vi "LS Durability Main (RT).vi"() -> ()   [LabVIEW 2013]
uses:
  Type Defs/App Config.ctl
  Type Defs/Controller Names.ctl
  SubVIs/Data Logger/Data Log Init.ctl
  Controls/Alarm Config.ctl
  Controls/Alarm Definition.ctl
  Controls/Alarm Profile Config.ctl
  Type Defs/Controller List.ctl
  Controls/Tank CMDs.ctl
  Controls/Controller Config.ctl
  Controls/Pump Data.ctl
  Controls/Tank Data.ctl
  Controls/HMI Cluster.ctl
  Controls/HMI Header.ctl
  Controls/HMI Tog Buttons.ctl
  Controls/HMI Mom Buttons.ctl
  Type Defs/LS Data.ctl
  Type Defs/Sequence States.ctl
  Controls/App Global Mode.ctl
  Controls/RPi HMI Mode.ctl
  Controls/Email Mode.ctl
  Type Defs/Pump Data Mode.ctl
  SubVIs/Watlow Modbus/Modbus Mode.ctl
  SubVIs/Watlow Modbus/Modbus Variable.ctl
  Controls/HMI Global Mode.ctl
  <vilib>/FPGAPlugInAG/sbRIO-9626/niLvFpga_Open_sbRIO-9626.vi
  <vilib>/Utility/error.llb/Error Cluster From Error Code.vi
  <vilib>/rvi/errors/niLvFpgaAdjustHostInterfaceError.vi
  <vilib>/Utility/file.llb/Write To Spreadsheet File (string).vi
  <vilib>/rvi/interface/nirviOpenFPGA/nirviOpenFPGA.xnode
  Controls/FPGA_Reference.ctl
  FPGA Bitfiles/LSDurability_Main.lvbitx
  <vilib>/rvi/interface/nirviReadWriteControl/nirviReadWriteControl.xnode
  <vilib>/Utility/config.llb/NI_LVConfig.lvlib
  Controls/Power Supply Global Mode.ctl
  SubVIs/Data Logger/Data Logger Mode.ctl
  SubVIs/Data Logger/Data Log Start.ctl
  <vilib>/rvi/errors/niLvFpgaMergeErrorWithErrorCode.vi
  NiFpgaLv.dll
panel:
  in  "pb.Run Profile":bool
  in  "Bank 2":T1={"7"=TRUE, "8"=TRUE, "9"=TRUE, "10"=TRUE, "11"=TRUE}
  in  "Bank 1":T2={"1"=TRUE, "2"=TRUE, "3"=TRUE, "4"=TRUE, "5"=TRUE} caption="Present"
  out "Email Alarms Disabled":bool
  out "Recording":bool
  in  "Disable Alarm Email":bool
  in  "Temp Tolerance":dbl=3.0 min=0.0 max=999999.0 step=1.0
  in  "Thermocouple":enum16{"2 TC/2 Tanks", "1 TC/1 Tank"}(ring)
  out "ADC Errors":i32
  in  "pb.Tare Pressure":bool
  in  "Data Log Enabled":bool=TRUE
  in  "RPMhyst":fxp<+,25,6>=1.0
  in  "pb.FuelChange":bool
  in  "Controller Type:":T3
  in  "Target Pressure:":dbl
  in  "Target Voltage:":dbl
  in  "Tank 1 Fuel Type:":string
  in  "Tank 2 Fuel Type:":string
  in  "Stagger Time (ms):":i32
  out "Cycles Completed:":u32=17
  in  "pb.Cycle Reset":bool
  in  "Serial Numbers":T4
  out "Read Inputs (ms)":u32
  out "Update Screen (ms)":u32
  out "Run Step (ms)":u32
  in  "Fuel Change Tab":enum32{"Page 1", "Page 2"}(tab)
  in  "pb.Fuel Change OK":bool
  in  "Reset Tab":enum32{"Page 1", "Page 2"}(tab)
  in  "pb.Reset OK":bool
  in  "pb.Reset Cancel":bool
  in  "Save As Tab":enum32{"Page 1", "Page 2"}(tab)
  in  "New Profile Name:":string
  in  "pb.Save As OK":bool
  in  "pb.Save As Cancel":bool
  in  "Alarm Tab":enum32{"Page 1", "Page 2"}(tab)
  out "Alarm Message":string
  in  "pb.Alarm OK":bool
  in  "Set Time Tab":enum32{"Page 1", "Page 2"}(tab)
  in  "pb.Set Time OK":bool
  in  "pb.Set Time Cancel":bool
  in  "New Time":dbl format="%<%H:%M:%S>t"
  in  "Pump Timers Tab":enum32{"Page 1", "Page 2"}(tab)=enum."Page 2"
  in  "Stop Time Enable":bool
  in  "Stop Time:":dbl format="%<%H:%M:%S>t"
  in  "pb.Time Reset All":bool
  out "Elapsed Time:":dbl[](array[numeric]) format="%<%H:%M:%S>t"
  in  "pb.Resets":bool[](array[boolean])=[FALSE, FALSE, FALSE, FALSE, FALSE, FALSE]
  in  "pb.Sets":bool[](array[boolean])=[FALSE, FALSE, FALSE, FALSE, FALSE, FALSE]
  in  "LS Serial Numbers":T5 caption="Serial Numbers"
  out "CPU Usage:":dbl=7.74131899555212 format="%.1f"
  in  "Live Data Tab":enum32{"Page 1", "Page 2", "Page 3"}(tab)=enum."Page 2"
  in  "Controller\nCMD":dbl[](array[numeric])=[0.0, 0.0, 0.0, 0.0, 0.0, 0.0] format="%#.2f"
  out "Speed":dbl[](array[numeric]) caption="Speed\n(RPM)" format="%#.0f"
  out "ControllerCurrent":dbl[](array[numeric])=[0.015201568603515625, 0.00335693359375, 0.003021240234375, 0.12260055541992188, 0.06085968017578125, 0.052234649658203125] caption="Controller\nCurrent\n(DC)" format="%.1f"
  out "PumpCurrent":dbl[](array[numeric])=[0.015201568603515625, 0.00335693359375, 0.003021240234375, 0.12260055541992188, 0.06085968017578125, 0.052234649658203125] caption="Pump\nCurrent\n(RMS)" format="%.1f"
  out "Flow":dbl[](array[numeric])=[0.0, 0.0, 0.0, 0.125, 0.0625, 0.0625] caption="Flow\n(L/H)" format="%#.0f"
  out "Pressure":dbl[](array[numeric])=[0.015201568603515625, 0.00335693359375, 0.003021240234375, 0.12260055541992188, 0.06085968017578125, 0.052234649658203125] caption="Pressure\n(kPa)" format="%#.0f"
  out "Ave. Speed":dbl=7.74131899555212 format="%.1f"
  out "Voltages":dbl[](array[numeric])=[0.015201568603515625, 0.00335693359375, 0.003021240234375, 0.12260055541992188, 0.06085968017578125, 0.052234649658203125] caption="Pump\nVoltage\n(V)" format="%.1f"
  in  "Reset Anomalies":bool
  in  "Reset Total Cycles":bool
  out "Anomalies (Last Cycle)":i32[](array[numeric]) caption="Anomalies\n(Last Cycle)" format="%#.0f"
  out "Anomalies/Cycle":i32[](array[numeric]) caption="Anomalies/\nCycle" format="%#.0f"
  out "Cycles":u32[](array[numeric]) format="%#.0f"
  out "Anomalies Total":i32[](array[numeric]) caption="Anomalies\nTotal" format="%#.0f"
  out "Steps":u32[](array[numeric]) format="%#.0f"
  out "Total Cycles":u32[](array[numeric]) caption="Total\nCycles" format="%#.0f"
  in  "Reset Opens":bool
  out "Opens":i32[](array[numeric]) format="%#.0f"
  in  "App Config":T6={"Location"="Tanks 162-163", "Profiles Path"=path "c:/Profiles", "Current Profile"="", "CA Number"="", "Cycles Completed"=0, "Controller Type:"=enum."Kuhnke", "Stagger Time (ms)"=0, "Tank 1 Fuel"="", "Tank 2 Fuel"="", "Serial Numbers"={"Position 1 SN"="", "Position 2 SN"="", "Poaition 3 SN"="", "Position 4 SN"="", "Position 5 SN"="", "Position 6 SN"=""}, "Pumps Present"={"Pump 1"=FALSE, "Pump 2"=FALSE, "Pump 3"=FALSE, "Pump 4"=FALSE, "Pump 5"=FALSE, "Pump 6"=FALSE}, "VoltCtrlRef"="", "VoltageSelect"=FALSE, "Watlow Present"=TRUE, "Temp 1"=0.0, "Temp 2"=0.0, "V_Run PI?"=FALSE, "Voltage Limits"={"V_Step"=1e-05, "V_CmdMax"=0.0, "V_CmdMin"=0.0}, "Voltage Far PI"={"V_FarSlew"=10.0, "V_FarKp"=0.0, "V_FarKi"=0.0}, "Voltage Mid PI"={"V_MidSlew"=10.0, "V_MidKp"=0.0, "V_MidKi"=0.0}, "Voltage Close PI"={"V_CloseSlew"=10.0, "V_CloseKp"=0.0, "V_CloseKi"=0.0}, "Voltage Scale"={"V_FFm"=0.0, "V_FFb"=0.0}, "Voltage Cutoffs"={"V_MidCutoff"=0.0, "V_CloseCutoff"=0.0}, "Pressure Scale"={"Pres_FFm"=1e-05, "Pres_FFb"=0.0}, "Temp Format"=0, "Temp Tolerance"=0.0, "Target Voltage"=0.0, "Target Pressure"=0.0, "Data Log Init"={"Data Path"=path "u:/Data", "Data Log Rate (S/s)"=1, "AKLH Rate (Hours/S)"=0.1, "Sync Time Offset (min)"=180, "IP Last 3"=0, "WebDAV IP"="10.31.176.36"}, "Email Handler IP"="10.30.189.34", "ADC Check"=FALSE, "3 Pump Tank"=TRUE, "Cycle Threshold:"=3.0, "Cycle Pts to Avg:"=3, "Anomaly Threshold:"=3.0, "Normal Steps:"=3, "Step Threshold:"=3.0} {"Step Threshold:" min=0.0 max=999999.0 step=1.0; "Normal Steps:" max=999999 step=1; "Anomaly Threshold:" min=0.0 max=999999.0 step=1.0; "Cycle Pts to Avg:" max=999999 step=1; "Cycle Threshold:" min=0.0 max=999999.0 step=1.0}
  in  "Monitoring Tab":enum32{"Page 1", "Page 2"}(tab)
  out "Avg Press:":dbl=7.74131899555212
  in  "pb.E Stop":bool
  in  "Ignition Relay":T8
  in  "Power Relay":T8
  out "Temp2":dbl caption="Tank 2 Temp (C):" format="%.1f"
  out "Temp1":dbl caption="Tank 1 Temp (C):" format="%.1f"
  out "PS Actual (V):":dbl format="%.2f"
  in  "Power Supply Cmd:":dbl min=0.0 max=20.0 format="%#.2f"
  in  "PressureCMD":dbl caption="Pressure Cmd:" min=0.0 max=825.0 format="%#.2f"
  in  "Pumps Present":T8={"Pump 1"=TRUE, "Pump 2"=TRUE, "Pump 3"=TRUE, "Pump 4"=TRUE, "Pump 5"=TRUE, "Pump 6"=TRUE}
  in  "Tank 1 Temp Cmd:":dbl caption="deg C"
  in  "Tank 2 Temp Cmd:":dbl caption="deg C"
  in  "Title Tab":enum32{"Page 1", "Page 2"}(tab)
  in  "Title":string="LS Durability Tester, v1.5"
  out "Time/Date":string
  in  "Login":bool
  in  "pb.Stop Profile":bool
  in  "Main Tab":T9(tab)
  in  "pb.Pause/Resume":bool
  out "Transferring":bool
  in  "Recording\nFrequency (Hz): 2":i32=1000
  in  "Recording\nDuration (s): 2":i32=3600
  in  "Record Constant":bool
  in  "Detection Mode:":u16(ring) items=["Anomalies", "Opens"]
  in  "Record During Profile":bool
  in  "Recording\nFrequency (Hz):":i32=1000
  in  "Recording\nDuration (s):":i32=10
  in  "Interval Between\nRecordings (s):":i32=600
  in  "LS Cycle Time (ms):":dbl=244.0 min=0.1 max=1000.0 step=0.1
  in  "LS On Time (ms):":dbl=4.0 min=0.0 max=1000.0 step=0.01
  in  "Bank 2 Power State:":u16(ring) items=["0 - Off", "1 - On", "2 - Pulsing"]
  in  "Bank 1 Power State:":u16(ring) items=["0 - Off", "1 - On", "2 - Pulsing"]
  in  "CA Number:":string
  in  "Profile Name:":string(combo)="test"
  in  "pb.Save As":bool
  out "Location:":string
  in  "Profile:":string[][](table)=[["1", "216000", "1", "2", "244", "4", "1", "67.6"], ["2", "1800", "0", "0", "244", "4", "1", "10.0"], ["3", "39600", "0", "0", "244", "4", "0", ""], ["4", "1800", "0", "0", "244", "4", "1", ""]]
  out "Recording":bool
  in  "Data File Name:":string
  out "Step:":i32=2
  out "Time Left:":dbl=0.21101045608520508
  out "Waveform Chart":dbl(graph)
  in  "Pause":bool
  in  "Position":i32=1 min=1 max=10 step=1
  in  "Voltage(T)/Resistance(F)":bool=TRUE
  in  "Bias Resistances":dbl[](array[numeric])=[681.0, 681.0, 681.0, 681.0, 681.0, 681.0, 681.0, 681.0, 681.0, 681.0, 681.0, 681.0] caption="Total\nCycles"
  in  "Subtract Noise":bool
  in  "Anomaly Threshold:":dbl=3.0 min=0.0 max=999999.0 step=1.0
  in  "Normal Steps:":u32=3 max=999999 step=1
  in  "Step Threshold:":dbl=3.0 min=0.0 max=999999.0 step=1.0
  in  "Cycle Pts to Avg:":i32=3 min=0 max=999999 step=1
  in  "Cycle Threshold:":dbl=3.0 min=0.0 max=999999.0 step=1.0
  in  "Note Tab":enum32{"Page 1", "Page 2"}(tab)
  in  "Stop Profile Note":string
  in  "pb.Note OK":bool
  in  "pb.Note Cancel":bool
  in  "Second Step Check":bool
  in  "Alarm Config":T10
  in  "WebDAV Push":bool
  in  "Concat Data":bool
  in  "Cutoffs":cluster{"Mid Range":dbl, "Close Range":dbl} {"Close Range" min=-100000.0 max=100000.0 step=1e-05 format="%#.5f"; "Mid Range" min=-100000.0 max=100000.0 step=1e-05 format="%#.5f"}
  in  "Mid PI":cluster{"Slew Rate":dbl, "Kp":dbl, "Ki":dbl}={"Slew Rate"=10.0, "Kp"=0.0, "Ki"=0.0} {"Ki" min=-100000.0 max=100000.0 step=1e-05 format="%#.5f"; "Kp" min=-100000.0 max=100000.0 step=1e-05 format="%#.5f"; "Slew Rate" min=0.0 max=1000000.0 step=0.01 format="%#.5f"}
  in  "Close PI":cluster{"Slew Rate":dbl, "Kp":dbl, "Ki":dbl}={"Slew Rate"=10.0, "Kp"=0.0, "Ki"=0.0} {"Ki" min=-100000.0 max=100000.0 step=1e-05 format="%#.5f"; "Kp" min=-100000.0 max=100000.0 step=1e-05 format="%#.5f"; "Slew Rate" min=0.0 max=1000000.0 step=0.01 format="%#.5f"}
  in  "Pressure Scale":cluster{"M":dbl, "B":dbl}={"M"=1e-05, "B"=0.0} {"B" min=-100000.0 max=100000.0 step=1e-05 format="%#.5f"; "M" min=-100000.0 max=100000.0 step=1e-05 format="%#.5f"}
  in  "Closed Loop Voltage":bool
  in  "Voltage Limits":cluster{"Step":dbl, "Max":dbl, "Min":dbl}={"Step"=1e-05, "Max"=0.0, "Min"=0.0} {"Min" min=0.0 max=10.0 step=1e-05 format="%#.5f"; "Max" min=0.0 max=10.0 step=1e-05 format="%#.5f"; "Step" min=0.0 max=100.0 step=1e-05 format="%#.5f"}
  in  "Far PI":cluster{"Slew Rate":dbl, "Kp":dbl, "Ki":dbl}={"Slew Rate"=10.0, "Kp"=0.0, "Ki"=0.0} {"Ki" min=-100000.0 max=100000.0 step=1e-05 format="%#.5f"; "Kp" min=-100000.0 max=100000.0 step=1e-05 format="%#.5f"; "Slew Rate" min=0.0 max=1000000.0 step=0.01 format="%#.5f"}
  in  "Voltage Scale":cluster{"M":dbl, "B":dbl} {"B" min=-100000.0 max=100000.0 step=1e-05 format="%#.5f"; "M" min=-100000.0 max=100000.0 step=1e-05 format="%#.5f"}
  # "Fuel Change was logged."
  # "Are you sure you want to reset?"
  # "Enter a new elapsed time."
  # "Pump Timers"
  # "Live Data"
  # "Level Sensor Monitor"
  # "Level Sensor Monitor"
  # "Manual Control"
  # "V"
  # "kPa"
  # "degC"
  # "degC"
  # "Data file note as to reason for stopping profile:"
  # "Voltage Control"
  # "Pressure Control"
  # "Data Server"
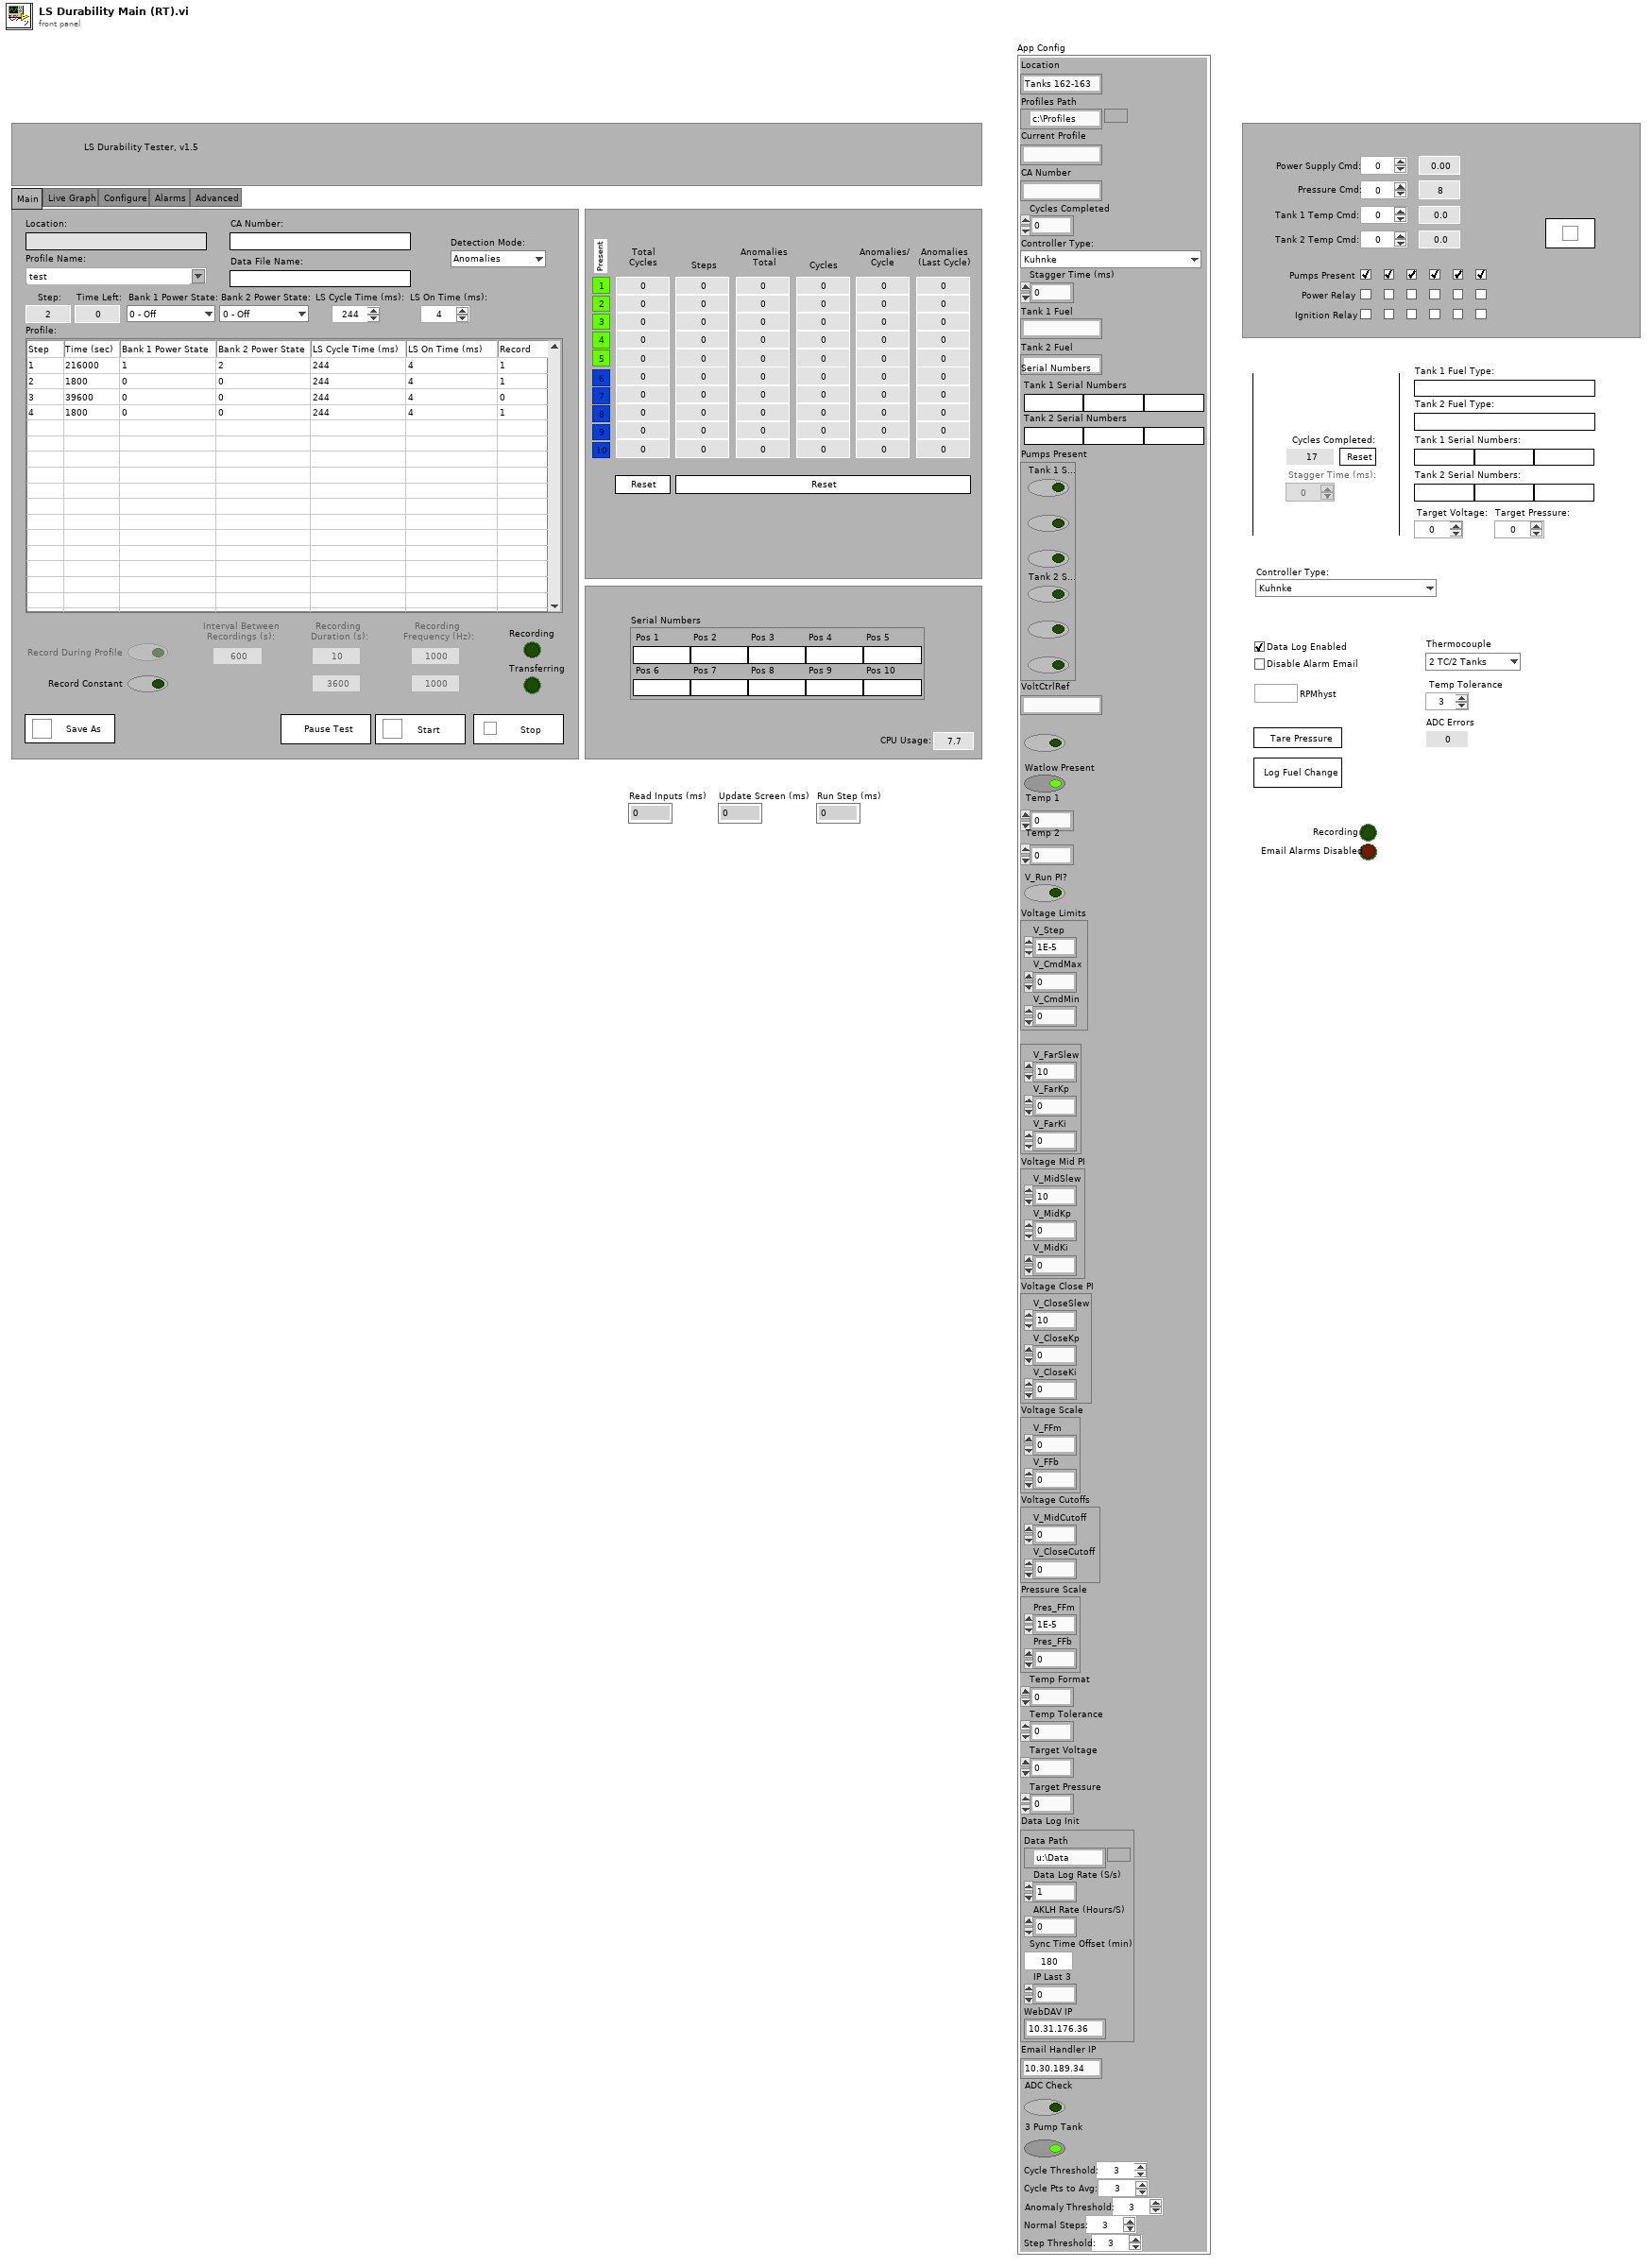
[diagram p1: front panel]
types:
  T1 = cluster{"7":bool, "8":bool, "9":bool, "10":bool, "11":bool}
  T2 = cluster{"1":bool, "2":bool, "3":bool, "4":bool, "5":bool}
  T3 = typedef "Controller Names.ctl" = enum16{"Kuhnke", "Helbako BLDC", "Conti", "Hella BLDC OL PWM", "Hella BLDC Turbine OL PWM", "Hella BLDC Pressure", "Helbako (old)", "TI PWM", "PSA", "Hella Gas", "Hella Diesel", "8 Comm", "10 Comm", "8 Comm Hella", "10 Comm Hella", "8 Comm Omron", "10 Comm Omron", "8 Comm Nissan", "10 Comm Nissan"}
  T4 = cluster{"Position 1 SN":string, "Position 2 SN":string, "Position 3 SN":string, "Position 4 SN":string, "Position 5 SN":string, "Position 6 SN":string}
  T5 = cluster{"Pos 1":string, "Pos 2":string, "Pos 3":string, "Pos 4":string, "Pos 5":string, "Pos 6":string, "Pos 7":string, "Pos 8":string, "Pos 9":string, "Pos 10":string}
  T6 = typedef "App Config.ctl" = cluster{"Location":string, "Profiles Path":path, "Current Profile":string, "CA Number":string, "Cycles Completed":u32, "Controller Type:":T3, "Stagger Time (ms)":i32, "Tank 1 Fuel":string, "Tank 2 Fuel":string, "Serial Numbers":cluster{"Position 1 SN":string, "Position 2 SN":string, "Poaition 3 SN":string, "Position 4 SN":string, "Position 5 SN":string, "Position 6 SN":string}, "Pumps Present":cluster{"Pump 1":bool, "Pump 2":bool, "Pump 3":bool, "Pump 4":bool, "Pump 5":bool, "Pump 6":bool}, "VoltCtrlRef":string, "VoltageSelect":bool, "Watlow Present":bool, "Temp 1":dbl, "Temp 2":dbl, "V_Run PI?":bool, "Voltage Limits":cluster{"V_Step":dbl, "V_CmdMax":dbl, "V_CmdMin":dbl}, "Voltage Far PI":cluster{"V_FarSlew":dbl, "V_FarKp":dbl, "V_FarKi":dbl}, "Voltage Mid PI":cluster{"V_MidSlew":dbl, "V_MidKp":dbl, "V_MidKi":dbl}, "Voltage Close PI":cluster{"V_CloseSlew":dbl, "V_CloseKp":dbl, "V_CloseKi":dbl}, "Voltage Scale":cluster{"V_FFm":dbl, "V_FFb":dbl}, "Voltage Cutoffs":cluster{"V_MidCutoff":dbl, "V_CloseCutoff":dbl}, "Pressure Scale":cluster{"Pres_FFm":dbl, "Pres_FFb":dbl}, "Temp Format":i32, "Temp Tolerance":dbl, "Target Voltage":dbl, "Target Pressure":dbl, "Data Log Init":T7, "Email Handler IP":string, "ADC Check":bool, "3 Pump Tank":bool, "Cycle Threshold:":dbl, "Cycle Pts to Avg:":i32, "Anomaly Threshold:":dbl, "Normal Steps:":u32, "Step Threshold:":dbl}
  T7 = typedef "Data Log Init.ctl" = cluster{"Data Path":path, "Data Log Rate (S/s)":u32, "AKLH Rate (Hours/S)":dbl, "Sync Time Offset (min)":i32, "IP Last 3":i32, "WebDAV IP":string}
  T8 = cluster{"Pump 1":bool, "Pump 2":bool, "Pump 3":bool, "Pump 4":bool, "Pump 5":bool, "Pump 6":bool}
  T9 = enum32{"Main", "Live Graph", "Configure", "Alarms", "Advanced"}
  T10 = typedef "Alarm Config.ctl" = cluster{"Alarms:":T11[], "Profile Sync:":T12}
  T11 = typedef "Alarm Definition.ctl" = cluster{"Description:":string, "Enabled:":bool, "Data Index:":i32, "Data Type:":string, "Low Limit:":dbl, "High Limit:":dbl, "Trip Time:":u32, "Profile Sync:":bool}
  T12 = typedef "Alarm Profile Config.ctl" = cluster{"Trip Time:":u32, "Consecutive Trips:":i32}
  T13 = cluster{"LS Power (Freq):":dbl, "LS Power (Duty):":dbl, "Bank 1 Present":cluster{"1":bool, "2":bool, "3":bool, "4":bool, "5":bool}, "Bank 2 Present":cluster{"7":bool, "8":bool, "9":bool, "10":bool, "11":bool}, "Data File Name:":string, "Record Bursts":bool, "RecInterval(s)":i32, "RecDuration(s)":i32, "RecFrequeny (Hz)":i32, "DetectionMode":i32, "Serial Numbers":string[], "Record Constant":bool, "2nd Step Check":bool, "Bias Resistances":dbl[], "Voltage(T)/Resistance(F)":bool}
  T14 = typedef "Sequence States.ctl" = enum16{"Main", "Init Files", "Init", "Unused", "Save As", "Start Profile", "Check Step Time", "Alarm", "Alarm Dismiss", "Run Step", "Stop Profile", "Cycle Reset", "Time Reset", "Time Reset All", "Time Set", "Tare CTs", "Save Profile", "Open Profile", "Get Profiles", "Update Screen", "Update Controls", "Save App Config", "Write Outputs", "Disable Background", "Enable Background", "Get/Release Control", "Log Fuel Change", "Fuel Change Popup", "Read Inputs", "Remote Timer Reset", "Controller Change", "Get Alarms", "Init Alarms", "Save Alarms", "Voltage Selection", "Set Watlow Temp 1", "Set Watlow Temp 2", "Get Pressure", "Write Tare Pressure", "Adjust Controls", "Reinit ADC", "Write Initial Times", "Write Pumps Present", "HMI Command", "Save Pump Times", "Check Pump Stop Time", "Save LS App Config", "Init Data File", "Reset LS Cycles", "Reset Anomalies", "Reset Opens", "Save LS Data", "Save LS Test Data", "Check Serial Numbers", "Main Tab", "Allow Data Note", "Resume Profile"}
  T15 = typedef "LS Data.ctl" = cluster{"Total Cycles":u32[], "Steps":u32[], "Anomalies Total":i32[], "Cycles":u32[], "Anomalies/Cycle":i32[], "Anomalies (Last Cycle)":i32[], "Opens":i32[]}
  T16 = typedef "HMI Cluster.ctl" = cluster{"Error":errorcluster, "COM Ref":refnum<visa-resource-name>, "Pump Data":T17, "Tank Data":cluster{"PS Actual (V):":dbl, "Temp1":dbl, "Temp2":dbl}, "Power Relays":cluster{"Pump 1":bool, "Pump 2":bool, "Pump 3":bool, "Pump 4":bool, "Pump 5":bool, "Pump 6":bool}, "Pump CMDs":dbl[], "HMI Header":T18, "Tank CMDs":T19, "HMI Tog Buttons":T20, "In Test":bool, "HMI Command":bool, "HMI Mom Buttons":T21, "Controller Config":T22, "Alarm":bool, "Alarm Message 1":string, "Alarm Message 2":string, "Recording":bool, "Serial Numbers":string[], "Pumps Present":bool[]}
  T17 = typedef "Pump Data.ctl" = cluster{"Voltages":dbl[], "PumpCurrent":dbl[], "Speed":dbl[], "ControllerCurrent":dbl[], "Pressure":dbl[], "Flow":dbl[], "Elapsed Time (Display)":dbl[], "Avg Pressure":dbl, "Avg Speed":dbl, "Elapsed Time":dbl[]}
  T18 = typedef "HMI Header.ctl" = cluster{"Line 1":string, "Line 2":string, "Line 3":string, "Line 4":string}
  T19 = typedef "Tank CMDs.ctl" = cluster{"PS CMD":dbl, "Press CMD":dbl, "Temp 1 CMD":dbl, "Temp 2 CMD":dbl}
  T20 = typedef "HMI Tog Buttons.ctl" = cluster{"Start Test":bool, "Toggle Spare 1":bool, "Toggle Spare 2":bool, "Toggle Spare 3":bool, "Toggle Spare 4":bool, "Toggle Spare 5":bool}
  T21 = typedef "HMI Mom Buttons.ctl" = cluster{"Stop":bool, "Reset Timers":bool, "Log Fuel Change":bool, "Alarm Dismiss":bool}
  T22 = typedef "Controller Config.ctl" = cluster{"Controller Name":T3, "CommSeg":i32, "PWM?":bool, "Frequency":i32, "Low Command":dbl, "High Command":dbl, "Stop Command":dbl, "Command Step":dbl, "Solenoid Stop?":bool, "Controller?":bool, "Invert PWM":bool}
  T23 = typedef "Tank Data.ctl" = cluster{"PS Actual (V):":dbl, "Temp1":dbl, "Temp2":dbl}
  T24 = typedef "Controller List.ctl" = cluster{"Controller Name":T3, "CommSeg":i32, "PWM?":bool, "Frequency":i32, "Low Command":dbl, "High Command":dbl, "Stop Command":dbl, "Command Step":dbl, "Solenoid Stop?":bool, "Controller?":bool, "Invert PWM":bool}[]
  T25 = cluster{"Error":errorcluster, "Profile":string[][], "App Config":T6, "Profiles":string[], "Current Step":i32, "Step Time Left":dbl, "Run Profile":bool, "Step Start Time":dbl, "Step Time":dbl, " # of Steps":i32, "Screen Timer":u32, "Last Profile Time":dbl, "Controller CMDs":dbl[], "Client?":bool, "pb.Run Profile":bool, "pb.Resets":bool[], "pb.Sets":bool[], "Initial Times":dbl[], "Pressure Offsets":dbl[], "Login":bool, "Stagger Counter":i32, "New Step":bool, "Inputs Timer":u32, "Tank Data":T23, "Voltage Enable":bool, "Power Relay":cluster{"Pump 1":bool, "Pump 2":bool, "Pump 3":bool, "Pump 4":bool, "Pump 5":bool, "Pump 6":bool}, "Ignition Relay":cluster{"Pump 1":bool, "Pump 2":bool, "Pump 3":bool, "Pump 4":bool, "Pump 5":bool, "Pump 6":bool}, "Controller List":T24, "Alarm Config":T10, "Alarm Config Path":path, "Trip Counters":i32[], "Previous Times":u32[], "Alarm Message 1":string, "Alarm Message 2":string, "Prev ON Times":u32[], "CalArray":dbl[][], "Tank CMDs":T19, "Controller Config":T22, "Fuel Log Path":path, "Pump Data":T17, "Alarm Latch":bool, "Time/Date":string, "Recording":bool, "HMI":T16, "WebDAV Push":bool, "Email Alarms Disabled":bool, "Concat Data":bool, "LS Data":T15, "Main Tab":enum32{"Main", "Live Graph", "Configure", "Alarms", "Advanced"}, "LS App Config":cluster{"LS Power (Freq):":dbl, "LS Power (Duty):":dbl, "Bank 1 Present":cluster{"1":bool, "2":bool, "3":bool, "4":bool, "5":bool}, "Bank 2 Present":cluster{"7":bool, "8":bool, "9":bool, "10":bool, "11":bool}, "Data File Name:":string, "Record Bursts":bool, "RecInterval(s)":i32, "RecDuration(s)":i32, "RecFrequeny (Hz)":i32, "DetectionMode":i32, "Serial Numbers":string[], "Record Constant":bool, "2nd Step Check":bool, "Bias Resistances":dbl[], "Voltage(T)/Resistance(F)":bool}, "Bank 1 State:":u16, "Bank 2 State:":u16, "LS Data Filepath":path, "Initial LS Data":T15, "day of month":i32, "Pause Test":bool}
  T26 = typedef "FPGA_Reference.ctl" = refnum<k20>
  T27 = typedef "App Global Mode.ctl" = enum16{"Read", "Write Client", "Write Login"}
  T28 = typedef "Data Logger Mode.ctl" = enum16{"Init", "Main", "Start", "Stop"}
  T29 = cluster{"Running?":bool, "Profile Record":bool, "RecordInterval":i32, "RecordDuration":i32, "RecordFreq":i32, "Data Filepath":path, "Hr Record":bool, "Serial Numbers":string[]}
  T30 = enum8{"Enabled", "Disabled", "Disabled and Grayed Out"}
  T31 = enum16{"open", "replace", "create", "open or create", "replace or create", "replace or create with confirmation"}
  T32 = typedef "Data Log Start.ctl" = cluster{"App Config":T6, "Profile":string[][], "Controller Type":string, "Tank CMDs":T19}
  T33 = typedef "Power Supply Global Mode.ctl" = enum16{"Write Setpoint", "Write FreezePID", "Read"}
  T34 = typedef "RPi HMI Mode.ctl" = enum16{"Init", "Write Data", "Read from RPi", "Write to RPi"}
  T35 = typedef "Email Mode.ctl" = enum16{"Trigger Email", "Send Email"}
  T36 = typedef "Pump Data Mode.ctl" = enum16{"Read", "Write Data", "Write Cal", "Write Watlow Data", "Write Pressure Offsets", "Write Initial Times", "Write Pumps Present"}
  T37 = typedef "Modbus Variable.ctl" = enum16{"Temperature", "Setpoint"}
  T38 = typedef "Modbus Mode.ctl" = enum16{"Init", "Tank 1 Write", "Tank 2 Write", "Tank 1 Read", "Tank 2 Read"}
  T39 = typedef "HMI Global Mode.ctl" = enum16{"Read", "Write Cluster", "Reset Cmd"}
  T40 = cluster{"Position 1 SN":string, "Position 2 SN":string, "Poaition 3 SN":string, "Position 4 SN":string, "Position 5 SN":string, "Position 6 SN":string}
  T41 = cluster{"V_Step":dbl, "V_CmdMax":dbl, "V_CmdMin":dbl}
  T42 = cluster{"V_FarSlew":dbl, "V_FarKp":dbl, "V_FarKi":dbl}
  T43 = cluster{"V_MidSlew":dbl, "V_MidKp":dbl, "V_MidKi":dbl}
  T44 = cluster{"V_CloseSlew":dbl, "V_CloseKp":dbl, "V_CloseKi":dbl}
  T45 = typedef "LVDateTimeRec.ctl" = cluster{"fractional second":dbl, "second":i32, "minute":i32, "hour":i32, "day of month":i32, "month":i32, "year":i32, "day of week":i32, "day of year":i32, "DST":i32}
  T46 = typedef "NI_LVConfig.lvlib/Config Data RefNum.ctl" = refnum<k1>
  T47 = cluster{"LS Power (Freq):":dbl, "LS Power (Duty):":dbl, "Bank 1 Present":cluster{"1":bool, "2":bool, "3":bool, "4":bool, "5":bool}, "Bank 2 Present":cluster{"6":bool, "7":bool, "8":bool, "9":bool, "10":bool}, "Data File Name:":string, "Record Bursts":bool, "RecInterval(s)":i32, "RecDuration(s)":i32, "RecFrequeny (Hz)":i32, "DetectionMode":i32, "Serial Numbers":string[], "Record Constant":bool, "2nd Step Check":bool, "Bias Resistances":dbl[], "Voltage(T)/Resistance(F)":bool}
  T48 = cluster{"Serial Numbers[0]":string, "Serial Numbers[1]":string, "Serial Numbers[2]":string, "Serial Numbers[3]":string, "Serial Numbers[4]":string, "Serial Numbers[5]":string, "Serial Numbers[6]":string, "Serial Numbers[7]":string, "Serial Numbers[8]":string, "Serial Numbers[9]":string}
  T49 = cluster{"Controller Name":T3, "CommSeg":i32, "PWM?":bool, "Frequency":i32, "Low Command":dbl, "High Command":dbl, "Stop Command":dbl, "Command Step":dbl, "Solenoid Stop?":bool, "Controller?":bool, "Invert PWM":bool}
  T50 = cluster{"[0]":bool, "[1]":bool, "[2]":bool, "[3]":bool, "[4]":bool, "[5]":bool}
  T51 = cluster{"[0]":string, "[1]":string, "[2]":string, "[3]":string, "[4]":string, "[5]":string, "[6]":string, "[7]":string, "[8]":string, "[9]":string}
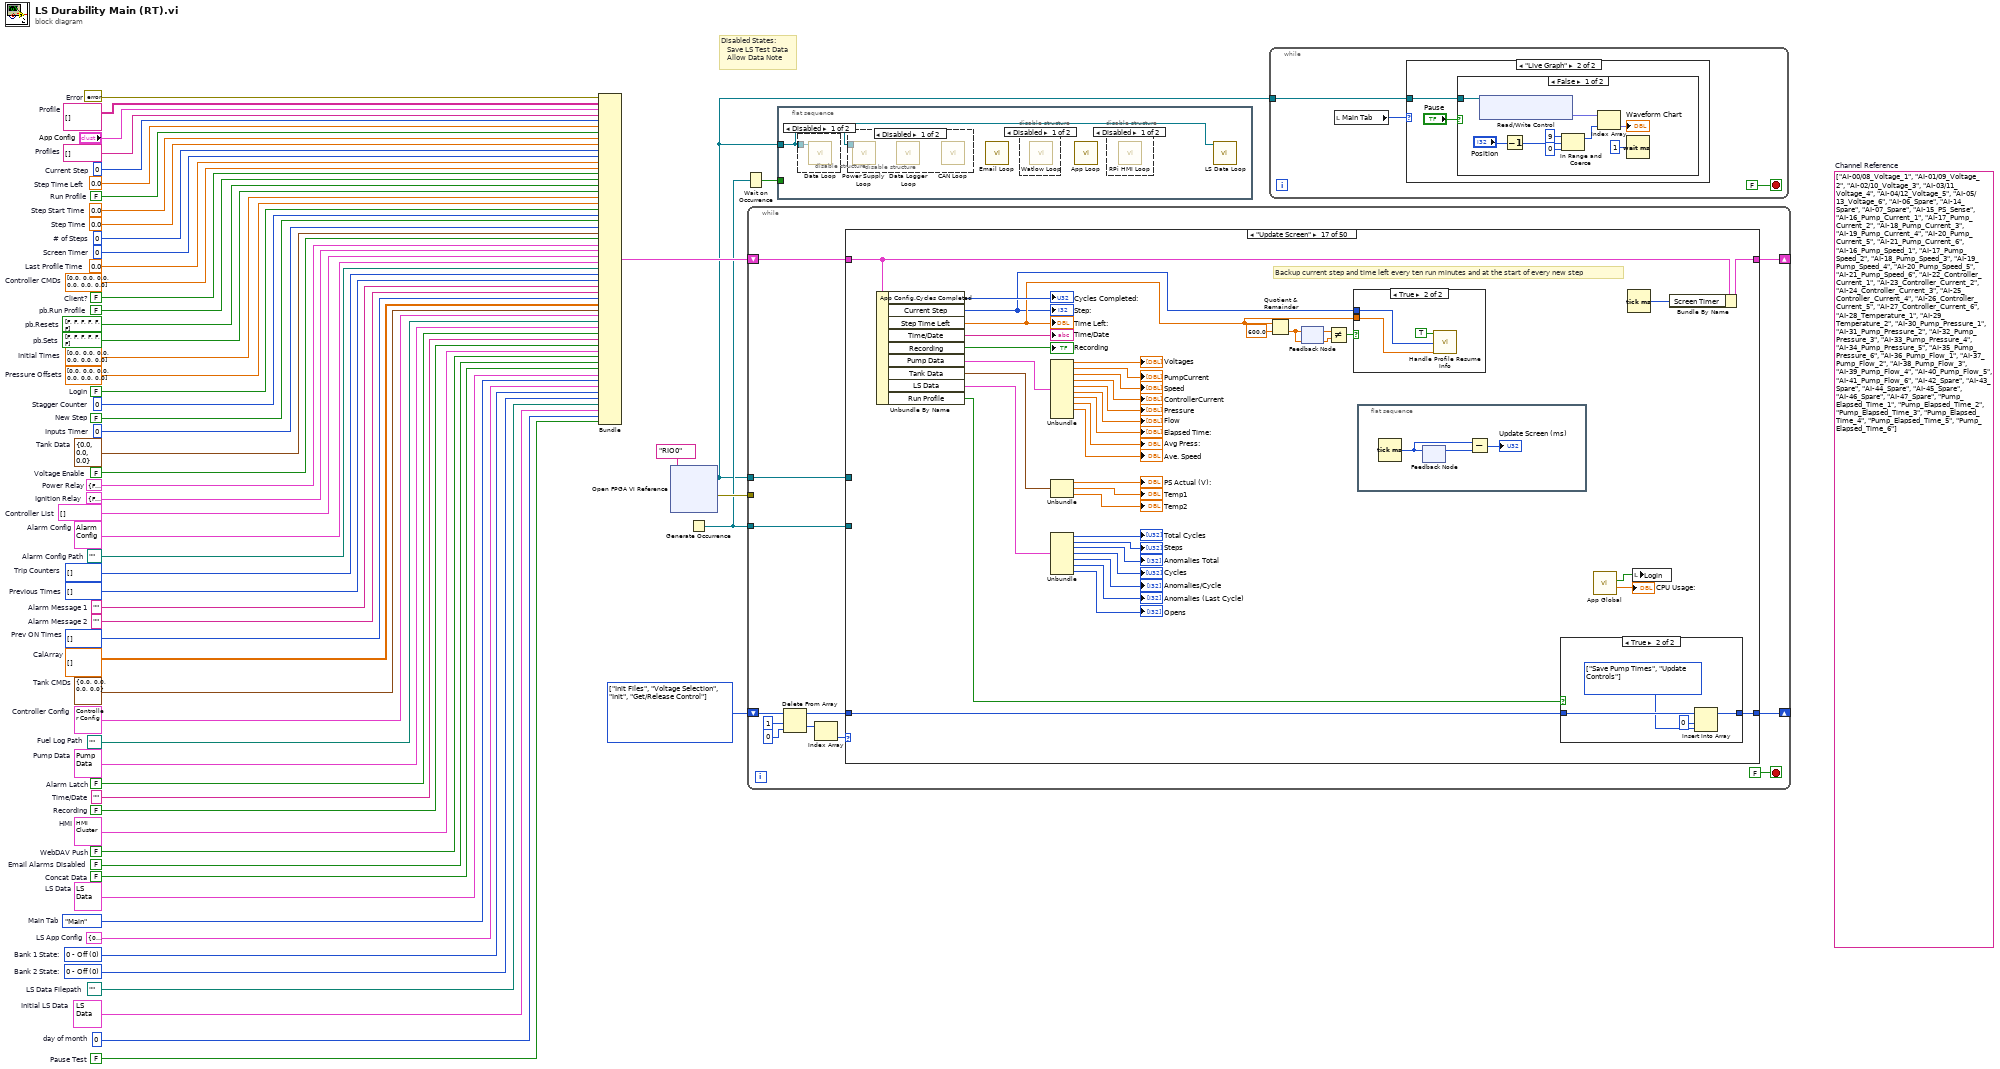
[diagram p0: block diagram]
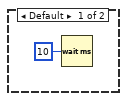
[diagram p2: hidden frame]
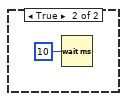
[diagram p3: hidden frame]
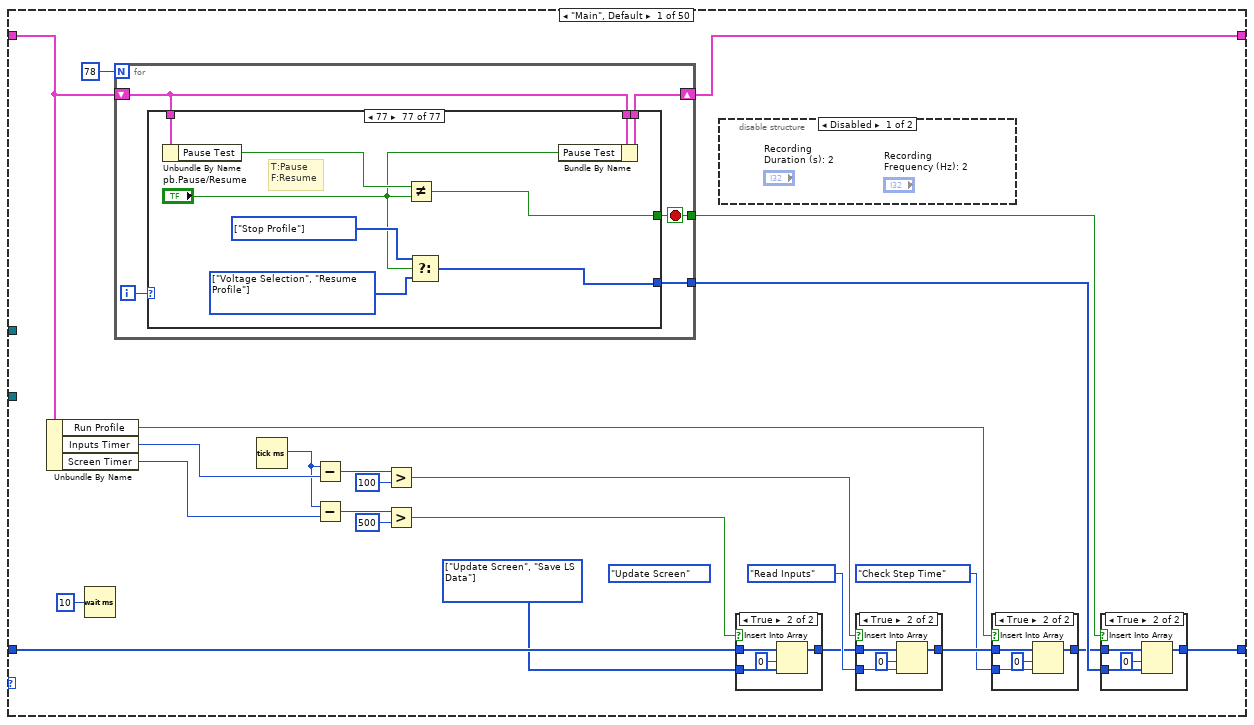
[diagram p8: hidden frame]
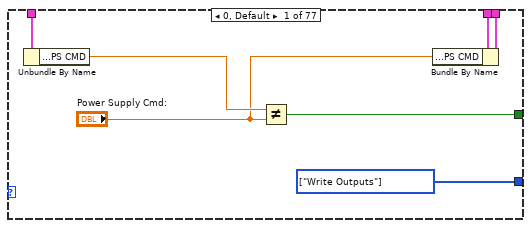
[diagram p14: hidden frame]
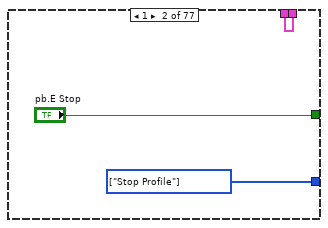
[diagram p15: hidden frame]
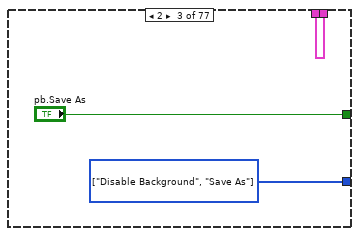
[diagram p16: hidden frame]
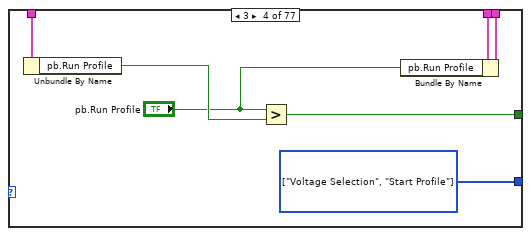
[diagram p17: hidden frame]
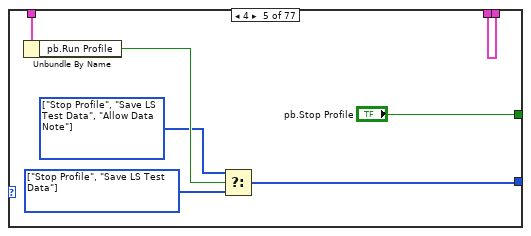
[diagram p18: hidden frame]
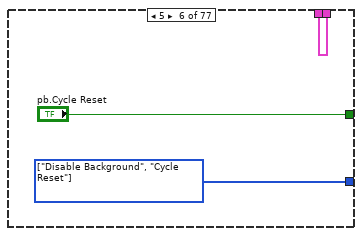
[diagram p19: hidden frame]
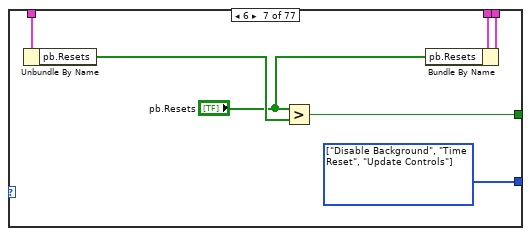
[diagram p20: hidden frame]
diagram:
  w1 = FALSE  # Pause Test
  w2 = T13 {"LS Power (Freq):"=0.0, "LS Power (Duty):"=0.0, "Bank 1 Present"={"1"=TRUE, "2"=TRUE, "3"=TRUE, "4"=TRUE, "5"=TRUE}, "Bank 2 Present"={"7"=TRUE, "8"=TRUE, "9"=TRUE, "10"=TRUE, "11"=TRUE}, "Data File Name:"="", "Record Bursts"=FALSE, "RecInterval(s)"=600, "RecDuration(s)"=10, "RecFrequeny (Hz)"=1000, "DetectionMode"=0, "Serial Numbers"=["", "", "", "", "", "", "", "", "", ""], "Record Constant"=FALSE, "2nd Step Check"=FALSE, "Bias Resistances"=[681.0, 681.0, 681.0, 681.0, 681.0, 681.0, 681.0, 681.0, 681.0, 681.0, 681.0, 681.0], "Voltage(T)/Resistance(F)"=TRUE}  # LS App Config
  w3 = 0  # day of month
  (unwired) string[] ["AI-00/08_Voltage_1", "AI-01/09_Voltage_2", "AI-02/10_Voltage_3", "AI-03/11_Voltage_4", "AI-04/12_Voltage_5", "AI-05/13_Voltage_6", "AI-06_Spare", "AI-14_Spare", "AI-07_Spare", "AI-15_PS_Sense", "AI-16_Pump_Current_1", "AI-17_Pump_Current_2", "AI-18_Pump_Current_3", "AI-19_Pump_Current_4", "AI-20_Pump_Current_5", "AI-21_Pump_Current_6", "AI-16_Pump_Speed_1", "AI-17_Pump_Speed_2", "AI-18_Pump_Speed_3", "AI-19_Pump_Speed_4", "AI-20_Pump_Speed_5", "AI-21_Pump_Speed_6", "AI-22_Controller_Current_1", "AI-23_Controller_Current_2", "AI-24_Controller_Current_3", "AI-25_Controller_Current_4", "AI-26_Controller_Current_5", "AI-27_Controller_Current_6", "AI-28_Temperature_1", "AI-29_Temperature_2", "AI-30_Pump_Pressure_1", "AI-31_Pump_Pressure_2", "AI-32_Pump_Pressure_3", "AI-33_Pump_Pressure_4", "AI-34_Pump_Pressure_5", "AI-35_Pump_Pressure_6", "AI-36_Pump_Flow_1", "AI-37_Pump_Flow_2", "AI-38_Pump_Flow_3", "AI-39_Pump_Flow_4", "AI-40_Pump_Flow_5", "AI-41_Pump_Flow_6", "AI-42_Spare", "AI-43_Spare", "AI-44_Spare", "AI-45_Spare", "AI-46_Spare", "AI-47_Spare", "Pump_Elapsed_Time_1", "Pump_Elapsed_Time_2", "Pump_Elapsed_Time_3", "Pump_Elapsed_Time_4", "Pump_Elapsed_Time_5", "Pump_Elapsed_Time_6"]  # Channel Reference
  w9 = T14[] [enum."Init Files", enum."Voltage Selection", enum."Init", enum."Get/Release Control"] items=["Main", "Init Files", "Init", "Unused", "Save As", "Start Profile", "Check Step Time", "Alarm", "Alarm Dismiss", "Run Step", "Stop Profile", "Cycle Reset", "Time Reset", "Time Reset All", "Time Set", "Tare CTs", "Save Profile", "Open Profile", "Get Profiles", "Update Screen", "Update Controls", "Save App Config", "Write Outputs", "Disable Background", "Enable Background", "Get/Release Control", "Log Fuel Change", "Fuel Change Popup", "Read Inputs", "Remote Timer Reset", "Controller Change", "Get Alarms", "Init Alarms", "Save Alarms", "Voltage Selection", "Set Watlow Temp 1", "Set Watlow Temp 2", "Get Pressure", "Write Tare Pressure", "Adjust Controls", "Reinit ADC", "Write Initial Times", "Write Pumps Present", "HMI Command", "Save Pump Times", "Check Pump Stop Time", "Save LS App Config", "Init Data File", "Reset LS Cycles", "Reset Anomalies", "Reset Opens", "Save LS Data", "Save LS Test Data", "Check Serial Numbers", "Main Tab", "Allow Data Note", "Resume Profile"]
  w10 = T15 {"Total Cycles"=[0, 0, 0, 0, 0, 0, 0, 0, 0, 0, 0, 0], "Steps"=[0, 0, 0, 0, 0, 0, 0, 0, 0, 0, 0, 0], "Anomalies Total"=[0, 0, 0, 0, 0, 0, 0, 0, 0, 0, 0, 0], "Cycles"=[0, 0, 0, 0, 0, 0, 0, 0, 0, 0, 0, 0], "Anomalies/Cycle"=[0, 0, 0, 0, 0, 0, 0, 0, 0, 0, 0, 0], "Anomalies (Last Cycle)"=[0, 0, 0, 0, 0, 0, 0, 0, 0, 0, 0, 0], "Opens"=[0, 0, 0, 0, 0, 0, 0, 0, 0, 0, 0, 0]}  # Initial LS Data
  w11 = path ""  # LS Data Filepath
  w13 = u16 0 items=["0 - Off", "1 - On", "2 - Pulsing"]  # Bank 1 State:
  w12 = u16 0 items=["0 - Off", "1 - On", "2 - Pulsing"]  # Bank 2 State:
  w14 = T9."Main"  # Main Tab
  w15 = T15 {"Total Cycles"=[0, 0, 0, 0, 0, 0, 0, 0, 0, 0, 0, 0], "Steps"=[0, 0, 0, 0, 0, 0, 0, 0, 0, 0, 0, 0], "Anomalies Total"=[0, 0, 0, 0, 0, 0, 0, 0, 0, 0, 0, 0], "Cycles"=[0, 0, 0, 0, 0, 0, 0, 0, 0, 0, 0, 0], "Anomalies/Cycle"=[0, 0, 0, 0, 0, 0, 0, 0, 0, 0, 0, 0], "Anomalies (Last Cycle)"=[0, 0, 0, 0, 0, 0, 0, 0, 0, 0, 0, 0], "Opens"=[]}  # LS Data
  w16 = FALSE  # Concat Data
  w17 = FALSE  # Email Alarms Disabled
  w18 = FALSE  # WebDAV Push
  w19 = T16 {"Error"={"status"=FALSE, "code"=0, "source"=""}, "COM Ref"="", "Pump Data"={"Voltages"=[], "PumpCurrent"=[], "Speed"=[], "ControllerCurrent"=[], "Pressure"=[], "Flow"=[], "Elapsed Time (Display)"=[], "Avg Pressure"=0.0, "Avg Speed"=0.0, "Elapsed Time"=[]}, "Tank Data"={"PS Actual (V):"=0.0, "Temp1"=0.0, "Temp2"=0.0}, "Power Relays"={"Pump 1"=FALSE, "Pump 2"=FALSE, "Pump 3"=FALSE, "Pump 4"=FALSE, "Pump 5"=FALSE, "Pump 6"=FALSE}, "Pump CMDs"=[], "HMI Header"={"Line 1"="", "Line 2"="", "Line 3"="", "Line 4"=""}, "Tank CMDs"={"PS CMD"=0.0, "Press CMD"=0.0, "Temp 1 CMD"=0.0, "Temp 2 CMD"=0.0}, "HMI Tog Buttons"={"Start Test"=FALSE, "Toggle Spare 1"=FALSE, "Toggle Spare 2"=FALSE, "Toggle Spare 3"=FALSE, "Toggle Spare 4"=FALSE, "Toggle Spare 5"=FALSE}, "In Test"=FALSE, "HMI Command"=FALSE, "HMI Mom Buttons"={"Stop"=FALSE, "Reset Timers"=FALSE, "Log Fuel Change"=FALSE, "Alarm Dismiss"=FALSE}, "Controller Config"={"Controller Name"=enum."Kuhnke", "CommSeg"=0, "PWM?"=FALSE, "Frequency"=0, "Low Command"=0.0, "High Command"=0.0, "Stop Command"=0.0, "Command Step"=0.0, "Solenoid Stop?"=FALSE, "Controller?"=FALSE, "Invert PWM"=FALSE}, "Alarm"=FALSE, "Alarm Message 1"="", "Alarm Message 2"="", "Recording"=FALSE, "Serial Numbers"=[], "Pumps Present"=[]}  # HMI
  w20 = T23 {"PS Actual (V):"=0.0, "Temp1"=0.0, "Temp2"=0.0}  # Tank Data
  w21 = FALSE  # Recording
  w22 = ""  # Time/Date
  w23 = ""  # Alarm Message 2
  w24 = FALSE  # Alarm Latch
  w25 = T17 {"Voltages"=[0.015201568603515625, 0.00335693359375, 0.003021240234375, 0.12260055541992188, 0.06085968017578125, 0.052234649658203125], "PumpCurrent"=[0.015201568603515625, 0.00335693359375, 0.003021240234375, 0.12260055541992188, 0.06085968017578125, 0.052234649658203125], "Speed"=[0.0, 0.0, 0.0, 0.0, 0.0, 0.0], "ControllerCurrent"=[0.015201568603515625, 0.00335693359375, 0.003021240234375, 0.12260055541992188, 0.06085968017578125, 0.052234649658203125], "Pressure"=[0.015201568603515625, 0.00335693359375, 0.003021240234375, 0.12260055541992188, 0.06085968017578125, 0.052234649658203125], "Flow"=[0.0, 0.0, 0.0, 0.125, 0.0625, 0.0625], "Elapsed Time (Display)"=[7.1, 7.1, 7.1, 458133.45, 458138.85000000003, 458126.75], "Avg Pressure"=0.0, "Avg Speed"=0.0, "Elapsed Time"=[]}  # Pump Data
  w26 = path ""  # Fuel Log Path
  w27 = T22 {"Controller Name"=enum."Kuhnke", "CommSeg"=0, "PWM?"=FALSE, "Frequency"=0, "Low Command"=0.0, "High Command"=0.0, "Stop Command"=0.0, "Command Step"=0.0, "Solenoid Stop?"=FALSE, "Controller?"=FALSE, "Invert PWM"=FALSE}  # Controller Config
  w28 = T19 {"PS CMD"=0.0, "Press CMD"=0.0, "Temp 1 CMD"=0.0, "Temp 2 CMD"=0.0}  # Tank CMDs
  w29 = dbl[][] []  # CalArray
  w30 = u32[] []  # Prev ON Times
  w31 = ""  # Alarm Message 1
  w32 = u32[] []  # Previous Times
  w33 = i32[] []  # Trip Counters
  w34 = path ""  # Alarm Config Path
  w35 = T10 {"Alarms:"=[{"Description:"="", "Enabled:"=FALSE, "Data Index:"=0, "Data Type:"="", "Low Limit:"=0.0, "High Limit:"=0.0, "Trip Time:"=0, "Profile Sync:"=FALSE}, {"Description:"="", "Enabled:"=FALSE, "Data Index:"=0, "Data Type:"="", "Low Limit:"=0.0, "High Limit:"=0.0, "Trip Time:"=0, "Profile Sync:"=FALSE}, {"Description:"="", "Enabled:"=FALSE, "Data Index:"=0, "Data Type:"="", "Low Limit:"=0.0, "High Limit:"=0.0, "Trip Time:"=0, "Profile Sync:"=FALSE}, {"Description:"="", "Enabled:"=FALSE, "Data Index:"=0, "Data Type:"="", "Low Limit:"=0.0, "High Limit:"=0.0, "Trip Time:"=0, "Profile Sync:"=FALSE}, {"Description:"="", "Enabled:"=FALSE, "Data Index:"=0, "Data Type:"="", "Low Limit:"=0.0, "High Limit:"=0.0, "Trip Time:"=0, "Profile Sync:"=FALSE}, {"Description:"="", "Enabled:"=FALSE, "Data Index:"=0, "Data Type:"="", "Low Limit:"=0.0, "High Limit:"=0.0, "Trip Time:"=0, "Profile Sync:"=FALSE}, {"Description:"="", "Enabled:"=FALSE, "Data Index:"=0, "Data Type:"="", "Low Limit:"=0.0, "High Limit:"=0.0, "Trip Time:"=0, "Profile Sync:"=FALSE}, {"Description:"="", "Enabled:"=FALSE, "Data Index:"=0, "Data Type:"="", "Low Limit:"=0.0, "High Limit:"=0.0, "Trip Time:"=0, "Profile Sync:"=FALSE}], "Profile Sync:"={"Trip Time:"=0, "Consecutive Trips:"=0}}  # Alarm Config
  w36 = T24 []  # Controller List
  w37 = T8 {"Pump 1"=FALSE, "Pump 2"=FALSE, "Pump 3"=FALSE, "Pump 4"=FALSE, "Pump 5"=FALSE, "Pump 6"=FALSE}  # Ignition Relay
  w38 = T8 {"Pump 1"=FALSE, "Pump 2"=FALSE, "Pump 3"=FALSE, "Pump 4"=FALSE, "Pump 5"=FALSE, "Pump 6"=FALSE}  # Power Relay
  w39 = FALSE  # Voltage Enable
  w40 = u32 0  # Inputs Timer
  w41 = dbl[] [0.0, 0.0, 0.0, 0.0, 0.0, 0.0]  # Pressure Offsets
  w43 = FALSE  # New Step
  w44 = 0  # Stagger Counter
  w45 = FALSE  # Login
  w46 = dbl[] [0.0, 0.0, 0.0, 0.0, 0.0, 0.0]  # Initial Times
  w47 = bool[] [FALSE, FALSE, FALSE, FALSE, FALSE, FALSE]  # pb.Sets
  w48 = bool[] [FALSE, FALSE, FALSE, FALSE, FALSE, FALSE]  # pb.Resets
  w49 = FALSE  # pb.Run Profile
  w50 = FALSE  # Client?
  w51 = dbl[] [0.0, 0.0, 0.0, 0.0, 0.0, 0.0]  # Controller CMDs
  w52 = 0.0  # Last Profile Time
  w53 = u32 0  # Screen Timer
  w54 = 0  # # of Steps
  w55 = 0.0  # Step Time
  w56 = 0.0  # Step Start Time
  w57 = FALSE  # Run Profile
  w59 = 0  # Current Step
  w58 = 0.0  # Step Time Left
  w60 = string[] []  # Profiles
  w62 = string[][] []  # Profile
  w63 = errorcluster {"status"=FALSE, "code"=0, "source"=""}  # Error
  # "Disabled States:\n   Save LS Test Data\n   Allow Data Note"
  n1 = Bundle("Error"=w63, "Profile"=w62, "App Config"="App Config", "Profiles"=w60, "Current Step"=w59, "Step Time Left"=w58, "Run Profile"=w57, "Step Start Time"=w56, "Step Time"=w55, "# of Steps"=w54, "Screen Timer"=w53, "Last Profile Time"=w52, "Controller CMDs"=w51, "Client?"=w50, "pb.Run Profile"=w49, "pb.Resets"=w48, "pb.Sets"=w47, "Initial Times"=w46, "Pressure Offsets"=w41, "Login"=w45, "Stagger Counter"=w44, "New Step"=w43, "Inputs Timer"=w40, "Tank Data"=w20, "Voltage Enable"=w39, "Power Relay"=w38, "Ignition Relay"=w37, "Controller List"=w36, "Alarm Config"=w35, "Alarm Config Path"=w34, "Trip Counters"=w33, "Previous Times"=w32, "Alarm Message 1"=w31, "Alarm Message 2"=w23, "Prev ON Times"=w30, "CalArray"=w29, "Tank CMDs"=w28, "Controller Config"=w27, "Fuel Log Path"=w26, "Pump Data"=w25, "Alarm Latch"=w24, "Time/Date"=w22, "Recording"=w21, "HMI"=w19, "WebDAV Push"=w18, "Email Alarms Disabled"=w17, "Concat Data"=w16, "LS Data"=w15, "Main Tab"=w14, "LS App Config"=w2, "Bank 1 State:"=w13, "Bank 2 State:"=w12, "LS Data Filepath"=w11, "Initial LS Data"=w10, "day of month"=w3, "Pause Test"=w1) -> (w42:T25)  [unwired: 1 in]
  n2 = xnode "Open FPGA VI Reference"("resource name"=tag "RIO0") -> ("FPGA VI Reference Out"=w4:T26, "error out"=w8:errorcluster)  [unwired: 1 in]
  n3 = Generate Occurrence() -> (w6:refnum<k4>)
  n4 = Wait on Occurrence(2:w6) -> (0:w5:bool)  [unwired: 2 in]
  n5 = while {
    shift-right: [w72] -> _
    shift-left: w9 -> [w70]
    shift-right: [w73] -> _
    shift-left: w42 -> [w74]
    tunnel: w4 -> [w71]
    tunnel: w6 -> [w65]
    tunnel: w8 -> [_]
    stop <- FALSE stop-if-true
    n6 = Delete From Array(array=w70, length=1, index=0 ("length")) -> (deleted portion=w66:T14[], array with subset deleted=w69:T14[])
    n7 = Index Array(array=w66) -> (element=w64:T14)  [unwired: 1 in]
    n8 = case shown="\"Update Screen\"" w64 {
      selector: w64 -> [_ _ _ _ _ _ _ _ _ _ _ _ _ _ _ _ _ _ _ _ _ _ _ _ _ _ w1599 _ _ _ _ _ _ _ _ _ w1857 _ _ _ _ _ _ _ _ _ _ _ _ _]
      tunnel: [w80 w713 w841 w876 w883 w905 w925 w933 w948 w962 w997 w1047 w1069 w1127 w1188 w1282 w1346 w1408 w1443 w1470 w1491 w1515 w1544 w1574 w1582 w1587 w1602 w1674 w1700 w1712 w1749 w1761 w1772 w1775 w1785 w1842 w1862 w1880 w1894 w1903 w1912 w1920 w1925 w1942 w1970 w2062 w2076 w2135 w2142 w2148] -> w73
      tunnel: w74 -> [w99 w714 w840 w876 w884 w906 w925 w934 w949 w963 w976 w1029 w1070 w1092 w1189 w1307 w1347 w1408 w1443 w1476 w1492 w1515 w1544 w1574 w1582 w1587 w1600 w1674 w1701 w1711 w1747 w1761 w1772 w1775 w1786 w1842 w1862 w1879 w1894 w1903 w1912 w1920 w1926 w1943 w1971 w2062 w2076 w2136 w2142 w2148]
      tunnel: [w93 w697 w822 w875 w880 w909 w926 w927 w938 w958 w990 w1042 w1050 w1107 w1176 w1277 w1369 w1421 w1439 w1479 w1486 w1516 w1543 w1575 w1581 w1585 w1597 w1680 w1702 w1706 w1743 w1760 w1771 w1776 w1783 w1841 w1863 w1883 w1895 w1904 w1911 w1915 w1934 w1939 w1972 w2061 w2072 w2134 w2143 w2151] -> w72
      tunnel: w71 -> [_ _ w796 _ _ _ _ _ _ _ _ _ _ _ w1152 w1260 _ _ _ _ _ _ _ _ _ w1586 w1601 _ _ w1710 w1748 _ _ _ w1787 _ _ _ _ _ w1907 _ _ _ _ _ _ _ _ _]
      tunnel: w69 -> [w87 w695 w825 w875 w879 w909 w926 w928 w939 w958 w991 w1043 w1051 w1123 w1142 w1292 w1368 w1420 w1440 w1480 w1487 w1516 w1543 w1575 w1581 w1585 w1598 w1681 w1703 w1707 w1742 w1760 w1771 w1777 w1784 w1841 w1863 w1884 w1895 w1904 w1911 w1916 w1935 w1951 w1972 w2061 w2072 w2134 w2143 w2152]
      tunnel: w65 -> [_ _ w834 _ _ _ _ _ _ _ _ _ _ _ _ _ _ _ _ _ _ _ _ _ _ _ _ _ _ _ _ _ _ _ _ _ _ _ _ _ _ _ _ _ _ _ _ _ _ _]
      frame "Main", Default {
        w76 = T14[] [enum."Update Screen", enum."Save LS Data"] items=["Main", "Init Files", "Init", "Unused", "Save As", "Start Profile", "Check Step Time", "Alarm", "Alarm Dismiss", "Run Step", "Stop Profile", "Cycle Reset", "Time Reset", "Time Reset All", "Time Set", "Tare CTs", "Save Profile", "Open Profile", "Get Profiles", "Update Screen", "Update Controls", "Save App Config", "Write Outputs", "Disable Background", "Enable Background", "Get/Release Control", "Log Fuel Change", "Fuel Change Popup", "Read Inputs", "Remote Timer Reset", "Controller Change", "Get Alarms", "Init Alarms", "Save Alarms", "Voltage Selection", "Set Watlow Temp 1", "Set Watlow Temp 2", "Get Pressure", "Write Tare Pressure", "Adjust Controls", "Reinit ADC", "Write Initial Times", "Write Pumps Present", "HMI Command", "Save Pump Times", "Check Pump Stop Time", "Save LS App Config", "Init Data File", "Reset LS Cycles", "Reset Anomalies", "Reset Opens", "Save LS Data", "Save LS Test Data", "Check Serial Numbers", "Main Tab", "Allow Data Note", "Resume Profile"]
        (unwired) Sequence_States."Update Screen"
        n9 = Unbundle By Name(w99) -> ("Run Profile"=w79:bool, "Inputs Timer"=w86:u32, "Screen Timer"=w85:u32)
        n10 = Wait (ms)(milliseconds to wait=u32 10) -> ()  [unwired: 1 out]
        n11 = for {
          N: 78 -> [_]
          shift-right: [w124] -> w80
          shift-left: w99 -> [w123]
          tunnel: [w122] -> w95
          tunnel: [w121] -> w94
          i -> [w120]
          stop <- w121 stop-if-true
          n12 = case shown="77" w120 {
            tunnel: w123 -> [w131 w133 w135 w144 w151 w152 w160 w167 w175 w182 w190 w198 w206 w213 w216 w217 w225 w233 w240 w248 w249 w257 w264 w271 w279 w283 w289 w305 w313 w320 w324 w327 w334 w343 w352 w361 w370 w379 w388 w397 w405 w412 w419 w426 w429 w436 w442 w447 w454 w461 w468 w475 w489 w497 w504 w513 w522 w529 w536 w543 w550 w557 w564 w576 w583 w590 w593 w596 w599 w607 w614 w621 w628 w635 w643 w650 w659]
            tunnel: [w130 w133 w135 w143 w151 w152 w159 w166 w174 w181 w189 w197 w205 w212 w216 w217 w224 w232 w239 w247 w249 w256 w263 w270 w278 w282 w288 w304 w312 w319 w324 w327 w333 w342 w351 w360 w369 w378 w387 w396 w404 w411 w418 w425 w429 w435 w441 w446 w453 w460 w467 w474 w488 w496 w503 w512 w521 w528 w535 w542 w549 w556 w563 w575 w582 w589 w593 w596 w599 w606 w613 w620 w628 w634 w642 w649 w658] -> w124
            tunnel: w123 -> [w129 _ _ w142 w149 _ w157 w164 w173 w180 w188 w196 w204 w211 _ _ w222 w230 w237 w246 _ w255 w262 w269 w277 w284 w291 w306 w314 w321 _ _ w335 w344 w353 w362 w371 w380 w389 w398 w406 w413 w417 w424 _ w437 _ _ w452 w459 w466 w473 w490 w498 w505 w514 w523 w530 w537 w544 w551 w558 w565 w577 w584 w591 _ _ _ w605 w615 w622 _ w633 w641 w648 w657]
            tunnel: [w128 w134 w136 w141 w146 w154 w155 w162 w170 w176 w187 w194 w200 w208 w215 w219 w221 w229 w236 w245 w251 w258 w265 w272 w276 w286 w296 w308 w315 w322 w325 w328 w330 w340 w345 w354 w363 w372 w381 w394 w402 w409 w420 w427 w431 w438 w443 w448 w455 w462 w469 w476 w485 w495 w502 w511 w520 w527 w534 w541 w548 w555 w562 w574 w581 w588 w594 w597 w600 w602 w610 w617 w626 w629 w639 w646 w651] -> w122
            tunnel: [w125 "pb.E Stop" "pb.Save As" w138 "pb.Stop Profile" "pb.Cycle Reset" w158 w165 w171 w178 w183 w192 w202 w209 FALSE ("pb.Tare Pressure") "pb.Time Reset All" w223 w231 w238 w242 "pb.FuelChange" w252 w261 w266 w273 w285 w292 w307 w309 w316 "pb.Alarm OK" "pb.Tare Pressure" w331 w336 w346 w356 w365 w373 w383 w391 w401 w407 w415 w422 w428 w432 FALSE ("HMI Command") FALSE ("HMI Command") w451 w458 w465 w472 w484 w492 w500 w506 w516 w525 w532 w539 w546 w553 w560 w569 w578 w586 "Reset Total Cycles" "Reset Anomalies" "Reset Opens" w603 w612 w619 FALSE ("Reset Opens") w632 w636 w645 w655] -> w121
            frame 0, Default {
              w128 = T14[] [enum."Write Outputs"] items=["Main", "Init Files", "Init", "Unused", "Save As", "Start Profile", "Check Step Time", "Alarm", "Alarm Dismiss", "Run Step", "Stop Profile", "Cycle Reset", "Time Reset", "Time Reset All", "Time Set", "Tare CTs", "Save Profile", "Open Profile", "Get Profiles", "Update Screen", "Update Controls", "Save App Config", "Write Outputs", "Disable Background", "Enable Background", "Get/Release Control", "Log Fuel Change", "Fuel Change Popup", "Read Inputs", "Remote Timer Reset", "Controller Change", "Get Alarms", "Init Alarms", "Save Alarms", "Voltage Selection", "Set Watlow Temp 1", "Set Watlow Temp 2", "Get Pressure", "Write Tare Pressure", "Adjust Controls", "Reinit ADC", "Write Initial Times", "Write Pumps Present", "HMI Command", "Save Pump Times", "Check Pump Stop Time", "Save LS App Config", "Init Data File", "Reset LS Cycles", "Reset Anomalies", "Reset Opens", "Save LS Data", "Save LS Test Data", "Check Serial Numbers", "Main Tab", "Allow Data Note", "Resume Profile"]
              n13 = Unbundle By Name(w129) -> ("Tank CMDs.PS CMD"=w127:dbl)
              n14 = Not Equal?(x=w127, y="Power Supply Cmd:") -> (x != y?=w125:bool)
              n15 = Bundle By Name(cluster=w131, "Tank CMDs.PS CMD"="Power Supply Cmd:") -> (w130:T25)
            }
            frame 1 {
              w134 = T14[] [enum."Stop Profile"] items=["Main", "Init Files", "Init", "Unused", "Save As", "Start Profile", "Check Step Time", "Alarm", "Alarm Dismiss", "Run Step", "Stop Profile", "Cycle Reset", "Time Reset", "Time Reset All", "Time Set", "Tare CTs", "Save Profile", "Open Profile", "Get Profiles", "Update Screen", "Update Controls", "Save App Config", "Write Outputs", "Disable Background", "Enable Background", "Get/Release Control", "Log Fuel Change", "Fuel Change Popup", "Read Inputs", "Remote Timer Reset", "Controller Change", "Get Alarms", "Init Alarms", "Save Alarms", "Voltage Selection", "Set Watlow Temp 1", "Set Watlow Temp 2", "Get Pressure", "Write Tare Pressure", "Adjust Controls", "Reinit ADC", "Write Initial Times", "Write Pumps Present", "HMI Command", "Save Pump Times", "Check Pump Stop Time", "Save LS App Config", "Init Data File", "Reset LS Cycles", "Reset Anomalies", "Reset Opens", "Save LS Data", "Save LS Test Data", "Check Serial Numbers", "Main Tab", "Allow Data Note", "Resume Profile"]
            }
            frame 2 {
              w136 = T14[] [enum."Disable Background", enum."Save As"] items=["Main", "Init Files", "Init", "Unused", "Save As", "Start Profile", "Check Step Time", "Alarm", "Alarm Dismiss", "Run Step", "Stop Profile", "Cycle Reset", "Time Reset", "Time Reset All", "Time Set", "Tare CTs", "Save Profile", "Open Profile", "Get Profiles", "Update Screen", "Update Controls", "Save App Config", "Write Outputs", "Disable Background", "Enable Background", "Get/Release Control", "Log Fuel Change", "Fuel Change Popup", "Read Inputs", "Remote Timer Reset", "Controller Change", "Get Alarms", "Init Alarms", "Save Alarms", "Voltage Selection", "Set Watlow Temp 1", "Set Watlow Temp 2", "Get Pressure", "Write Tare Pressure", "Adjust Controls", "Reinit ADC", "Write Initial Times", "Write Pumps Present", "HMI Command", "Save Pump Times", "Check Pump Stop Time", "Save LS App Config", "Init Data File", "Reset LS Cycles", "Reset Anomalies", "Reset Opens", "Save LS Data", "Save LS Test Data", "Check Serial Numbers", "Main Tab", "Allow Data Note", "Resume Profile"]
            }
            frame 3 {
              w141 = T14[] [enum."Voltage Selection", enum."Start Profile"] items=["Main", "Init Files", "Init", "Unused", "Save As", "Start Profile", "Check Step Time", "Alarm", "Alarm Dismiss", "Run Step", "Stop Profile", "Cycle Reset", "Time Reset", "Time Reset All", "Time Set", "Tare CTs", "Save Profile", "Open Profile", "Get Profiles", "Update Screen", "Update Controls", "Save App Config", "Write Outputs", "Disable Background", "Enable Background", "Get/Release Control", "Log Fuel Change", "Fuel Change Popup", "Read Inputs", "Remote Timer Reset", "Controller Change", "Get Alarms", "Init Alarms", "Save Alarms", "Voltage Selection", "Set Watlow Temp 1", "Set Watlow Temp 2", "Get Pressure", "Write Tare Pressure", "Adjust Controls", "Reinit ADC", "Write Initial Times", "Write Pumps Present", "HMI Command", "Save Pump Times", "Check Pump Stop Time", "Save LS App Config", "Init Data File", "Reset LS Cycles", "Reset Anomalies", "Reset Opens", "Save LS Data", "Save LS Test Data", "Check Serial Numbers", "Main Tab", "Allow Data Note", "Resume Profile"]
              n16 = Unbundle By Name(w142) -> ("pb.Run Profile"=w140:bool)
              n17 = Greater?(x="pb.Run Profile", y=w140) -> (0:w138:bool)
              n18 = Bundle By Name(cluster=w144, "pb.Run Profile"="pb.Run Profile") -> (w143:T25)
            }
            frame 4 {
              w145 = T14[] [enum."Stop Profile", enum."Save LS Test Data"] items=["Main", "Init Files", "Init", "Unused", "Save As", "Start Profile", "Check Step Time", "Alarm", "Alarm Dismiss", "Run Step", "Stop Profile", "Cycle Reset", "Time Reset", "Time Reset All", "Time Set", "Tare CTs", "Save Profile", "Open Profile", "Get Profiles", "Update Screen", "Update Controls", "Save App Config", "Write Outputs", "Disable Background", "Enable Background", "Get/Release Control", "Log Fuel Change", "Fuel Change Popup", "Read Inputs", "Remote Timer Reset", "Controller Change", "Get Alarms", "Init Alarms", "Save Alarms", "Voltage Selection", "Set Watlow Temp 1", "Set Watlow Temp 2", "Get Pressure", "Write Tare Pressure", "Adjust Controls", "Reinit ADC", "Write Initial Times", "Write Pumps Present", "HMI Command", "Save Pump Times", "Check Pump Stop Time", "Save LS App Config", "Init Data File", "Reset LS Cycles", "Reset Anomalies", "Reset Opens", "Save LS Data", "Save LS Test Data", "Check Serial Numbers", "Main Tab", "Allow Data Note", "Resume Profile"]
              w147 = T14[] [enum."Stop Profile", enum."Save LS Test Data", enum."Allow Data Note"] items=["Main", "Init Files", "Init", "Unused", "Save As", "Start Profile", "Check Step Time", "Alarm", "Alarm Dismiss", "Run Step", "Stop Profile", "Cycle Reset", "Time Reset", "Time Reset All", "Time Set", "Tare CTs", "Save Profile", "Open Profile", "Get Profiles", "Update Screen", "Update Controls", "Save App Config", "Write Outputs", "Disable Background", "Enable Background", "Get/Release Control", "Log Fuel Change", "Fuel Change Popup", "Read Inputs", "Remote Timer Reset", "Controller Change", "Get Alarms", "Init Alarms", "Save Alarms", "Voltage Selection", "Set Watlow Temp 1", "Set Watlow Temp 2", "Get Pressure", "Write Tare Pressure", "Adjust Controls", "Reinit ADC", "Write Initial Times", "Write Pumps Present", "HMI Command", "Save Pump Times", "Check Pump Stop Time", "Save LS App Config", "Init Data File", "Reset LS Cycles", "Reset Anomalies", "Reset Opens", "Save LS Data", "Save LS Test Data", "Check Serial Numbers", "Main Tab", "Allow Data Note", "Resume Profile"]
              n19 = Unbundle By Name(w149) -> ("pb.Run Profile"=w148:bool)
              n20 = Select(t=w147, s=w148, f=w145) -> (s? t:f=w146:T14[])
            }
            frame 5 {
              w154 = T14[] [enum."Disable Background", enum."Cycle Reset"] items=["Main", "Init Files", "Init", "Unused", "Save As", "Start Profile", "Check Step Time", "Alarm", "Alarm Dismiss", "Run Step", "Stop Profile", "Cycle Reset", "Time Reset", "Time Reset All", "Time Set", "Tare CTs", "Save Profile", "Open Profile", "Get Profiles", "Update Screen", "Update Controls", "Save App Config", "Write Outputs", "Disable Background", "Enable Background", "Get/Release Control", "Log Fuel Change", "Fuel Change Popup", "Read Inputs", "Remote Timer Reset", "Controller Change", "Get Alarms", "Init Alarms", "Save Alarms", "Voltage Selection", "Set Watlow Temp 1", "Set Watlow Temp 2", "Get Pressure", "Write Tare Pressure", "Adjust Controls", "Reinit ADC", "Write Initial Times", "Write Pumps Present", "HMI Command", "Save Pump Times", "Check Pump Stop Time", "Save LS App Config", "Init Data File", "Reset LS Cycles", "Reset Anomalies", "Reset Opens", "Save LS Data", "Save LS Test Data", "Check Serial Numbers", "Main Tab", "Allow Data Note", "Resume Profile"]
            }
            frame 6 {
              w155 = T14[] [enum."Disable Background", enum."Time Reset", enum."Update Controls"] items=["Main", "Init Files", "Init", "Unused", "Save As", "Start Profile", "Check Step Time", "Alarm", "Alarm Dismiss", "Run Step", "Stop Profile", "Cycle Reset", "Time Reset", "Time Reset All", "Time Set", "Tare CTs", "Save Profile", "Open Profile", "Get Profiles", "Update Screen", "Update Controls", "Save App Config", "Write Outputs", "Disable Background", "Enable Background", "Get/Release Control", "Log Fuel Change", "Fuel Change Popup", "Read Inputs", "Remote Timer Reset", "Controller Change", "Get Alarms", "Init Alarms", "Save Alarms", "Voltage Selection", "Set Watlow Temp 1", "Set Watlow Temp 2", "Get Pressure", "Write Tare Pressure", "Adjust Controls", "Reinit ADC", "Write Initial Times", "Write Pumps Present", "HMI Command", "Save Pump Times", "Check Pump Stop Time", "Save LS App Config", "Init Data File", "Reset LS Cycles", "Reset Anomalies", "Reset Opens", "Save LS Data", "Save LS Test Data", "Check Serial Numbers", "Main Tab", "Allow Data Note", "Resume Profile"]
              n21 = Unbundle By Name(w157) -> ("pb.Resets"=w161:bool[])
              n22 = Greater?(x="pb.Resets", y=w161) -> (0:w158:bool)
              n23 = Bundle By Name(cluster=w160, "pb.Resets"="pb.Resets") -> (w159:T25)
            }
            frame 7 {
              w162 = T14[] [enum."Disable Background", enum."Time Set", enum."Update Controls"] items=["Main", "Init Files", "Init", "Unused", "Save As", "Start Profile", "Check Step Time", "Alarm", "Alarm Dismiss", "Run Step", "Stop Profile", "Cycle Reset", "Time Reset", "Time Reset All", "Time Set", "Tare CTs", "Save Profile", "Open Profile", "Get Profiles", "Update Screen", "Update Controls", "Save App Config", "Write Outputs", "Disable Background", "Enable Background", "Get/Release Control", "Log Fuel Change", "Fuel Change Popup", "Read Inputs", "Remote Timer Reset", "Controller Change", "Get Alarms", "Init Alarms", "Save Alarms", "Voltage Selection", "Set Watlow Temp 1", "Set Watlow Temp 2", "Get Pressure", "Write Tare Pressure", "Adjust Controls", "Reinit ADC", "Write Initial Times", "Write Pumps Present", "HMI Command", "Save Pump Times", "Check Pump Stop Time", "Save LS App Config", "Init Data File", "Reset LS Cycles", "Reset Anomalies", "Reset Opens", "Save LS Data", "Save LS Test Data", "Check Serial Numbers", "Main Tab", "Allow Data Note", "Resume Profile"]
              n24 = Unbundle By Name(w164) -> ("pb.Sets"=w168:bool[])
              n25 = Greater?(x="pb.Sets", y=w168) -> (0:w165:bool)
              n26 = Bundle By Name(cluster=w167, "pb.Sets"="pb.Sets") -> (w166:T25)
            }
            frame 8 {
              w170 = T14[] [enum."Save Profile", enum."Update Controls"] items=["Main", "Init Files", "Init", "Unused", "Save As", "Start Profile", "Check Step Time", "Alarm", "Alarm Dismiss", "Run Step", "Stop Profile", "Cycle Reset", "Time Reset", "Time Reset All", "Time Set", "Tare CTs", "Save Profile", "Open Profile", "Get Profiles", "Update Screen", "Update Controls", "Save App Config", "Write Outputs", "Disable Background", "Enable Background", "Get/Release Control", "Log Fuel Change", "Fuel Change Popup", "Read Inputs", "Remote Timer Reset", "Controller Change", "Get Alarms", "Init Alarms", "Save Alarms", "Voltage Selection", "Set Watlow Temp 1", "Set Watlow Temp 2", "Get Pressure", "Write Tare Pressure", "Adjust Controls", "Reinit ADC", "Write Initial Times", "Write Pumps Present", "HMI Command", "Save Pump Times", "Check Pump Stop Time", "Save LS App Config", "Init Data File", "Reset LS Cycles", "Reset Anomalies", "Reset Opens", "Save LS Data", "Save LS Test Data", "Check Serial Numbers", "Main Tab", "Allow Data Note", "Resume Profile"]
              n27 = Unbundle By Name(w173) -> ("Profile"=w172:string[][])
              n28 = Not Equal?(x=w172, y="Profile:") -> (x != y?=w171:bool)
              n29 = Bundle By Name(cluster=w175, "Profile"="Profile:") -> (w174:T25)
            }
            frame 9 {
              w176 = T14[] [enum."Open Profile", enum."Update Controls"] items=["Main", "Init Files", "Init", "Unused", "Save As", "Start Profile", "Check Step Time", "Alarm", "Alarm Dismiss", "Run Step", "Stop Profile", "Cycle Reset", "Time Reset", "Time Reset All", "Time Set", "Tare CTs", "Save Profile", "Open Profile", "Get Profiles", "Update Screen", "Update Controls", "Save App Config", "Write Outputs", "Disable Background", "Enable Background", "Get/Release Control", "Log Fuel Change", "Fuel Change Popup", "Read Inputs", "Remote Timer Reset", "Controller Change", "Get Alarms", "Init Alarms", "Save Alarms", "Voltage Selection", "Set Watlow Temp 1", "Set Watlow Temp 2", "Get Pressure", "Write Tare Pressure", "Adjust Controls", "Reinit ADC", "Write Initial Times", "Write Pumps Present", "HMI Command", "Save Pump Times", "Check Pump Stop Time", "Save LS App Config", "Init Data File", "Reset LS Cycles", "Reset Anomalies", "Reset Opens", "Save LS Data", "Save LS Test Data", "Check Serial Numbers", "Main Tab", "Allow Data Note", "Resume Profile"]
              n30 = Unbundle By Name(w180) -> ("App Config.Current Profile"=w179:string)
              n31 = Not Equal?(x=w179, y="Profile Name:") -> (x != y?=w178:bool)
              n32 = Bundle By Name(cluster=w182, "App Config.Current Profile"="Profile Name:") -> (w181:T25)
            }
            frame 10 {
              w187 = T14[] [enum."Write Outputs"] items=["Main", "Init Files", "Init", "Unused", "Save As", "Start Profile", "Check Step Time", "Alarm", "Alarm Dismiss", "Run Step", "Stop Profile", "Cycle Reset", "Time Reset", "Time Reset All", "Time Set", "Tare CTs", "Save Profile", "Open Profile", "Get Profiles", "Update Screen", "Update Controls", "Save App Config", "Write Outputs", "Disable Background", "Enable Background", "Get/Release Control", "Log Fuel Change", "Fuel Change Popup", "Read Inputs", "Remote Timer Reset", "Controller Change", "Get Alarms", "Init Alarms", "Save Alarms", "Voltage Selection", "Set Watlow Temp 1", "Set Watlow Temp 2", "Get Pressure", "Write Tare Pressure", "Adjust Controls", "Reinit ADC", "Write Initial Times", "Write Pumps Present", "HMI Command", "Save Pump Times", "Check Pump Stop Time", "Save LS App Config", "Init Data File", "Reset LS Cycles", "Reset Anomalies", "Reset Opens", "Save LS Data", "Save LS Test Data", "Check Serial Numbers", "Main Tab", "Allow Data Note", "Resume Profile"]
              n33 = Unbundle By Name(w188) -> ("Controller CMDs"=w186:dbl[])
              n34 = Not Equal?(x="Controller\nCMD", y=w186) -> (x != y?=w184:bool[])
              n35 = Or Array Elements(Boolean array=w184) -> (logical OR=w183:bool)
              n36 = Bundle By Name(cluster=w190, "Controller CMDs"="Controller\nCMD") -> (w189:T25)
            }
            frame 11 {
              w194 = T14[] [enum."Get/Release Control"] items=["Main", "Init Files", "Init", "Unused", "Save As", "Start Profile", "Check Step Time", "Alarm", "Alarm Dismiss", "Run Step", "Stop Profile", "Cycle Reset", "Time Reset", "Time Reset All", "Time Set", "Tare CTs", "Save Profile", "Open Profile", "Get Profiles", "Update Screen", "Update Controls", "Save App Config", "Write Outputs", "Disable Background", "Enable Background", "Get/Release Control", "Log Fuel Change", "Fuel Change Popup", "Read Inputs", "Remote Timer Reset", "Controller Change", "Get Alarms", "Init Alarms", "Save Alarms", "Voltage Selection", "Set Watlow Temp 1", "Set Watlow Temp 2", "Get Pressure", "Write Tare Pressure", "Adjust Controls", "Reinit ADC", "Write Initial Times", "Write Pumps Present", "HMI Command", "Save Pump Times", "Check Pump Stop Time", "Save LS App Config", "Init Data File", "Reset LS Cycles", "Reset Anomalies", "Reset Opens", "Save LS Data", "Save LS Test Data", "Check Serial Numbers", "Main Tab", "Allow Data Note", "Resume Profile"]
              n37 = Unbundle By Name(w196) -> ("Client?"=w193:bool, "Profiles"=w195:string[])
              n38 = call "App Global.vi"() -> ("Client? OUT"=w191:bool)  [unwired: 9 in, 2 out]
              n39 = Greater?(x=w191, y=w193) -> (0:w192:bool)
              n40 = case shown="True" w192 {
                tunnel: w195 -> [_ w199]
                frame False {
                }
                frame True {
                  n41 = property on="Profile Name:" class="CmbBox"("Strings[]"=w199) -> ()  [unwired: 2 in, 2 out]
                }
              }
              n42 = Bundle By Name(cluster=w198, "Client?"=w191) -> (w197:T25)
            }
            frame 13 {
              w200 = T14[] [enum."Init Data File", enum."Save LS App Config", enum."Save App Config"] items=["Main", "Init Files", "Init", "Unused", "Save As", "Start Profile", "Check Step Time", "Alarm", "Alarm Dismiss", "Run Step", "Stop Profile", "Cycle Reset", "Time Reset", "Time Reset All", "Time Set", "Tare CTs", "Save Profile", "Open Profile", "Get Profiles", "Update Screen", "Update Controls", "Save App Config", "Write Outputs", "Disable Background", "Enable Background", "Get/Release Control", "Log Fuel Change", "Fuel Change Popup", "Read Inputs", "Remote Timer Reset", "Controller Change", "Get Alarms", "Init Alarms", "Save Alarms", "Voltage Selection", "Set Watlow Temp 1", "Set Watlow Temp 2", "Get Pressure", "Write Tare Pressure", "Adjust Controls", "Reinit ADC", "Write Initial Times", "Write Pumps Present", "HMI Command", "Save Pump Times", "Check Pump Stop Time", "Save LS App Config", "Init Data File", "Reset LS Cycles", "Reset Anomalies", "Reset Opens", "Save LS Data", "Save LS Test Data", "Check Serial Numbers", "Main Tab", "Allow Data Note", "Resume Profile"]
              n43 = Unbundle By Name(w204) -> ("App Config.CA Number"=w203:string)
              n44 = Not Equal?(x=w203, y="CA Number:") -> (x != y?=w202:bool)
              n45 = Bundle By Name(cluster=w206, "App Config.CA Number"="CA Number:") -> (w205:T25)
            }
            frame 14 {
              w208 = T14[] [enum."Save App Config", enum."Controller Change", enum."Write Outputs"] items=["Main", "Init Files", "Init", "Unused", "Save As", "Start Profile", "Check Step Time", "Alarm", "Alarm Dismiss", "Run Step", "Stop Profile", "Cycle Reset", "Time Reset", "Time Reset All", "Time Set", "Tare CTs", "Save Profile", "Open Profile", "Get Profiles", "Update Screen", "Update Controls", "Save App Config", "Write Outputs", "Disable Background", "Enable Background", "Get/Release Control", "Log Fuel Change", "Fuel Change Popup", "Read Inputs", "Remote Timer Reset", "Controller Change", "Get Alarms", "Init Alarms", "Save Alarms", "Voltage Selection", "Set Watlow Temp 1", "Set Watlow Temp 2", "Get Pressure", "Write Tare Pressure", "Adjust Controls", "Reinit ADC", "Write Initial Times", "Write Pumps Present", "HMI Command", "Save Pump Times", "Check Pump Stop Time", "Save LS App Config", "Init Data File", "Reset LS Cycles", "Reset Anomalies", "Reset Opens", "Save LS Data", "Save LS Test Data", "Check Serial Numbers", "Main Tab", "Allow Data Note", "Resume Profile"]
              n46 = Unbundle By Name(w211) -> ("App Config.Controller Type:"=w210:T3)
              n47 = Not Equal?(x=w210, y="Controller Type:") -> (x != y?=w209:bool)
              n48 = Bundle By Name(cluster=w213, "App Config.Controller Type:"="Controller Type:") -> (w212:T25)
            }
            frame 15 {
              w215 = T14[] [] items=["Main", "Init Files", "Init", "Unused", "Save As", "Start Profile", "Check Step Time", "Alarm", "Alarm Dismiss", "Run Step", "Stop Profile", "Cycle Reset", "Time Reset", "Time Reset All", "Time Set", "Tare CTs", "Save Profile", "Open Profile", "Get Profiles", "Update Screen", "Update Controls", "Save App Config", "Write Outputs", "Disable Background", "Enable Background", "Get/Release Control", "Log Fuel Change", "Fuel Change Popup", "Read Inputs", "Remote Timer Reset", "Controller Change", "Get Alarms", "Init Alarms", "Save Alarms", "Voltage Selection", "Set Watlow Temp 1", "Set Watlow Temp 2", "Get Pressure", "Write Tare Pressure", "Adjust Controls", "Reinit ADC", "Write Initial Times", "Write Pumps Present", "HMI Command", "Save Pump Times", "Check Pump Stop Time", "Save LS App Config", "Init Data File", "Reset LS Cycles", "Reset Anomalies", "Reset Opens", "Save LS Data", "Save LS Test Data", "Check Serial Numbers", "Main Tab", "Allow Data Note", "Resume Profile"]
            }
            frame 16 {
              w219 = T14[] [enum."Disable Background", enum."Time Reset All", enum."Update Controls"] items=["Main", "Init Files", "Init", "Unused", "Save As", "Start Profile", "Check Step Time", "Alarm", "Alarm Dismiss", "Run Step", "Stop Profile", "Cycle Reset", "Time Reset", "Time Reset All", "Time Set", "Tare CTs", "Save Profile", "Open Profile", "Get Profiles", "Update Screen", "Update Controls", "Save App Config", "Write Outputs", "Disable Background", "Enable Background", "Get/Release Control", "Log Fuel Change", "Fuel Change Popup", "Read Inputs", "Remote Timer Reset", "Controller Change", "Get Alarms", "Init Alarms", "Save Alarms", "Voltage Selection", "Set Watlow Temp 1", "Set Watlow Temp 2", "Get Pressure", "Write Tare Pressure", "Adjust Controls", "Reinit ADC", "Write Initial Times", "Write Pumps Present", "HMI Command", "Save Pump Times", "Check Pump Stop Time", "Save LS App Config", "Init Data File", "Reset LS Cycles", "Reset Anomalies", "Reset Opens", "Save LS Data", "Save LS Test Data", "Check Serial Numbers", "Main Tab", "Allow Data Note", "Resume Profile"]
            }
            frame 17 {
              w221 = T14[] [enum."Save App Config", enum."Write Pumps Present"] items=["Main", "Init Files", "Init", "Unused", "Save As", "Start Profile", "Check Step Time", "Alarm", "Alarm Dismiss", "Run Step", "Stop Profile", "Cycle Reset", "Time Reset", "Time Reset All", "Time Set", "Tare CTs", "Save Profile", "Open Profile", "Get Profiles", "Update Screen", "Update Controls", "Save App Config", "Write Outputs", "Disable Background", "Enable Background", "Get/Release Control", "Log Fuel Change", "Fuel Change Popup", "Read Inputs", "Remote Timer Reset", "Controller Change", "Get Alarms", "Init Alarms", "Save Alarms", "Voltage Selection", "Set Watlow Temp 1", "Set Watlow Temp 2", "Get Pressure", "Write Tare Pressure", "Adjust Controls", "Reinit ADC", "Write Initial Times", "Write Pumps Present", "HMI Command", "Save Pump Times", "Check Pump Stop Time", "Save LS App Config", "Init Data File", "Reset LS Cycles", "Reset Anomalies", "Reset Opens", "Save LS Data", "Save LS Test Data", "Check Serial Numbers", "Main Tab", "Allow Data Note", "Resume Profile"]
              n49 = Unbundle By Name(w222) -> ("App Config.Pumps Present"=w226:T8)
              n50 = Not Equal?(x="Pumps Present", y=w226) -> (x != y?=w223:bool)
              n51 = Bundle By Name(cluster=w225, "App Config.Pumps Present"="Pumps Present") -> (w224:T25)
            }
            frame 18 {
              w229 = T14[] [enum."Get/Release Control"] items=["Main", "Init Files", "Init", "Unused", "Save As", "Start Profile", "Check Step Time", "Alarm", "Alarm Dismiss", "Run Step", "Stop Profile", "Cycle Reset", "Time Reset", "Time Reset All", "Time Set", "Tare CTs", "Save Profile", "Open Profile", "Get Profiles", "Update Screen", "Update Controls", "Save App Config", "Write Outputs", "Disable Background", "Enable Background", "Get/Release Control", "Log Fuel Change", "Fuel Change Popup", "Read Inputs", "Remote Timer Reset", "Controller Change", "Get Alarms", "Init Alarms", "Save Alarms", "Voltage Selection", "Set Watlow Temp 1", "Set Watlow Temp 2", "Get Pressure", "Write Tare Pressure", "Adjust Controls", "Reinit ADC", "Write Initial Times", "Write Pumps Present", "HMI Command", "Save Pump Times", "Check Pump Stop Time", "Save LS App Config", "Init Data File", "Reset LS Cycles", "Reset Anomalies", "Reset Opens", "Save LS Data", "Save LS Test Data", "Check Serial Numbers", "Main Tab", "Allow Data Note", "Resume Profile"]
              n52 = Unbundle By Name(w230) -> ("Login"=w234:bool)
              n53 = call "App Global.vi"("Mode"=App_Global_Mode."Write Login", "Login"="Login") -> ()  [unwired: 7 in, 3 out]
              n54 = Not Equal?(x="Login", y=w234) -> (x != y?=w231:bool)
              n55 = Bundle By Name(cluster=w233, "Login"="Login") -> (w232:T25)
            }
            frame 19 {
              w236 = T14[] [enum."Save App Config"] items=["Main", "Init Files", "Init", "Unused", "Save As", "Start Profile", "Check Step Time", "Alarm", "Alarm Dismiss", "Run Step", "Stop Profile", "Cycle Reset", "Time Reset", "Time Reset All", "Time Set", "Tare CTs", "Save Profile", "Open Profile", "Get Profiles", "Update Screen", "Update Controls", "Save App Config", "Write Outputs", "Disable Background", "Enable Background", "Get/Release Control", "Log Fuel Change", "Fuel Change Popup", "Read Inputs", "Remote Timer Reset", "Controller Change", "Get Alarms", "Init Alarms", "Save Alarms", "Voltage Selection", "Set Watlow Temp 1", "Set Watlow Temp 2", "Get Pressure", "Write Tare Pressure", "Adjust Controls", "Reinit ADC", "Write Initial Times", "Write Pumps Present", "HMI Command", "Save Pump Times", "Check Pump Stop Time", "Save LS App Config", "Init Data File", "Reset LS Cycles", "Reset Anomalies", "Reset Opens", "Save LS Data", "Save LS Test Data", "Check Serial Numbers", "Main Tab", "Allow Data Note", "Resume Profile"]
              n56 = Unbundle By Name(w237) -> ("App Config.Stagger Time (ms)"=w241:i32)
              n57 = Not Equal?(x="Stagger Time (ms):", y=w241) -> (x != y?=w238:bool)
              n58 = Bundle By Name(cluster=w240, "App Config.Stagger Time (ms)"="Stagger Time (ms):") -> (w239:T25)
            }
            frame 20 {
              w245 = T14[] [enum."Write Outputs"] items=["Main", "Init Files", "Init", "Unused", "Save As", "Start Profile", "Check Step Time", "Alarm", "Alarm Dismiss", "Run Step", "Stop Profile", "Cycle Reset", "Time Reset", "Time Reset All", "Time Set", "Tare CTs", "Save Profile", "Open Profile", "Get Profiles", "Update Screen", "Update Controls", "Save App Config", "Write Outputs", "Disable Background", "Enable Background", "Get/Release Control", "Log Fuel Change", "Fuel Change Popup", "Read Inputs", "Remote Timer Reset", "Controller Change", "Get Alarms", "Init Alarms", "Save Alarms", "Voltage Selection", "Set Watlow Temp 1", "Set Watlow Temp 2", "Get Pressure", "Write Tare Pressure", "Adjust Controls", "Reinit ADC", "Write Initial Times", "Write Pumps Present", "HMI Command", "Save Pump Times", "Check Pump Stop Time", "Save LS App Config", "Init Data File", "Reset LS Cycles", "Reset Anomalies", "Reset Opens", "Save LS Data", "Save LS Test Data", "Check Serial Numbers", "Main Tab", "Allow Data Note", "Resume Profile"]
              n59 = Unbundle By Name(w246) -> ("Tank CMDs.Press CMD"=w244:dbl)
              n60 = Not Equal?(x="PressureCMD", y=w244) -> (x != y?=w242:bool)
              n61 = Bundle By Name(cluster=w248, "Tank CMDs.Press CMD"="PressureCMD") -> (w247:T25)
            }
            frame 21 {
              w251 = T14[] [enum."Disable Background", enum."Log Fuel Change", enum."Fuel Change Popup"] items=["Main", "Init Files", "Init", "Unused", "Save As", "Start Profile", "Check Step Time", "Alarm", "Alarm Dismiss", "Run Step", "Stop Profile", "Cycle Reset", "Time Reset", "Time Reset All", "Time Set", "Tare CTs", "Save Profile", "Open Profile", "Get Profiles", "Update Screen", "Update Controls", "Save App Config", "Write Outputs", "Disable Background", "Enable Background", "Get/Release Control", "Log Fuel Change", "Fuel Change Popup", "Read Inputs", "Remote Timer Reset", "Controller Change", "Get Alarms", "Init Alarms", "Save Alarms", "Voltage Selection", "Set Watlow Temp 1", "Set Watlow Temp 2", "Get Pressure", "Write Tare Pressure", "Adjust Controls", "Reinit ADC", "Write Initial Times", "Write Pumps Present", "HMI Command", "Save Pump Times", "Check Pump Stop Time", "Save LS App Config", "Init Data File", "Reset LS Cycles", "Reset Anomalies", "Reset Opens", "Save LS Data", "Save LS Test Data", "Check Serial Numbers", "Main Tab", "Allow Data Note", "Resume Profile"]
            }
            frame 22 {
              w258 = T14[] [enum."Save App Config"] items=["Main", "Init Files", "Init", "Unused", "Save As", "Start Profile", "Check Step Time", "Alarm", "Alarm Dismiss", "Run Step", "Stop Profile", "Cycle Reset", "Time Reset", "Time Reset All", "Time Set", "Tare CTs", "Save Profile", "Open Profile", "Get Profiles", "Update Screen", "Update Controls", "Save App Config", "Write Outputs", "Disable Background", "Enable Background", "Get/Release Control", "Log Fuel Change", "Fuel Change Popup", "Read Inputs", "Remote Timer Reset", "Controller Change", "Get Alarms", "Init Alarms", "Save Alarms", "Voltage Selection", "Set Watlow Temp 1", "Set Watlow Temp 2", "Get Pressure", "Write Tare Pressure", "Adjust Controls", "Reinit ADC", "Write Initial Times", "Write Pumps Present", "HMI Command", "Save Pump Times", "Check Pump Stop Time", "Save LS App Config", "Init Data File", "Reset LS Cycles", "Reset Anomalies", "Reset Opens", "Save LS Data", "Save LS Test Data", "Check Serial Numbers", "Main Tab", "Allow Data Note", "Resume Profile"]
              n62 = Unbundle By Name(w255) -> ("App Config.Tank 1 Fuel"=w254:string)
              n63 = Not Equal?(x=w254, y="Tank 1 Fuel Type:") -> (x != y?=w252:bool)
              n64 = Bundle By Name(cluster=w257, "App Config.Tank 1 Fuel"="Tank 1 Fuel Type:") -> (w256:T25)
            }
            frame 23 {
              w265 = T14[] [enum."Save App Config"] items=["Main", "Init Files", "Init", "Unused", "Save As", "Start Profile", "Check Step Time", "Alarm", "Alarm Dismiss", "Run Step", "Stop Profile", "Cycle Reset", "Time Reset", "Time Reset All", "Time Set", "Tare CTs", "Save Profile", "Open Profile", "Get Profiles", "Update Screen", "Update Controls", "Save App Config", "Write Outputs", "Disable Background", "Enable Background", "Get/Release Control", "Log Fuel Change", "Fuel Change Popup", "Read Inputs", "Remote Timer Reset", "Controller Change", "Get Alarms", "Init Alarms", "Save Alarms", "Voltage Selection", "Set Watlow Temp 1", "Set Watlow Temp 2", "Get Pressure", "Write Tare Pressure", "Adjust Controls", "Reinit ADC", "Write Initial Times", "Write Pumps Present", "HMI Command", "Save Pump Times", "Check Pump Stop Time", "Save LS App Config", "Init Data File", "Reset LS Cycles", "Reset Anomalies", "Reset Opens", "Save LS Data", "Save LS Test Data", "Check Serial Numbers", "Main Tab", "Allow Data Note", "Resume Profile"]
              n65 = Unbundle By Name(w262) -> ("App Config.Tank 2 Fuel"=w260:string)
              n66 = Not Equal?(x=w260, y="Tank 2 Fuel Type:") -> (x != y?=w261:bool)
              n67 = Bundle By Name(cluster=w264, "App Config.Tank 2 Fuel"="Tank 2 Fuel Type:") -> (w263:T25)
            }
            frame 24 {
              w272 = T14[] [enum."Save App Config"] items=["Main", "Init Files", "Init", "Unused", "Save As", "Start Profile", "Check Step Time", "Alarm", "Alarm Dismiss", "Run Step", "Stop Profile", "Cycle Reset", "Time Reset", "Time Reset All", "Time Set", "Tare CTs", "Save Profile", "Open Profile", "Get Profiles", "Update Screen", "Update Controls", "Save App Config", "Write Outputs", "Disable Background", "Enable Background", "Get/Release Control", "Log Fuel Change", "Fuel Change Popup", "Read Inputs", "Remote Timer Reset", "Controller Change", "Get Alarms", "Init Alarms", "Save Alarms", "Voltage Selection", "Set Watlow Temp 1", "Set Watlow Temp 2", "Get Pressure", "Write Tare Pressure", "Adjust Controls", "Reinit ADC", "Write Initial Times", "Write Pumps Present", "HMI Command", "Save Pump Times", "Check Pump Stop Time", "Save LS App Config", "Init Data File", "Reset LS Cycles", "Reset Anomalies", "Reset Opens", "Save LS Data", "Save LS Test Data", "Check Serial Numbers", "Main Tab", "Allow Data Note", "Resume Profile"]
              n68 = Unbundle By Name(w269) -> ("App Config.Serial Numbers"=w268:T40)
              n69 = Not Equal?(x=w268, y="Serial Numbers") -> (x != y?=w266:bool)
              n70 = Bundle By Name(cluster=w271, "App Config.Serial Numbers"="Serial Numbers") -> (w270:T25)
            }
            frame 25 {
              w276 = T14[] [enum."Write Pumps Present", enum."Save App Config"] items=["Main", "Init Files", "Init", "Unused", "Save As", "Start Profile", "Check Step Time", "Alarm", "Alarm Dismiss", "Run Step", "Stop Profile", "Cycle Reset", "Time Reset", "Time Reset All", "Time Set", "Tare CTs", "Save Profile", "Open Profile", "Get Profiles", "Update Screen", "Update Controls", "Save App Config", "Write Outputs", "Disable Background", "Enable Background", "Get/Release Control", "Log Fuel Change", "Fuel Change Popup", "Read Inputs", "Remote Timer Reset", "Controller Change", "Get Alarms", "Init Alarms", "Save Alarms", "Voltage Selection", "Set Watlow Temp 1", "Set Watlow Temp 2", "Get Pressure", "Write Tare Pressure", "Adjust Controls", "Reinit ADC", "Write Initial Times", "Write Pumps Present", "HMI Command", "Save Pump Times", "Check Pump Stop Time", "Save LS App Config", "Init Data File", "Reset LS Cycles", "Reset Anomalies", "Reset Opens", "Save LS Data", "Save LS Test Data", "Check Serial Numbers", "Main Tab", "Allow Data Note", "Resume Profile"]
              n71 = Unbundle By Name(w277) -> ("Power Relay"=w275:T8)
              n72 = Not Equal?(x="Power Relay", y=w275) -> (x != y?=w273:bool)
              n73 = Bundle By Name(cluster=w279, "Power Relay"="Power Relay") -> (w278:T25)
            }
            frame 26 {
              w286 = T14[] [enum."Write Pumps Present", enum."Save App Config"] items=["Main", "Init Files", "Init", "Unused", "Save As", "Start Profile", "Check Step Time", "Alarm", "Alarm Dismiss", "Run Step", "Stop Profile", "Cycle Reset", "Time Reset", "Time Reset All", "Time Set", "Tare CTs", "Save Profile", "Open Profile", "Get Profiles", "Update Screen", "Update Controls", "Save App Config", "Write Outputs", "Disable Background", "Enable Background", "Get/Release Control", "Log Fuel Change", "Fuel Change Popup", "Read Inputs", "Remote Timer Reset", "Controller Change", "Get Alarms", "Init Alarms", "Save Alarms", "Voltage Selection", "Set Watlow Temp 1", "Set Watlow Temp 2", "Get Pressure", "Write Tare Pressure", "Adjust Controls", "Reinit ADC", "Write Initial Times", "Write Pumps Present", "HMI Command", "Save Pump Times", "Check Pump Stop Time", "Save LS App Config", "Init Data File", "Reset LS Cycles", "Reset Anomalies", "Reset Opens", "Save LS Data", "Save LS Test Data", "Check Serial Numbers", "Main Tab", "Allow Data Note", "Resume Profile"]
              n74 = Unbundle By Name(w284) -> ("Ignition Relay"=w281:T8)
              n75 = Not Equal?(x="Ignition Relay", y=w281) -> (x != y?=w285:bool)
              n76 = Bundle By Name(cluster=w283, "Ignition Relay"="Ignition Relay") -> (w282:T25)
            }
            frame 27 {
              n77 = Unbundle By Name(w291) -> ("HMI.HMI Mom Buttons"=w290:T21)
              n78 = Cluster To Array(cluster=w290) -> (array=w295:bool[])
              n79 = Search 1D Array(1D array=w295, element=TRUE) -> (index of element=w293:i32)  [unwired: 1 in]
              n80 = case shown="1" w293 {
                tunnel: [w297 w298 w299 w300 w301] -> w296
                frame -1, Default {
                  w297 = T14[] [] items=["Main", "Init Files", "Init", "Unused", "Save As", "Start Profile", "Check Step Time", "Alarm", "Alarm Dismiss", "Run Step", "Stop Profile", "Cycle Reset", "Time Reset", "Time Reset All", "Time Set", "Tare CTs", "Save Profile", "Open Profile", "Get Profiles", "Update Screen", "Update Controls", "Save App Config", "Write Outputs", "Disable Background", "Enable Background", "Get/Release Control", "Log Fuel Change", "Fuel Change Popup", "Read Inputs", "Remote Timer Reset", "Controller Change", "Get Alarms", "Init Alarms", "Save Alarms", "Voltage Selection", "Set Watlow Temp 1", "Set Watlow Temp 2", "Get Pressure", "Write Tare Pressure", "Adjust Controls", "Reinit ADC", "Write Initial Times", "Write Pumps Present", "HMI Command", "Save Pump Times", "Check Pump Stop Time", "Save LS App Config", "Init Data File", "Reset LS Cycles", "Reset Anomalies", "Reset Opens", "Save LS Data", "Save LS Test Data", "Check Serial Numbers", "Main Tab", "Allow Data Note", "Resume Profile"]
                }
                frame 0 {
                  w298 = T14[] [enum."Stop Profile"] items=["Main", "Init Files", "Init", "Unused", "Save As", "Start Profile", "Check Step Time", "Alarm", "Alarm Dismiss", "Run Step", "Stop Profile", "Cycle Reset", "Time Reset", "Time Reset All", "Time Set", "Tare CTs", "Save Profile", "Open Profile", "Get Profiles", "Update Screen", "Update Controls", "Save App Config", "Write Outputs", "Disable Background", "Enable Background", "Get/Release Control", "Log Fuel Change", "Fuel Change Popup", "Read Inputs", "Remote Timer Reset", "Controller Change", "Get Alarms", "Init Alarms", "Save Alarms", "Voltage Selection", "Set Watlow Temp 1", "Set Watlow Temp 2", "Get Pressure", "Write Tare Pressure", "Adjust Controls", "Reinit ADC", "Write Initial Times", "Write Pumps Present", "HMI Command", "Save Pump Times", "Check Pump Stop Time", "Save LS App Config", "Init Data File", "Reset LS Cycles", "Reset Anomalies", "Reset Opens", "Save LS Data", "Save LS Test Data", "Check Serial Numbers", "Main Tab", "Allow Data Note", "Resume Profile"]
                }
                frame 1 {
                  w299 = T14[] [enum."Remote Timer Reset"] items=["Main", "Init Files", "Init", "Unused", "Save As", "Start Profile", "Check Step Time", "Alarm", "Alarm Dismiss", "Run Step", "Stop Profile", "Cycle Reset", "Time Reset", "Time Reset All", "Time Set", "Tare CTs", "Save Profile", "Open Profile", "Get Profiles", "Update Screen", "Update Controls", "Save App Config", "Write Outputs", "Disable Background", "Enable Background", "Get/Release Control", "Log Fuel Change", "Fuel Change Popup", "Read Inputs", "Remote Timer Reset", "Controller Change", "Get Alarms", "Init Alarms", "Save Alarms", "Voltage Selection", "Set Watlow Temp 1", "Set Watlow Temp 2", "Get Pressure", "Write Tare Pressure", "Adjust Controls", "Reinit ADC", "Write Initial Times", "Write Pumps Present", "HMI Command", "Save Pump Times", "Check Pump Stop Time", "Save LS App Config", "Init Data File", "Reset LS Cycles", "Reset Anomalies", "Reset Opens", "Save LS Data", "Save LS Test Data", "Check Serial Numbers", "Main Tab", "Allow Data Note", "Resume Profile"]
                }
                frame 2 {
                  w300 = T14[] [enum."Log Fuel Change"] items=["Main", "Init Files", "Init", "Unused", "Save As", "Start Profile", "Check Step Time", "Alarm", "Alarm Dismiss", "Run Step", "Stop Profile", "Cycle Reset", "Time Reset", "Time Reset All", "Time Set", "Tare CTs", "Save Profile", "Open Profile", "Get Profiles", "Update Screen", "Update Controls", "Save App Config", "Write Outputs", "Disable Background", "Enable Background", "Get/Release Control", "Log Fuel Change", "Fuel Change Popup", "Read Inputs", "Remote Timer Reset", "Controller Change", "Get Alarms", "Init Alarms", "Save Alarms", "Voltage Selection", "Set Watlow Temp 1", "Set Watlow Temp 2", "Get Pressure", "Write Tare Pressure", "Adjust Controls", "Reinit ADC", "Write Initial Times", "Write Pumps Present", "HMI Command", "Save Pump Times", "Check Pump Stop Time", "Save LS App Config", "Init Data File", "Reset LS Cycles", "Reset Anomalies", "Reset Opens", "Save LS Data", "Save LS Test Data", "Check Serial Numbers", "Main Tab", "Allow Data Note", "Resume Profile"]
                }
                frame 3 {
                  w301 = T14[] [enum."Alarm Dismiss"] items=["Main", "Init Files", "Init", "Unused", "Save As", "Start Profile", "Check Step Time", "Alarm", "Alarm Dismiss", "Run Step", "Stop Profile", "Cycle Reset", "Time Reset", "Time Reset All", "Time Set", "Tare CTs", "Save Profile", "Open Profile", "Get Profiles", "Update Screen", "Update Controls", "Save App Config", "Write Outputs", "Disable Background", "Enable Background", "Get/Release Control", "Log Fuel Change", "Fuel Change Popup", "Read Inputs", "Remote Timer Reset", "Controller Change", "Get Alarms", "Init Alarms", "Save Alarms", "Voltage Selection", "Set Watlow Temp 1", "Set Watlow Temp 2", "Get Pressure", "Write Tare Pressure", "Adjust Controls", "Reinit ADC", "Write Initial Times", "Write Pumps Present", "HMI Command", "Save Pump Times", "Check Pump Stop Time", "Save LS App Config", "Init Data File", "Reset LS Cycles", "Reset Anomalies", "Reset Opens", "Save LS Data", "Save LS Test Data", "Check Serial Numbers", "Main Tab", "Allow Data Note", "Resume Profile"]
                }
              }
              n81 = Greater Or Equal To 0?(x=w293) -> (x >= 0?=w292:bool)
              n82 = Bundle By Name(cluster=w289, "HMI.HMI Mom Buttons"=T21 {"Stop"=FALSE, "Reset Timers"=FALSE, "Log Fuel Change"=FALSE, "Alarm Dismiss"=FALSE}) -> (w288:T25)
            }
            frame 28 {
              w308 = T14[] [enum."Save Alarms"] items=["Main", "Init Files", "Init", "Unused", "Save As", "Start Profile", "Check Step Time", "Alarm", "Alarm Dismiss", "Run Step", "Stop Profile", "Cycle Reset", "Time Reset", "Time Reset All", "Time Set", "Tare CTs", "Save Profile", "Open Profile", "Get Profiles", "Update Screen", "Update Controls", "Save App Config", "Write Outputs", "Disable Background", "Enable Background", "Get/Release Control", "Log Fuel Change", "Fuel Change Popup", "Read Inputs", "Remote Timer Reset", "Controller Change", "Get Alarms", "Init Alarms", "Save Alarms", "Voltage Selection", "Set Watlow Temp 1", "Set Watlow Temp 2", "Get Pressure", "Write Tare Pressure", "Adjust Controls", "Reinit ADC", "Write Initial Times", "Write Pumps Present", "HMI Command", "Save Pump Times", "Check Pump Stop Time", "Save LS App Config", "Init Data File", "Reset LS Cycles", "Reset Anomalies", "Reset Opens", "Save LS Data", "Save LS Test Data", "Check Serial Numbers", "Main Tab", "Allow Data Note", "Resume Profile"]
              n83 = Unbundle By Name(w306) -> ("Alarm Config"=w303:T10)
              n84 = Not Equal?(x="Alarm Config", y=w303) -> (x != y?=w307:bool)
              n85 = Bundle By Name(cluster=w305, "Alarm Config"="Alarm Config") -> (w304:T25)
            }
            frame 29 {
              w315 = T14[] [enum."Set Watlow Temp 1", enum."Save App Config"] items=["Main", "Init Files", "Init", "Unused", "Save As", "Start Profile", "Check Step Time", "Alarm", "Alarm Dismiss", "Run Step", "Stop Profile", "Cycle Reset", "Time Reset", "Time Reset All", "Time Set", "Tare CTs", "Save Profile", "Open Profile", "Get Profiles", "Update Screen", "Update Controls", "Save App Config", "Write Outputs", "Disable Background", "Enable Background", "Get/Release Control", "Log Fuel Change", "Fuel Change Popup", "Read Inputs", "Remote Timer Reset", "Controller Change", "Get Alarms", "Init Alarms", "Save Alarms", "Voltage Selection", "Set Watlow Temp 1", "Set Watlow Temp 2", "Get Pressure", "Write Tare Pressure", "Adjust Controls", "Reinit ADC", "Write Initial Times", "Write Pumps Present", "HMI Command", "Save Pump Times", "Check Pump Stop Time", "Save LS App Config", "Init Data File", "Reset LS Cycles", "Reset Anomalies", "Reset Opens", "Save LS Data", "Save LS Test Data", "Check Serial Numbers", "Main Tab", "Allow Data Note", "Resume Profile"]
              n86 = Unbundle By Name(w314) -> ("Tank CMDs.Temp 1 CMD"=w311:dbl)
              n87 = Not Equal?(x="Tank 1 Temp Cmd:", y=w311) -> (x != y?=w309:bool)
              n88 = Bundle By Name(cluster=w313, "Tank CMDs.Temp 1 CMD"="Tank 1 Temp Cmd:", "App Config.Temp 1"="Tank 1 Temp Cmd:") -> (w312:T25)
            }
            frame 30 {
              w322 = T14[] [enum."Set Watlow Temp 2", enum."Save App Config"] items=["Main", "Init Files", "Init", "Unused", "Save As", "Start Profile", "Check Step Time", "Alarm", "Alarm Dismiss", "Run Step", "Stop Profile", "Cycle Reset", "Time Reset", "Time Reset All", "Time Set", "Tare CTs", "Save Profile", "Open Profile", "Get Profiles", "Update Screen", "Update Controls", "Save App Config", "Write Outputs", "Disable Background", "Enable Background", "Get/Release Control", "Log Fuel Change", "Fuel Change Popup", "Read Inputs", "Remote Timer Reset", "Controller Change", "Get Alarms", "Init Alarms", "Save Alarms", "Voltage Selection", "Set Watlow Temp 1", "Set Watlow Temp 2", "Get Pressure", "Write Tare Pressure", "Adjust Controls", "Reinit ADC", "Write Initial Times", "Write Pumps Present", "HMI Command", "Save Pump Times", "Check Pump Stop Time", "Save LS App Config", "Init Data File", "Reset LS Cycles", "Reset Anomalies", "Reset Opens", "Save LS Data", "Save LS Test Data", "Check Serial Numbers", "Main Tab", "Allow Data Note", "Resume Profile"]
              n89 = Unbundle By Name(w321) -> ("Tank CMDs.Temp 2 CMD"=w318:dbl)
              n90 = Not Equal?(x="Tank 2 Temp Cmd:", y=w318) -> (x != y?=w316:bool)
              n91 = Bundle By Name(cluster=w320, "Tank CMDs.Temp 2 CMD"="Tank 2 Temp Cmd:", "App Config.Temp 2"="Tank 2 Temp Cmd:") -> (w319:T25)
            }
            frame 31 {
              w325 = T14[] [enum."Alarm Dismiss"] items=["Main", "Init Files", "Init", "Unused", "Save As", "Start Profile", "Check Step Time", "Alarm", "Alarm Dismiss", "Run Step", "Stop Profile", "Cycle Reset", "Time Reset", "Time Reset All", "Time Set", "Tare CTs", "Save Profile", "Open Profile", "Get Profiles", "Update Screen", "Update Controls", "Save App Config", "Write Outputs", "Disable Background", "Enable Background", "Get/Release Control", "Log Fuel Change", "Fuel Change Popup", "Read Inputs", "Remote Timer Reset", "Controller Change", "Get Alarms", "Init Alarms", "Save Alarms", "Voltage Selection", "Set Watlow Temp 1", "Set Watlow Temp 2", "Get Pressure", "Write Tare Pressure", "Adjust Controls", "Reinit ADC", "Write Initial Times", "Write Pumps Present", "HMI Command", "Save Pump Times", "Check Pump Stop Time", "Save LS App Config", "Init Data File", "Reset LS Cycles", "Reset Anomalies", "Reset Opens", "Save LS Data", "Save LS Test Data", "Check Serial Numbers", "Main Tab", "Allow Data Note", "Resume Profile"]
            }
            frame 32 {
              w328 = T14[] [enum."Get Pressure"] items=["Main", "Init Files", "Init", "Unused", "Save As", "Start Profile", "Check Step Time", "Alarm", "Alarm Dismiss", "Run Step", "Stop Profile", "Cycle Reset", "Time Reset", "Time Reset All", "Time Set", "Tare CTs", "Save Profile", "Open Profile", "Get Profiles", "Update Screen", "Update Controls", "Save App Config", "Write Outputs", "Disable Background", "Enable Background", "Get/Release Control", "Log Fuel Change", "Fuel Change Popup", "Read Inputs", "Remote Timer Reset", "Controller Change", "Get Alarms", "Init Alarms", "Save Alarms", "Voltage Selection", "Set Watlow Temp 1", "Set Watlow Temp 2", "Get Pressure", "Write Tare Pressure", "Adjust Controls", "Reinit ADC", "Write Initial Times", "Write Pumps Present", "HMI Command", "Save Pump Times", "Check Pump Stop Time", "Save LS App Config", "Init Data File", "Reset LS Cycles", "Reset Anomalies", "Reset Opens", "Save LS Data", "Save LS Test Data", "Check Serial Numbers", "Main Tab", "Allow Data Note", "Resume Profile"]
            }
            frame 33 {
              w330 = T14[] [enum."Save App Config"] items=["Main", "Init Files", "Init", "Unused", "Save As", "Start Profile", "Check Step Time", "Alarm", "Alarm Dismiss", "Run Step", "Stop Profile", "Cycle Reset", "Time Reset", "Time Reset All", "Time Set", "Tare CTs", "Save Profile", "Open Profile", "Get Profiles", "Update Screen", "Update Controls", "Save App Config", "Write Outputs", "Disable Background", "Enable Background", "Get/Release Control", "Log Fuel Change", "Fuel Change Popup", "Read Inputs", "Remote Timer Reset", "Controller Change", "Get Alarms", "Init Alarms", "Save Alarms", "Voltage Selection", "Set Watlow Temp 1", "Set Watlow Temp 2", "Get Pressure", "Write Tare Pressure", "Adjust Controls", "Reinit ADC", "Write Initial Times", "Write Pumps Present", "HMI Command", "Save Pump Times", "Check Pump Stop Time", "Save LS App Config", "Init Data File", "Reset LS Cycles", "Reset Anomalies", "Reset Opens", "Save LS Data", "Save LS Test Data", "Check Serial Numbers", "Main Tab", "Allow Data Note", "Resume Profile"]
              n92 = Unbundle By Name(w335) -> ("App Config.V_Run PI?"=w332:bool)
              n93 = Not Equal?(x="Closed Loop Voltage", y=w332) -> (x != y?=w331:bool)
              n94 = Bundle By Name(cluster=w334, "App Config.V_Run PI?"="Closed Loop Voltage") -> (w333:T25)
            }
            frame 34 {
              w340 = T14[] [enum."Adjust Controls", enum."Save App Config"] items=["Main", "Init Files", "Init", "Unused", "Save As", "Start Profile", "Check Step Time", "Alarm", "Alarm Dismiss", "Run Step", "Stop Profile", "Cycle Reset", "Time Reset", "Time Reset All", "Time Set", "Tare CTs", "Save Profile", "Open Profile", "Get Profiles", "Update Screen", "Update Controls", "Save App Config", "Write Outputs", "Disable Background", "Enable Background", "Get/Release Control", "Log Fuel Change", "Fuel Change Popup", "Read Inputs", "Remote Timer Reset", "Controller Change", "Get Alarms", "Init Alarms", "Save Alarms", "Voltage Selection", "Set Watlow Temp 1", "Set Watlow Temp 2", "Get Pressure", "Write Tare Pressure", "Adjust Controls", "Reinit ADC", "Write Initial Times", "Write Pumps Present", "HMI Command", "Save Pump Times", "Check Pump Stop Time", "Save LS App Config", "Init Data File", "Reset LS Cycles", "Reset Anomalies", "Reset Opens", "Save LS Data", "Save LS Test Data", "Check Serial Numbers", "Main Tab", "Allow Data Note", "Resume Profile"]
              n95 = Unbundle By Name(w344) -> ("App Config.Voltage Limits"=w341:T41)
              n96 = Not Equal?(x="Voltage Limits", y=w341) -> (x != y?=w337:cluster{bool, bool, bool})
              n97 = Cluster To Array(cluster=w337) -> (array=w338:bool[])
              n98 = Or Array Elements(Boolean array=w338) -> (logical OR=w336:bool)
              n99 = Bundle By Name(cluster=w343, "App Config.Voltage Limits"="Voltage Limits") -> (w342:T25)
            }
            frame 35 {
              w345 = T14[] [enum."Adjust Controls", enum."Save App Config"] items=["Main", "Init Files", "Init", "Unused", "Save As", "Start Profile", "Check Step Time", "Alarm", "Alarm Dismiss", "Run Step", "Stop Profile", "Cycle Reset", "Time Reset", "Time Reset All", "Time Set", "Tare CTs", "Save Profile", "Open Profile", "Get Profiles", "Update Screen", "Update Controls", "Save App Config", "Write Outputs", "Disable Background", "Enable Background", "Get/Release Control", "Log Fuel Change", "Fuel Change Popup", "Read Inputs", "Remote Timer Reset", "Controller Change", "Get Alarms", "Init Alarms", "Save Alarms", "Voltage Selection", "Set Watlow Temp 1", "Set Watlow Temp 2", "Get Pressure", "Write Tare Pressure", "Adjust Controls", "Reinit ADC", "Write Initial Times", "Write Pumps Present", "HMI Command", "Save Pump Times", "Check Pump Stop Time", "Save LS App Config", "Init Data File", "Reset LS Cycles", "Reset Anomalies", "Reset Opens", "Save LS Data", "Save LS Test Data", "Check Serial Numbers", "Main Tab", "Allow Data Note", "Resume Profile"]
              n100 = Unbundle By Name(w353) -> ("App Config.Voltage Far PI"=w350:T42)
              n101 = Not Equal?(x="Far PI", y=w350) -> (x != y?=w347:cluster{bool, bool, bool})
              n102 = Cluster To Array(cluster=w347) -> (array=w348:bool[])
              n103 = Or Array Elements(Boolean array=w348) -> (logical OR=w346:bool)
              n104 = Bundle By Name(cluster=w352, "App Config.Voltage Far PI"="Far PI") -> (w351:T25)
            }
            frame 36 {
              w354 = T14[] [enum."Adjust Controls", enum."Save App Config"] items=["Main", "Init Files", "Init", "Unused", "Save As", "Start Profile", "Check Step Time", "Alarm", "Alarm Dismiss", "Run Step", "Stop Profile", "Cycle Reset", "Time Reset", "Time Reset All", "Time Set", "Tare CTs", "Save Profile", "Open Profile", "Get Profiles", "Update Screen", "Update Controls", "Save App Config", "Write Outputs", "Disable Background", "Enable Background", "Get/Release Control", "Log Fuel Change", "Fuel Change Popup", "Read Inputs", "Remote Timer Reset", "Controller Change", "Get Alarms", "Init Alarms", "Save Alarms", "Voltage Selection", "Set Watlow Temp 1", "Set Watlow Temp 2", "Get Pressure", "Write Tare Pressure", "Adjust Controls", "Reinit ADC", "Write Initial Times", "Write Pumps Present", "HMI Command", "Save Pump Times", "Check Pump Stop Time", "Save LS App Config", "Init Data File", "Reset LS Cycles", "Reset Anomalies", "Reset Opens", "Save LS Data", "Save LS Test Data", "Check Serial Numbers", "Main Tab", "Allow Data Note", "Resume Profile"]
              n105 = Unbundle By Name(w362) -> ("App Config.Voltage Mid PI"=w359:T43)
              n106 = Not Equal?(x="Mid PI", y=w359) -> (x != y?=w357:cluster{bool, bool, bool})
              n107 = Cluster To Array(cluster=w357) -> (array=w358:bool[])
              n108 = Or Array Elements(Boolean array=w358) -> (logical OR=w356:bool)
              n109 = Bundle By Name(cluster=w361, "App Config.Voltage Mid PI"="Mid PI") -> (w360:T25)
            }
            frame 37 {
              w363 = T14[] [enum."Adjust Controls", enum."Save App Config"] items=["Main", "Init Files", "Init", "Unused", "Save As", "Start Profile", "Check Step Time", "Alarm", "Alarm Dismiss", "Run Step", "Stop Profile", "Cycle Reset", "Time Reset", "Time Reset All", "Time Set", "Tare CTs", "Save Profile", "Open Profile", "Get Profiles", "Update Screen", "Update Controls", "Save App Config", "Write Outputs", "Disable Background", "Enable Background", "Get/Release Control", "Log Fuel Change", "Fuel Change Popup", "Read Inputs", "Remote Timer Reset", "Controller Change", "Get Alarms", "Init Alarms", "Save Alarms", "Voltage Selection", "Set Watlow Temp 1", "Set Watlow Temp 2", "Get Pressure", "Write Tare Pressure", "Adjust Controls", "Reinit ADC", "Write Initial Times", "Write Pumps Present", "HMI Command", "Save Pump Times", "Check Pump Stop Time", "Save LS App Config", "Init Data File", "Reset LS Cycles", "Reset Anomalies", "Reset Opens", "Save LS Data", "Save LS Test Data", "Check Serial Numbers", "Main Tab", "Allow Data Note", "Resume Profile"]
              n110 = Unbundle By Name(w371) -> ("App Config.Voltage Close PI"=w368:T44)
              n111 = Not Equal?(x="Close PI", y=w368) -> (x != y?=w366:cluster{bool, bool, bool})
              n112 = Cluster To Array(cluster=w366) -> (array=w367:bool[])
              n113 = Or Array Elements(Boolean array=w367) -> (logical OR=w365:bool)
              n114 = Bundle By Name(cluster=w370, "App Config.Voltage Close PI"="Close PI") -> (w369:T25)
            }
            frame 38 {
              w372 = T14[] [enum."Adjust Controls", enum."Save App Config"] items=["Main", "Init Files", "Init", "Unused", "Save As", "Start Profile", "Check Step Time", "Alarm", "Alarm Dismiss", "Run Step", "Stop Profile", "Cycle Reset", "Time Reset", "Time Reset All", "Time Set", "Tare CTs", "Save Profile", "Open Profile", "Get Profiles", "Update Screen", "Update Controls", "Save App Config", "Write Outputs", "Disable Background", "Enable Background", "Get/Release Control", "Log Fuel Change", "Fuel Change Popup", "Read Inputs", "Remote Timer Reset", "Controller Change", "Get Alarms", "Init Alarms", "Save Alarms", "Voltage Selection", "Set Watlow Temp 1", "Set Watlow Temp 2", "Get Pressure", "Write Tare Pressure", "Adjust Controls", "Reinit ADC", "Write Initial Times", "Write Pumps Present", "HMI Command", "Save Pump Times", "Check Pump Stop Time", "Save LS App Config", "Init Data File", "Reset LS Cycles", "Reset Anomalies", "Reset Opens", "Save LS Data", "Save LS Test Data", "Check Serial Numbers", "Main Tab", "Allow Data Note", "Resume Profile"]
              n115 = Unbundle By Name(w380) -> ("App Config.Voltage Scale"=w377:cluster{"V_FFm":dbl, "V_FFb":dbl})
              n116 = Not Equal?(x="Voltage Scale", y=w377) -> (x != y?=w375:cluster{bool, bool})
              n117 = Cluster To Array(cluster=w375) -> (array=w374:bool[])
              n118 = Or Array Elements(Boolean array=w374) -> (logical OR=w373:bool)
              n119 = Bundle By Name(cluster=w379, "App Config.Voltage Scale"="Voltage Scale") -> (w378:T25)
            }
            frame 39 {
              w381 = T14[] [enum."Adjust Controls", enum."Save App Config"] items=["Main", "Init Files", "Init", "Unused", "Save As", "Start Profile", "Check Step Time", "Alarm", "Alarm Dismiss", "Run Step", "Stop Profile", "Cycle Reset", "Time Reset", "Time Reset All", "Time Set", "Tare CTs", "Save Profile", "Open Profile", "Get Profiles", "Update Screen", "Update Controls", "Save App Config", "Write Outputs", "Disable Background", "Enable Background", "Get/Release Control", "Log Fuel Change", "Fuel Change Popup", "Read Inputs", "Remote Timer Reset", "Controller Change", "Get Alarms", "Init Alarms", "Save Alarms", "Voltage Selection", "Set Watlow Temp 1", "Set Watlow Temp 2", "Get Pressure", "Write Tare Pressure", "Adjust Controls", "Reinit ADC", "Write Initial Times", "Write Pumps Present", "HMI Command", "Save Pump Times", "Check Pump Stop Time", "Save LS App Config", "Init Data File", "Reset LS Cycles", "Reset Anomalies", "Reset Opens", "Save LS Data", "Save LS Test Data", "Check Serial Numbers", "Main Tab", "Allow Data Note", "Resume Profile"]
              n120 = Unbundle By Name(w389) -> ("App Config.Voltage Cutoffs"=w386:cluster{"V_MidCutoff":dbl, "V_CloseCutoff":dbl})
              n121 = Not Equal?(x="Cutoffs", y=w386) -> (x != y?=w385:cluster{bool, bool})
              n122 = Cluster To Array(cluster=w385) -> (array=w384:bool[])
              n123 = Or Array Elements(Boolean array=w384) -> (logical OR=w383:bool)
              n124 = Bundle By Name(cluster=w388, "App Config.Voltage Cutoffs"="Cutoffs") -> (w387:T25)
            }
            frame 40 {
              w394 = T14[] [enum."Save App Config"] items=["Main", "Init Files", "Init", "Unused", "Save As", "Start Profile", "Check Step Time", "Alarm", "Alarm Dismiss", "Run Step", "Stop Profile", "Cycle Reset", "Time Reset", "Time Reset All", "Time Set", "Tare CTs", "Save Profile", "Open Profile", "Get Profiles", "Update Screen", "Update Controls", "Save App Config", "Write Outputs", "Disable Background", "Enable Background", "Get/Release Control", "Log Fuel Change", "Fuel Change Popup", "Read Inputs", "Remote Timer Reset", "Controller Change", "Get Alarms", "Init Alarms", "Save Alarms", "Voltage Selection", "Set Watlow Temp 1", "Set Watlow Temp 2", "Get Pressure", "Write Tare Pressure", "Adjust Controls", "Reinit ADC", "Write Initial Times", "Write Pumps Present", "HMI Command", "Save Pump Times", "Check Pump Stop Time", "Save LS App Config", "Init Data File", "Reset LS Cycles", "Reset Anomalies", "Reset Opens", "Save LS Data", "Save LS Test Data", "Check Serial Numbers", "Main Tab", "Allow Data Note", "Resume Profile"]
              n125 = Unbundle By Name(w398) -> ("App Config.Pressure Scale"=w395:cluster{"Pres_FFm":dbl, "Pres_FFb":dbl})
              n126 = Not Equal?(x="Pressure Scale", y=w395) -> (x != y?=w393:cluster{bool, bool})
              n127 = Cluster To Array(cluster=w393) -> (array=w392:bool[])
              n128 = Or Array Elements(Boolean array=w392) -> (logical OR=w391:bool)
              n129 = Bundle By Name(cluster=w397, "App Config.Pressure Scale"="Pressure Scale") -> (w396:T25)
            }
            frame 41 {
              w402 = T14[] [enum."Save App Config"] items=["Main", "Init Files", "Init", "Unused", "Save As", "Start Profile", "Check Step Time", "Alarm", "Alarm Dismiss", "Run Step", "Stop Profile", "Cycle Reset", "Time Reset", "Time Reset All", "Time Set", "Tare CTs", "Save Profile", "Open Profile", "Get Profiles", "Update Screen", "Update Controls", "Save App Config", "Write Outputs", "Disable Background", "Enable Background", "Get/Release Control", "Log Fuel Change", "Fuel Change Popup", "Read Inputs", "Remote Timer Reset", "Controller Change", "Get Alarms", "Init Alarms", "Save Alarms", "Voltage Selection", "Set Watlow Temp 1", "Set Watlow Temp 2", "Get Pressure", "Write Tare Pressure", "Adjust Controls", "Reinit ADC", "Write Initial Times", "Write Pumps Present", "HMI Command", "Save Pump Times", "Check Pump Stop Time", "Save LS App Config", "Init Data File", "Reset LS Cycles", "Reset Anomalies", "Reset Opens", "Save LS Data", "Save LS Test Data", "Check Serial Numbers", "Main Tab", "Allow Data Note", "Resume Profile"]
              n130 = Unbundle By Name(w406) -> ("App Config.Temp Format"=w403:i32)
              n131 = To Long Integer(number="Thermocouple") -> (32bit integer=w399:i32)
              n132 = Not Equal?(x=w399, y=w403) -> (x != y?=w401:bool)
              n133 = Bundle By Name(cluster=w405, "App Config.Temp Format"=w399) -> (w404:T25)
            }
            frame 42 {
              w409 = T14[] [enum."Save App Config"] items=["Main", "Init Files", "Init", "Unused", "Save As", "Start Profile", "Check Step Time", "Alarm", "Alarm Dismiss", "Run Step", "Stop Profile", "Cycle Reset", "Time Reset", "Time Reset All", "Time Set", "Tare CTs", "Save Profile", "Open Profile", "Get Profiles", "Update Screen", "Update Controls", "Save App Config", "Write Outputs", "Disable Background", "Enable Background", "Get/Release Control", "Log Fuel Change", "Fuel Change Popup", "Read Inputs", "Remote Timer Reset", "Controller Change", "Get Alarms", "Init Alarms", "Save Alarms", "Voltage Selection", "Set Watlow Temp 1", "Set Watlow Temp 2", "Get Pressure", "Write Tare Pressure", "Adjust Controls", "Reinit ADC", "Write Initial Times", "Write Pumps Present", "HMI Command", "Save Pump Times", "Check Pump Stop Time", "Save LS App Config", "Init Data File", "Reset LS Cycles", "Reset Anomalies", "Reset Opens", "Save LS Data", "Save LS Test Data", "Check Serial Numbers", "Main Tab", "Allow Data Note", "Resume Profile"]
              n134 = Unbundle By Name(w413) -> ("App Config.Temp Tolerance"=w410:dbl)
              n135 = Not Equal?(x="Temp Tolerance", y=w410) -> (x != y?=w407:bool)
              n136 = Bundle By Name(cluster=w412, "App Config.Temp Tolerance"="Temp Tolerance") -> (w411:T25)
            }
            frame 43 {
              w420 = T14[] [enum."Save App Config"] items=["Main", "Init Files", "Init", "Unused", "Save As", "Start Profile", "Check Step Time", "Alarm", "Alarm Dismiss", "Run Step", "Stop Profile", "Cycle Reset", "Time Reset", "Time Reset All", "Time Set", "Tare CTs", "Save Profile", "Open Profile", "Get Profiles", "Update Screen", "Update Controls", "Save App Config", "Write Outputs", "Disable Background", "Enable Background", "Get/Release Control", "Log Fuel Change", "Fuel Change Popup", "Read Inputs", "Remote Timer Reset", "Controller Change", "Get Alarms", "Init Alarms", "Save Alarms", "Voltage Selection", "Set Watlow Temp 1", "Set Watlow Temp 2", "Get Pressure", "Write Tare Pressure", "Adjust Controls", "Reinit ADC", "Write Initial Times", "Write Pumps Present", "HMI Command", "Save Pump Times", "Check Pump Stop Time", "Save LS App Config", "Init Data File", "Reset LS Cycles", "Reset Anomalies", "Reset Opens", "Save LS Data", "Save LS Test Data", "Check Serial Numbers", "Main Tab", "Allow Data Note", "Resume Profile"]
              n137 = Unbundle By Name(w417) -> ("App Config.Target Voltage"=w416:dbl)
              n138 = Not Equal?(x=w416, y="Target Voltage:") -> (x != y?=w415:bool)
              n139 = Bundle By Name(cluster=w419, "App Config.Target Voltage"="Target Voltage:") -> (w418:T25)
            }
            frame 44 {
              w427 = T14[] [enum."Save App Config"] items=["Main", "Init Files", "Init", "Unused", "Save As", "Start Profile", "Check Step Time", "Alarm", "Alarm Dismiss", "Run Step", "Stop Profile", "Cycle Reset", "Time Reset", "Time Reset All", "Time Set", "Tare CTs", "Save Profile", "Open Profile", "Get Profiles", "Update Screen", "Update Controls", "Save App Config", "Write Outputs", "Disable Background", "Enable Background", "Get/Release Control", "Log Fuel Change", "Fuel Change Popup", "Read Inputs", "Remote Timer Reset", "Controller Change", "Get Alarms", "Init Alarms", "Save Alarms", "Voltage Selection", "Set Watlow Temp 1", "Set Watlow Temp 2", "Get Pressure", "Write Tare Pressure", "Adjust Controls", "Reinit ADC", "Write Initial Times", "Write Pumps Present", "HMI Command", "Save Pump Times", "Check Pump Stop Time", "Save LS App Config", "Init Data File", "Reset LS Cycles", "Reset Anomalies", "Reset Opens", "Save LS Data", "Save LS Test Data", "Check Serial Numbers", "Main Tab", "Allow Data Note", "Resume Profile"]
              n140 = Unbundle By Name(w424) -> ("App Config.Target Pressure"=w423:dbl)
              n141 = Not Equal?(x=w423, y="Target Pressure:") -> (x != y?=w422:bool)
              n142 = Bundle By Name(cluster=w426, "App Config.Target Pressure"="Target Pressure:") -> (w425:T25)
            }
            frame 45 {
              w431 = T14[] [enum."HMI Command"] items=["Main", "Init Files", "Init", "Unused", "Save As", "Start Profile", "Check Step Time", "Alarm", "Alarm Dismiss", "Run Step", "Stop Profile", "Cycle Reset", "Time Reset", "Time Reset All", "Time Set", "Tare CTs", "Save Profile", "Open Profile", "Get Profiles", "Update Screen", "Update Controls", "Save App Config", "Write Outputs", "Disable Background", "Enable Background", "Get/Release Control", "Log Fuel Change", "Fuel Change Popup", "Read Inputs", "Remote Timer Reset", "Controller Change", "Get Alarms", "Init Alarms", "Save Alarms", "Voltage Selection", "Set Watlow Temp 1", "Set Watlow Temp 2", "Get Pressure", "Write Tare Pressure", "Adjust Controls", "Reinit ADC", "Write Initial Times", "Write Pumps Present", "HMI Command", "Save Pump Times", "Check Pump Stop Time", "Save LS App Config", "Init Data File", "Reset LS Cycles", "Reset Anomalies", "Reset Opens", "Save LS Data", "Save LS Test Data", "Check Serial Numbers", "Main Tab", "Allow Data Note", "Resume Profile"]
              n143 = call "RPi HMI Global.vi"() -> ("HMI Cluster OUT"=w430:T16)  [unwired: 11 in]
              n144 = Unbundle By Name(w430) -> ("HMI Command"=w428:bool)
            }
            frame 46 {
              w438 = T14[] [enum."Update Controls"] items=["Main", "Init Files", "Init", "Unused", "Save As", "Start Profile", "Check Step Time", "Alarm", "Alarm Dismiss", "Run Step", "Stop Profile", "Cycle Reset", "Time Reset", "Time Reset All", "Time Set", "Tare CTs", "Save Profile", "Open Profile", "Get Profiles", "Update Screen", "Update Controls", "Save App Config", "Write Outputs", "Disable Background", "Enable Background", "Get/Release Control", "Log Fuel Change", "Fuel Change Popup", "Read Inputs", "Remote Timer Reset", "Controller Change", "Get Alarms", "Init Alarms", "Save Alarms", "Voltage Selection", "Set Watlow Temp 1", "Set Watlow Temp 2", "Get Pressure", "Write Tare Pressure", "Adjust Controls", "Reinit ADC", "Write Initial Times", "Write Pumps Present", "HMI Command", "Save Pump Times", "Check Pump Stop Time", "Save LS App Config", "Init Data File", "Reset LS Cycles", "Reset Anomalies", "Reset Opens", "Save LS Data", "Save LS Test Data", "Check Serial Numbers", "Main Tab", "Allow Data Note", "Resume Profile"]
              n145 = Unbundle By Name(w437) -> ("Email Alarms Disabled"=w434:bool)
              n146 = Greater?(x="Disable Alarm Email", y=w434) -> (0:w432:bool)
              n147 = Bundle By Name(cluster=w436, "Email Alarms Disabled"="Disable Alarm Email") -> (w435:T25)
            }
            frame 47 {
              w443 = T14[] [] items=["Main", "Init Files", "Init", "Unused", "Save As", "Start Profile", "Check Step Time", "Alarm", "Alarm Dismiss", "Run Step", "Stop Profile", "Cycle Reset", "Time Reset", "Time Reset All", "Time Set", "Tare CTs", "Save Profile", "Open Profile", "Get Profiles", "Update Screen", "Update Controls", "Save App Config", "Write Outputs", "Disable Background", "Enable Background", "Get/Release Control", "Log Fuel Change", "Fuel Change Popup", "Read Inputs", "Remote Timer Reset", "Controller Change", "Get Alarms", "Init Alarms", "Save Alarms", "Voltage Selection", "Set Watlow Temp 1", "Set Watlow Temp 2", "Get Pressure", "Write Tare Pressure", "Adjust Controls", "Reinit ADC", "Write Initial Times", "Write Pumps Present", "HMI Command", "Save Pump Times", "Check Pump Stop Time", "Save LS App Config", "Init Data File", "Reset LS Cycles", "Reset Anomalies", "Reset Opens", "Save LS Data", "Save LS Test Data", "Check Serial Numbers", "Main Tab", "Allow Data Note", "Resume Profile"]
              n148 = Bundle By Name(cluster=w442, "Concat Data"="Concat Data") -> (w441:T25)
            }
            frame 48 {
              w448 = T14[] [] items=["Main", "Init Files", "Init", "Unused", "Save As", "Start Profile", "Check Step Time", "Alarm", "Alarm Dismiss", "Run Step", "Stop Profile", "Cycle Reset", "Time Reset", "Time Reset All", "Time Set", "Tare CTs", "Save Profile", "Open Profile", "Get Profiles", "Update Screen", "Update Controls", "Save App Config", "Write Outputs", "Disable Background", "Enable Background", "Get/Release Control", "Log Fuel Change", "Fuel Change Popup", "Read Inputs", "Remote Timer Reset", "Controller Change", "Get Alarms", "Init Alarms", "Save Alarms", "Voltage Selection", "Set Watlow Temp 1", "Set Watlow Temp 2", "Get Pressure", "Write Tare Pressure", "Adjust Controls", "Reinit ADC", "Write Initial Times", "Write Pumps Present", "HMI Command", "Save Pump Times", "Check Pump Stop Time", "Save LS App Config", "Init Data File", "Reset LS Cycles", "Reset Anomalies", "Reset Opens", "Save LS Data", "Save LS Test Data", "Check Serial Numbers", "Main Tab", "Allow Data Note", "Resume Profile"]
              n149 = Bundle By Name(cluster=w447, "WebDAV Push"="WebDAV Push") -> (w446:T25)
            }
            frame 49 {
              w455 = T14[] [enum."Save App Config"] items=["Main", "Init Files", "Init", "Unused", "Save As", "Start Profile", "Check Step Time", "Alarm", "Alarm Dismiss", "Run Step", "Stop Profile", "Cycle Reset", "Time Reset", "Time Reset All", "Time Set", "Tare CTs", "Save Profile", "Open Profile", "Get Profiles", "Update Screen", "Update Controls", "Save App Config", "Write Outputs", "Disable Background", "Enable Background", "Get/Release Control", "Log Fuel Change", "Fuel Change Popup", "Read Inputs", "Remote Timer Reset", "Controller Change", "Get Alarms", "Init Alarms", "Save Alarms", "Voltage Selection", "Set Watlow Temp 1", "Set Watlow Temp 2", "Get Pressure", "Write Tare Pressure", "Adjust Controls", "Reinit ADC", "Write Initial Times", "Write Pumps Present", "HMI Command", "Save Pump Times", "Check Pump Stop Time", "Save LS App Config", "Init Data File", "Reset LS Cycles", "Reset Anomalies", "Reset Opens", "Save LS Data", "Save LS Test Data", "Check Serial Numbers", "Main Tab", "Allow Data Note", "Resume Profile"]
              n150 = Unbundle By Name(w452) -> ("App Config.Cycle Threshold:"=w450:dbl)
              n151 = Not Equal?(x=w450, y="Cycle Threshold:") -> (x != y?=w451:bool)
              n152 = Bundle By Name(cluster=w454, "App Config.Cycle Threshold:"="Cycle Threshold:") -> (w453:T25)
            }
            frame 50 {
              w462 = T14[] [enum."Save App Config"] items=["Main", "Init Files", "Init", "Unused", "Save As", "Start Profile", "Check Step Time", "Alarm", "Alarm Dismiss", "Run Step", "Stop Profile", "Cycle Reset", "Time Reset", "Time Reset All", "Time Set", "Tare CTs", "Save Profile", "Open Profile", "Get Profiles", "Update Screen", "Update Controls", "Save App Config", "Write Outputs", "Disable Background", "Enable Background", "Get/Release Control", "Log Fuel Change", "Fuel Change Popup", "Read Inputs", "Remote Timer Reset", "Controller Change", "Get Alarms", "Init Alarms", "Save Alarms", "Voltage Selection", "Set Watlow Temp 1", "Set Watlow Temp 2", "Get Pressure", "Write Tare Pressure", "Adjust Controls", "Reinit ADC", "Write Initial Times", "Write Pumps Present", "HMI Command", "Save Pump Times", "Check Pump Stop Time", "Save LS App Config", "Init Data File", "Reset LS Cycles", "Reset Anomalies", "Reset Opens", "Save LS Data", "Save LS Test Data", "Check Serial Numbers", "Main Tab", "Allow Data Note", "Resume Profile"]
              n153 = Unbundle By Name(w459) -> ("App Config.Cycle Pts to Avg:"=w457:i32)
              n154 = Not Equal?(x=w457, y="Cycle Pts to Avg:") -> (x != y?=w458:bool)
              n155 = Bundle By Name(cluster=w461, "App Config.Cycle Pts to Avg:"="Cycle Pts to Avg:") -> (w460:T25)
            }
            frame 51 {
              w469 = T14[] [enum."Save App Config", enum."Write Outputs"] items=["Main", "Init Files", "Init", "Unused", "Save As", "Start Profile", "Check Step Time", "Alarm", "Alarm Dismiss", "Run Step", "Stop Profile", "Cycle Reset", "Time Reset", "Time Reset All", "Time Set", "Tare CTs", "Save Profile", "Open Profile", "Get Profiles", "Update Screen", "Update Controls", "Save App Config", "Write Outputs", "Disable Background", "Enable Background", "Get/Release Control", "Log Fuel Change", "Fuel Change Popup", "Read Inputs", "Remote Timer Reset", "Controller Change", "Get Alarms", "Init Alarms", "Save Alarms", "Voltage Selection", "Set Watlow Temp 1", "Set Watlow Temp 2", "Get Pressure", "Write Tare Pressure", "Adjust Controls", "Reinit ADC", "Write Initial Times", "Write Pumps Present", "HMI Command", "Save Pump Times", "Check Pump Stop Time", "Save LS App Config", "Init Data File", "Reset LS Cycles", "Reset Anomalies", "Reset Opens", "Save LS Data", "Save LS Test Data", "Check Serial Numbers", "Main Tab", "Allow Data Note", "Resume Profile"]
              n156 = Unbundle By Name(w466) -> ("App Config.Step Threshold:"=w464:dbl)
              n157 = Not Equal?(x=w464, y="Step Threshold:") -> (x != y?=w465:bool)
              n158 = Bundle By Name(cluster=w468, "App Config.Step Threshold:"="Step Threshold:") -> (w467:T25)
            }
            frame 52 {
              w476 = T14[] [enum."Save App Config", enum."Write Outputs"] items=["Main", "Init Files", "Init", "Unused", "Save As", "Start Profile", "Check Step Time", "Alarm", "Alarm Dismiss", "Run Step", "Stop Profile", "Cycle Reset", "Time Reset", "Time Reset All", "Time Set", "Tare CTs", "Save Profile", "Open Profile", "Get Profiles", "Update Screen", "Update Controls", "Save App Config", "Write Outputs", "Disable Background", "Enable Background", "Get/Release Control", "Log Fuel Change", "Fuel Change Popup", "Read Inputs", "Remote Timer Reset", "Controller Change", "Get Alarms", "Init Alarms", "Save Alarms", "Voltage Selection", "Set Watlow Temp 1", "Set Watlow Temp 2", "Get Pressure", "Write Tare Pressure", "Adjust Controls", "Reinit ADC", "Write Initial Times", "Write Pumps Present", "HMI Command", "Save Pump Times", "Check Pump Stop Time", "Save LS App Config", "Init Data File", "Reset LS Cycles", "Reset Anomalies", "Reset Opens", "Save LS Data", "Save LS Test Data", "Check Serial Numbers", "Main Tab", "Allow Data Note", "Resume Profile"]
              n159 = Unbundle By Name(w473) -> ("App Config.Normal Steps:"=w471:u32)
              n160 = Not Equal?(x=w471, y="Normal Steps:") -> (x != y?=w472:bool)
              n161 = Bundle By Name(cluster=w475, "App Config.Normal Steps:"="Normal Steps:") -> (w474:T25)
            }
            frame 53 {
              w485 = T14[] [enum."Main Tab"] items=["Main", "Init Files", "Init", "Unused", "Save As", "Start Profile", "Check Step Time", "Alarm", "Alarm Dismiss", "Run Step", "Stop Profile", "Cycle Reset", "Time Reset", "Time Reset All", "Time Set", "Tare CTs", "Save Profile", "Open Profile", "Get Profiles", "Update Screen", "Update Controls", "Save App Config", "Write Outputs", "Disable Background", "Enable Background", "Get/Release Control", "Log Fuel Change", "Fuel Change Popup", "Read Inputs", "Remote Timer Reset", "Controller Change", "Get Alarms", "Init Alarms", "Save Alarms", "Voltage Selection", "Set Watlow Temp 1", "Set Watlow Temp 2", "Get Pressure", "Write Tare Pressure", "Adjust Controls", "Reinit ADC", "Write Initial Times", "Write Pumps Present", "HMI Command", "Save Pump Times", "Check Pump Stop Time", "Save LS App Config", "Init Data File", "Reset LS Cycles", "Reset Anomalies", "Reset Opens", "Save LS Data", "Save LS Test Data", "Check Serial Numbers", "Main Tab", "Allow Data Note", "Resume Profile"]
              n162 = Unbundle By Name(w490) -> ("Main Tab"=w487:T9)
              n163 = local read "Main Tab"() -> (w486:T9)
              n164 = local read "Position"() -> (w479:i32)
              n165 = local read "Pause"() -> (w481:bool)
              n166 = feedback-in #1(w479) -> ()
              n167 = feedback #1(w479) -> (w480:i32)
              n168 = feedback #2(w481) -> (w482:bool)
              n169 = feedback-in #2(w481) -> ()
              n170 = Not Equal?(x=w487, y=w486) -> (x != y?=w484:bool)
              n171 = Not Equal?(x=w480, y=w479) -> (x != y?=w478:bool)
              n172 = Greater?(x=w482, y=w481) -> (0:w477:bool)
              n173 = Compound Arithmetic op=OR(w484, w478, w477) -> (w483:bool)
              n174 = case shown="True" w483 {
                frame False {
                }
                frame True {
                  n175 = property on="Waveform Chart" class="WFChart (strict)"("History Data"=dbl[] []) -> ()  [unwired: 2 in, 2 out]
                }
              }
              n176 = Bundle By Name(cluster=w489, "Main Tab"=w486) -> (w488:T25)
            }
            frame 54 {
              w495 = T14[] [enum."Save LS App Config", enum."Write Outputs"] items=["Main", "Init Files", "Init", "Unused", "Save As", "Start Profile", "Check Step Time", "Alarm", "Alarm Dismiss", "Run Step", "Stop Profile", "Cycle Reset", "Time Reset", "Time Reset All", "Time Set", "Tare CTs", "Save Profile", "Open Profile", "Get Profiles", "Update Screen", "Update Controls", "Save App Config", "Write Outputs", "Disable Background", "Enable Background", "Get/Release Control", "Log Fuel Change", "Fuel Change Popup", "Read Inputs", "Remote Timer Reset", "Controller Change", "Get Alarms", "Init Alarms", "Save Alarms", "Voltage Selection", "Set Watlow Temp 1", "Set Watlow Temp 2", "Get Pressure", "Write Tare Pressure", "Adjust Controls", "Reinit ADC", "Write Initial Times", "Write Pumps Present", "HMI Command", "Save Pump Times", "Check Pump Stop Time", "Save LS App Config", "Init Data File", "Reset LS Cycles", "Reset Anomalies", "Reset Opens", "Save LS Data", "Save LS Test Data", "Check Serial Numbers", "Main Tab", "Allow Data Note", "Resume Profile"]
              n177 = Unbundle By Name(w498) -> ("LS App Config.LS Power (Freq):"=w494:dbl)
              n178 = Not Equal?(x=w494, y="LS Cycle Time (ms):") -> (x != y?=w492:bool)
              n179 = Bundle By Name(cluster=w497, "LS App Config.LS Power (Freq):"="LS Cycle Time (ms):") -> (w496:T25)
            }
            frame 55 {
              w502 = T14[] [enum."Save LS App Config", enum."Write Outputs"] items=["Main", "Init Files", "Init", "Unused", "Save As", "Start Profile", "Check Step Time", "Alarm", "Alarm Dismiss", "Run Step", "Stop Profile", "Cycle Reset", "Time Reset", "Time Reset All", "Time Set", "Tare CTs", "Save Profile", "Open Profile", "Get Profiles", "Update Screen", "Update Controls", "Save App Config", "Write Outputs", "Disable Background", "Enable Background", "Get/Release Control", "Log Fuel Change", "Fuel Change Popup", "Read Inputs", "Remote Timer Reset", "Controller Change", "Get Alarms", "Init Alarms", "Save Alarms", "Voltage Selection", "Set Watlow Temp 1", "Set Watlow Temp 2", "Get Pressure", "Write Tare Pressure", "Adjust Controls", "Reinit ADC", "Write Initial Times", "Write Pumps Present", "HMI Command", "Save Pump Times", "Check Pump Stop Time", "Save LS App Config", "Init Data File", "Reset LS Cycles", "Reset Anomalies", "Reset Opens", "Save LS Data", "Save LS Test Data", "Check Serial Numbers", "Main Tab", "Allow Data Note", "Resume Profile"]
              n180 = Unbundle By Name(w505) -> ("LS App Config.LS Power (Duty):"=w501:dbl)
              n181 = Not Equal?(x=w501, y="LS On Time (ms):") -> (x != y?=w500:bool)
              n182 = Bundle By Name(cluster=w504, "LS App Config.LS Power (Duty):"="LS On Time (ms):") -> (w503:T25)
            }
            frame 56 {
              w511 = T14[] [enum."Save LS App Config", enum."Write Outputs"] items=["Main", "Init Files", "Init", "Unused", "Save As", "Start Profile", "Check Step Time", "Alarm", "Alarm Dismiss", "Run Step", "Stop Profile", "Cycle Reset", "Time Reset", "Time Reset All", "Time Set", "Tare CTs", "Save Profile", "Open Profile", "Get Profiles", "Update Screen", "Update Controls", "Save App Config", "Write Outputs", "Disable Background", "Enable Background", "Get/Release Control", "Log Fuel Change", "Fuel Change Popup", "Read Inputs", "Remote Timer Reset", "Controller Change", "Get Alarms", "Init Alarms", "Save Alarms", "Voltage Selection", "Set Watlow Temp 1", "Set Watlow Temp 2", "Get Pressure", "Write Tare Pressure", "Adjust Controls", "Reinit ADC", "Write Initial Times", "Write Pumps Present", "HMI Command", "Save Pump Times", "Check Pump Stop Time", "Save LS App Config", "Init Data File", "Reset LS Cycles", "Reset Anomalies", "Reset Opens", "Save LS Data", "Save LS Test Data", "Check Serial Numbers", "Main Tab", "Allow Data Note", "Resume Profile"]
              n183 = Unbundle By Name(w514) -> ("LS App Config.Bank 1 Present"=w510:T2)
              n184 = Not Equal?(x=w510, y="Bank 1") -> (x != y?=w508:T2)
              n185 = Cluster To Array(cluster=w508) -> (array=w507:bool[])
              n186 = Or Array Elements(Boolean array=w507) -> (logical OR=w506:bool)
              n187 = Bundle By Name(cluster=w513, "LS App Config.Bank 1 Present"="Bank 1") -> (w512:T25)
            }
            frame 57 {
              w520 = T14[] [enum."Save LS App Config", enum."Write Outputs"] items=["Main", "Init Files", "Init", "Unused", "Save As", "Start Profile", "Check Step Time", "Alarm", "Alarm Dismiss", "Run Step", "Stop Profile", "Cycle Reset", "Time Reset", "Time Reset All", "Time Set", "Tare CTs", "Save Profile", "Open Profile", "Get Profiles", "Update Screen", "Update Controls", "Save App Config", "Write Outputs", "Disable Background", "Enable Background", "Get/Release Control", "Log Fuel Change", "Fuel Change Popup", "Read Inputs", "Remote Timer Reset", "Controller Change", "Get Alarms", "Init Alarms", "Save Alarms", "Voltage Selection", "Set Watlow Temp 1", "Set Watlow Temp 2", "Get Pressure", "Write Tare Pressure", "Adjust Controls", "Reinit ADC", "Write Initial Times", "Write Pumps Present", "HMI Command", "Save Pump Times", "Check Pump Stop Time", "Save LS App Config", "Init Data File", "Reset LS Cycles", "Reset Anomalies", "Reset Opens", "Save LS Data", "Save LS Test Data", "Check Serial Numbers", "Main Tab", "Allow Data Note", "Resume Profile"]
              n188 = Unbundle By Name(w523) -> ("LS App Config.Bank 2 Present"=w519:T1)
              n189 = Not Equal?(x=w519, y="Bank 2") -> (x != y?=w518:T1)
              n190 = Cluster To Array(cluster=w518) -> (array=w517:bool[])
              n191 = Or Array Elements(Boolean array=w517) -> (logical OR=w516:bool)
              n192 = Bundle By Name(cluster=w522, "LS App Config.Bank 2 Present"="Bank 2") -> (w521:T25)
            }
            frame 58 {
              w527 = T14[] [enum."Init Data File", enum."Save LS App Config"] items=["Main", "Init Files", "Init", "Unused", "Save As", "Start Profile", "Check Step Time", "Alarm", "Alarm Dismiss", "Run Step", "Stop Profile", "Cycle Reset", "Time Reset", "Time Reset All", "Time Set", "Tare CTs", "Save Profile", "Open Profile", "Get Profiles", "Update Screen", "Update Controls", "Save App Config", "Write Outputs", "Disable Background", "Enable Background", "Get/Release Control", "Log Fuel Change", "Fuel Change Popup", "Read Inputs", "Remote Timer Reset", "Controller Change", "Get Alarms", "Init Alarms", "Save Alarms", "Voltage Selection", "Set Watlow Temp 1", "Set Watlow Temp 2", "Get Pressure", "Write Tare Pressure", "Adjust Controls", "Reinit ADC", "Write Initial Times", "Write Pumps Present", "HMI Command", "Save Pump Times", "Check Pump Stop Time", "Save LS App Config", "Init Data File", "Reset LS Cycles", "Reset Anomalies", "Reset Opens", "Save LS Data", "Save LS Test Data", "Check Serial Numbers", "Main Tab", "Allow Data Note", "Resume Profile"]
              n193 = Unbundle By Name(w530) -> ("LS App Config.Data File Name:"=w526:string)
              n194 = Not Equal?(x=w526, y="Data File Name:") -> (x != y?=w525:bool)
              n195 = Bundle By Name(cluster=w529, "LS App Config.Data File Name:"="Data File Name:") -> (w528:T25)
            }
            frame 59 {
              w534 = T14[] [enum."Save LS App Config"] items=["Main", "Init Files", "Init", "Unused", "Save As", "Start Profile", "Check Step Time", "Alarm", "Alarm Dismiss", "Run Step", "Stop Profile", "Cycle Reset", "Time Reset", "Time Reset All", "Time Set", "Tare CTs", "Save Profile", "Open Profile", "Get Profiles", "Update Screen", "Update Controls", "Save App Config", "Write Outputs", "Disable Background", "Enable Background", "Get/Release Control", "Log Fuel Change", "Fuel Change Popup", "Read Inputs", "Remote Timer Reset", "Controller Change", "Get Alarms", "Init Alarms", "Save Alarms", "Voltage Selection", "Set Watlow Temp 1", "Set Watlow Temp 2", "Get Pressure", "Write Tare Pressure", "Adjust Controls", "Reinit ADC", "Write Initial Times", "Write Pumps Present", "HMI Command", "Save Pump Times", "Check Pump Stop Time", "Save LS App Config", "Init Data File", "Reset LS Cycles", "Reset Anomalies", "Reset Opens", "Save LS Data", "Save LS Test Data", "Check Serial Numbers", "Main Tab", "Allow Data Note", "Resume Profile"]
              n196 = Unbundle By Name(w537) -> ("LS App Config.Record Bursts"=w533:bool)
              n197 = Not Equal?(x=w533, y="Record During Profile") -> (x != y?=w532:bool)
              n198 = Bundle By Name(cluster=w536, "LS App Config.Record Bursts"="Record During Profile") -> (w535:T25)
            }
            frame 60 {
              w541 = T14[] [enum."Save LS App Config"] items=["Main", "Init Files", "Init", "Unused", "Save As", "Start Profile", "Check Step Time", "Alarm", "Alarm Dismiss", "Run Step", "Stop Profile", "Cycle Reset", "Time Reset", "Time Reset All", "Time Set", "Tare CTs", "Save Profile", "Open Profile", "Get Profiles", "Update Screen", "Update Controls", "Save App Config", "Write Outputs", "Disable Background", "Enable Background", "Get/Release Control", "Log Fuel Change", "Fuel Change Popup", "Read Inputs", "Remote Timer Reset", "Controller Change", "Get Alarms", "Init Alarms", "Save Alarms", "Voltage Selection", "Set Watlow Temp 1", "Set Watlow Temp 2", "Get Pressure", "Write Tare Pressure", "Adjust Controls", "Reinit ADC", "Write Initial Times", "Write Pumps Present", "HMI Command", "Save Pump Times", "Check Pump Stop Time", "Save LS App Config", "Init Data File", "Reset LS Cycles", "Reset Anomalies", "Reset Opens", "Save LS Data", "Save LS Test Data", "Check Serial Numbers", "Main Tab", "Allow Data Note", "Resume Profile"]
              n199 = Unbundle By Name(w544) -> ("LS App Config.RecInterval(s)"=w540:i32)
              n200 = Not Equal?(x=w540, y="Interval Between\nRecordings (s):") -> (x != y?=w539:bool)
              n201 = Bundle By Name(cluster=w543, "LS App Config.RecInterval(s)"="Interval Between\nRecordings (s):") -> (w542:T25)
            }
            frame 61 {
              w548 = T14[] [enum."Save LS App Config"] items=["Main", "Init Files", "Init", "Unused", "Save As", "Start Profile", "Check Step Time", "Alarm", "Alarm Dismiss", "Run Step", "Stop Profile", "Cycle Reset", "Time Reset", "Time Reset All", "Time Set", "Tare CTs", "Save Profile", "Open Profile", "Get Profiles", "Update Screen", "Update Controls", "Save App Config", "Write Outputs", "Disable Background", "Enable Background", "Get/Release Control", "Log Fuel Change", "Fuel Change Popup", "Read Inputs", "Remote Timer Reset", "Controller Change", "Get Alarms", "Init Alarms", "Save Alarms", "Voltage Selection", "Set Watlow Temp 1", "Set Watlow Temp 2", "Get Pressure", "Write Tare Pressure", "Adjust Controls", "Reinit ADC", "Write Initial Times", "Write Pumps Present", "HMI Command", "Save Pump Times", "Check Pump Stop Time", "Save LS App Config", "Init Data File", "Reset LS Cycles", "Reset Anomalies", "Reset Opens", "Save LS Data", "Save LS Test Data", "Check Serial Numbers", "Main Tab", "Allow Data Note", "Resume Profile"]
              n202 = Unbundle By Name(w551) -> ("LS App Config.RecDuration(s)"=w547:i32)
              n203 = Not Equal?(x=w547, y="Recording\nDuration (s):") -> (x != y?=w546:bool)
              n204 = Bundle By Name(cluster=w550, "LS App Config.RecDuration(s)"="Recording\nDuration (s):") -> (w549:T25)
            }
            frame 62 {
              w555 = T14[] [enum."Save LS App Config"] items=["Main", "Init Files", "Init", "Unused", "Save As", "Start Profile", "Check Step Time", "Alarm", "Alarm Dismiss", "Run Step", "Stop Profile", "Cycle Reset", "Time Reset", "Time Reset All", "Time Set", "Tare CTs", "Save Profile", "Open Profile", "Get Profiles", "Update Screen", "Update Controls", "Save App Config", "Write Outputs", "Disable Background", "Enable Background", "Get/Release Control", "Log Fuel Change", "Fuel Change Popup", "Read Inputs", "Remote Timer Reset", "Controller Change", "Get Alarms", "Init Alarms", "Save Alarms", "Voltage Selection", "Set Watlow Temp 1", "Set Watlow Temp 2", "Get Pressure", "Write Tare Pressure", "Adjust Controls", "Reinit ADC", "Write Initial Times", "Write Pumps Present", "HMI Command", "Save Pump Times", "Check Pump Stop Time", "Save LS App Config", "Init Data File", "Reset LS Cycles", "Reset Anomalies", "Reset Opens", "Save LS Data", "Save LS Test Data", "Check Serial Numbers", "Main Tab", "Allow Data Note", "Resume Profile"]
              n205 = Unbundle By Name(w558) -> ("LS App Config.RecFrequeny (Hz)"=w554:i32)
              n206 = Not Equal?(x=w554, y="Recording\nFrequency (Hz):") -> (x != y?=w553:bool)
              n207 = Bundle By Name(cluster=w557, "LS App Config.RecFrequeny (Hz)"="Recording\nFrequency (Hz):") -> (w556:T25)
            }
            frame 63 {
              w562 = T14[] [enum."Save LS App Config", enum."Write Outputs"] items=["Main", "Init Files", "Init", "Unused", "Save As", "Start Profile", "Check Step Time", "Alarm", "Alarm Dismiss", "Run Step", "Stop Profile", "Cycle Reset", "Time Reset", "Time Reset All", "Time Set", "Tare CTs", "Save Profile", "Open Profile", "Get Profiles", "Update Screen", "Update Controls", "Save App Config", "Write Outputs", "Disable Background", "Enable Background", "Get/Release Control", "Log Fuel Change", "Fuel Change Popup", "Read Inputs", "Remote Timer Reset", "Controller Change", "Get Alarms", "Init Alarms", "Save Alarms", "Voltage Selection", "Set Watlow Temp 1", "Set Watlow Temp 2", "Get Pressure", "Write Tare Pressure", "Adjust Controls", "Reinit ADC", "Write Initial Times", "Write Pumps Present", "HMI Command", "Save Pump Times", "Check Pump Stop Time", "Save LS App Config", "Init Data File", "Reset LS Cycles", "Reset Anomalies", "Reset Opens", "Save LS Data", "Save LS Test Data", "Check Serial Numbers", "Main Tab", "Allow Data Note", "Resume Profile"]
              n208 = Unbundle By Name(w565) -> ("LS App Config.DetectionMode"=w561:i32)
              n209 = Not Equal?(x=w561, y="Detection Mode:") -> (x != y?=w560:bool)
              n210 = case shown="True" w560 {
                tunnel: "Detection Mode:" -> [_ w566]
                frame False {
                }
                frame True {
                  n211 = case shown="0, Default" w566 {
                    frame 0, Default {
                      n212 = local write "Live Data Tab"(enum32{"Page 1", "Page 2", "Page 3"}."Page 2" ("Live Data Tab")) -> ()
                    }
                    frame 1 {
                      n213 = local write "Live Data Tab"(enum32{"Page 1", "Page 2", "Page 3"}."Page 3" ("Live Data Tab")) -> ()
                    }
                  }
                }
              }
              n214 = Bundle By Name(cluster=w564, "LS App Config.DetectionMode"="Detection Mode:") -> (w563:T25)
            }
            frame 64 {
              w574 = T14[] [enum."Check Serial Numbers", enum."Save LS App Config"] items=["Main", "Init Files", "Init", "Unused", "Save As", "Start Profile", "Check Step Time", "Alarm", "Alarm Dismiss", "Run Step", "Stop Profile", "Cycle Reset", "Time Reset", "Time Reset All", "Time Set", "Tare CTs", "Save Profile", "Open Profile", "Get Profiles", "Update Screen", "Update Controls", "Save App Config", "Write Outputs", "Disable Background", "Enable Background", "Get/Release Control", "Log Fuel Change", "Fuel Change Popup", "Read Inputs", "Remote Timer Reset", "Controller Change", "Get Alarms", "Init Alarms", "Save Alarms", "Voltage Selection", "Set Watlow Temp 1", "Set Watlow Temp 2", "Get Pressure", "Write Tare Pressure", "Adjust Controls", "Reinit ADC", "Write Initial Times", "Write Pumps Present", "HMI Command", "Save Pump Times", "Check Pump Stop Time", "Save LS App Config", "Init Data File", "Reset LS Cycles", "Reset Anomalies", "Reset Opens", "Save LS Data", "Save LS Test Data", "Check Serial Numbers", "Main Tab", "Allow Data Note", "Resume Profile"]
              n215 = Unbundle By Name(w577) -> ("LS App Config.Serial Numbers"=w573:string[])
              n216 = Cluster To Array(cluster="LS Serial Numbers") -> (array=w571:string[])
              n217 = Not Equal?(x=w573, y=w571) -> (x != y?=w570:bool[])
              n218 = Or Array Elements(Boolean array=w570) -> (logical OR=w569:bool)
              n219 = Bundle By Name(cluster=w576, "LS App Config.Serial Numbers"=w571) -> (w575:T25)
            }
            frame 65 {
              w581 = T14[] [enum."Write Outputs"] items=["Main", "Init Files", "Init", "Unused", "Save As", "Start Profile", "Check Step Time", "Alarm", "Alarm Dismiss", "Run Step", "Stop Profile", "Cycle Reset", "Time Reset", "Time Reset All", "Time Set", "Tare CTs", "Save Profile", "Open Profile", "Get Profiles", "Update Screen", "Update Controls", "Save App Config", "Write Outputs", "Disable Background", "Enable Background", "Get/Release Control", "Log Fuel Change", "Fuel Change Popup", "Read Inputs", "Remote Timer Reset", "Controller Change", "Get Alarms", "Init Alarms", "Save Alarms", "Voltage Selection", "Set Watlow Temp 1", "Set Watlow Temp 2", "Get Pressure", "Write Tare Pressure", "Adjust Controls", "Reinit ADC", "Write Initial Times", "Write Pumps Present", "HMI Command", "Save Pump Times", "Check Pump Stop Time", "Save LS App Config", "Init Data File", "Reset LS Cycles", "Reset Anomalies", "Reset Opens", "Save LS Data", "Save LS Test Data", "Check Serial Numbers", "Main Tab", "Allow Data Note", "Resume Profile"]
              n220 = Unbundle By Name(w584) -> ("Bank 1 State:"=w580:u16)
              n221 = Not Equal?(x=w580, y="Bank 1 Power State:") -> (x != y?=w578:bool)
              n222 = Bundle By Name(cluster=w583, "Bank 1 State:"="Bank 1 Power State:") -> (w582:T25)
            }
            frame 66 {
              w588 = T14[] [enum."Write Outputs"] items=["Main", "Init Files", "Init", "Unused", "Save As", "Start Profile", "Check Step Time", "Alarm", "Alarm Dismiss", "Run Step", "Stop Profile", "Cycle Reset", "Time Reset", "Time Reset All", "Time Set", "Tare CTs", "Save Profile", "Open Profile", "Get Profiles", "Update Screen", "Update Controls", "Save App Config", "Write Outputs", "Disable Background", "Enable Background", "Get/Release Control", "Log Fuel Change", "Fuel Change Popup", "Read Inputs", "Remote Timer Reset", "Controller Change", "Get Alarms", "Init Alarms", "Save Alarms", "Voltage Selection", "Set Watlow Temp 1", "Set Watlow Temp 2", "Get Pressure", "Write Tare Pressure", "Adjust Controls", "Reinit ADC", "Write Initial Times", "Write Pumps Present", "HMI Command", "Save Pump Times", "Check Pump Stop Time", "Save LS App Config", "Init Data File", "Reset LS Cycles", "Reset Anomalies", "Reset Opens", "Save LS Data", "Save LS Test Data", "Check Serial Numbers", "Main Tab", "Allow Data Note", "Resume Profile"]
              n223 = Unbundle By Name(w591) -> ("Bank 2 State:"=w587:u16)
              n224 = Not Equal?(x=w587, y="Bank 2 Power State:") -> (x != y?=w586:bool)
              n225 = Bundle By Name(cluster=w590, "Bank 2 State:"="Bank 2 Power State:") -> (w589:T25)
            }
            frame 67 {
              w594 = T14[] [enum."Reset LS Cycles"] items=["Main", "Init Files", "Init", "Unused", "Save As", "Start Profile", "Check Step Time", "Alarm", "Alarm Dismiss", "Run Step", "Stop Profile", "Cycle Reset", "Time Reset", "Time Reset All", "Time Set", "Tare CTs", "Save Profile", "Open Profile", "Get Profiles", "Update Screen", "Update Controls", "Save App Config", "Write Outputs", "Disable Background", "Enable Background", "Get/Release Control", "Log Fuel Change", "Fuel Change Popup", "Read Inputs", "Remote Timer Reset", "Controller Change", "Get Alarms", "Init Alarms", "Save Alarms", "Voltage Selection", "Set Watlow Temp 1", "Set Watlow Temp 2", "Get Pressure", "Write Tare Pressure", "Adjust Controls", "Reinit ADC", "Write Initial Times", "Write Pumps Present", "HMI Command", "Save Pump Times", "Check Pump Stop Time", "Save LS App Config", "Init Data File", "Reset LS Cycles", "Reset Anomalies", "Reset Opens", "Save LS Data", "Save LS Test Data", "Check Serial Numbers", "Main Tab", "Allow Data Note", "Resume Profile"]
            }
            frame 68 {
              w597 = T14[] [enum."Reset Anomalies"] items=["Main", "Init Files", "Init", "Unused", "Save As", "Start Profile", "Check Step Time", "Alarm", "Alarm Dismiss", "Run Step", "Stop Profile", "Cycle Reset", "Time Reset", "Time Reset All", "Time Set", "Tare CTs", "Save Profile", "Open Profile", "Get Profiles", "Update Screen", "Update Controls", "Save App Config", "Write Outputs", "Disable Background", "Enable Background", "Get/Release Control", "Log Fuel Change", "Fuel Change Popup", "Read Inputs", "Remote Timer Reset", "Controller Change", "Get Alarms", "Init Alarms", "Save Alarms", "Voltage Selection", "Set Watlow Temp 1", "Set Watlow Temp 2", "Get Pressure", "Write Tare Pressure", "Adjust Controls", "Reinit ADC", "Write Initial Times", "Write Pumps Present", "HMI Command", "Save Pump Times", "Check Pump Stop Time", "Save LS App Config", "Init Data File", "Reset LS Cycles", "Reset Anomalies", "Reset Opens", "Save LS Data", "Save LS Test Data", "Check Serial Numbers", "Main Tab", "Allow Data Note", "Resume Profile"]
            }
            frame 69 {
              w600 = T14[] [enum."Reset Opens"] items=["Main", "Init Files", "Init", "Unused", "Save As", "Start Profile", "Check Step Time", "Alarm", "Alarm Dismiss", "Run Step", "Stop Profile", "Cycle Reset", "Time Reset", "Time Reset All", "Time Set", "Tare CTs", "Save Profile", "Open Profile", "Get Profiles", "Update Screen", "Update Controls", "Save App Config", "Write Outputs", "Disable Background", "Enable Background", "Get/Release Control", "Log Fuel Change", "Fuel Change Popup", "Read Inputs", "Remote Timer Reset", "Controller Change", "Get Alarms", "Init Alarms", "Save Alarms", "Voltage Selection", "Set Watlow Temp 1", "Set Watlow Temp 2", "Get Pressure", "Write Tare Pressure", "Adjust Controls", "Reinit ADC", "Write Initial Times", "Write Pumps Present", "HMI Command", "Save Pump Times", "Check Pump Stop Time", "Save LS App Config", "Init Data File", "Reset LS Cycles", "Reset Anomalies", "Reset Opens", "Save LS Data", "Save LS Test Data", "Check Serial Numbers", "Main Tab", "Allow Data Note", "Resume Profile"]
            }
            frame 70 {
              w602 = T14[] [enum."Init Data File", enum."Save LS App Config"] items=["Main", "Init Files", "Init", "Unused", "Save As", "Start Profile", "Check Step Time", "Alarm", "Alarm Dismiss", "Run Step", "Stop Profile", "Cycle Reset", "Time Reset", "Time Reset All", "Time Set", "Tare CTs", "Save Profile", "Open Profile", "Get Profiles", "Update Screen", "Update Controls", "Save App Config", "Write Outputs", "Disable Background", "Enable Background", "Get/Release Control", "Log Fuel Change", "Fuel Change Popup", "Read Inputs", "Remote Timer Reset", "Controller Change", "Get Alarms", "Init Alarms", "Save Alarms", "Voltage Selection", "Set Watlow Temp 1", "Set Watlow Temp 2", "Get Pressure", "Write Tare Pressure", "Adjust Controls", "Reinit ADC", "Write Initial Times", "Write Pumps Present", "HMI Command", "Save Pump Times", "Check Pump Stop Time", "Save LS App Config", "Init Data File", "Reset LS Cycles", "Reset Anomalies", "Reset Opens", "Save LS Data", "Save LS Test Data", "Check Serial Numbers", "Main Tab", "Allow Data Note", "Resume Profile"]
              n226 = Unbundle By Name(w605) -> ("day of month"=w604:i32)
              n227 = Get Date/Time In Seconds() -> (seconds since 1Jan1904=w608:timestamp)
              n228 = Seconds To Date/Time(time stamp (now)=w608) -> (date time rec=w609:T45)  [unwired: 1 in]
              n229 = Unbundle By Name(w609) -> ("day of month"=w601:i32)
              n230 = Not Equal?(x=w604, y=w601) -> (x != y?=w603:bool)
              n231 = Bundle By Name(cluster=w607, "day of month"=w601) -> (w606:T25)
            }
            frame 71 {
              w610 = T14[] [enum."Save App Config", enum."Write Outputs"] items=["Main", "Init Files", "Init", "Unused", "Save As", "Start Profile", "Check Step Time", "Alarm", "Alarm Dismiss", "Run Step", "Stop Profile", "Cycle Reset", "Time Reset", "Time Reset All", "Time Set", "Tare CTs", "Save Profile", "Open Profile", "Get Profiles", "Update Screen", "Update Controls", "Save App Config", "Write Outputs", "Disable Background", "Enable Background", "Get/Release Control", "Log Fuel Change", "Fuel Change Popup", "Read Inputs", "Remote Timer Reset", "Controller Change", "Get Alarms", "Init Alarms", "Save Alarms", "Voltage Selection", "Set Watlow Temp 1", "Set Watlow Temp 2", "Get Pressure", "Write Tare Pressure", "Adjust Controls", "Reinit ADC", "Write Initial Times", "Write Pumps Present", "HMI Command", "Save Pump Times", "Check Pump Stop Time", "Save LS App Config", "Init Data File", "Reset LS Cycles", "Reset Anomalies", "Reset Opens", "Save LS Data", "Save LS Test Data", "Check Serial Numbers", "Main Tab", "Allow Data Note", "Resume Profile"]
              n232 = Unbundle By Name(w615) -> ("App Config.Anomaly Threshold:"=w616:dbl)
              n233 = Not Equal?(x=w616, y="Anomaly Threshold:") -> (x != y?=w612:bool)
              n234 = Bundle By Name(cluster=w614, "App Config.Anomaly Threshold:"="Anomaly Threshold:") -> (w613:T25)
            }
            frame 72 {
              w617 = T14[] [enum."Save LS App Config"] items=["Main", "Init Files", "Init", "Unused", "Save As", "Start Profile", "Check Step Time", "Alarm", "Alarm Dismiss", "Run Step", "Stop Profile", "Cycle Reset", "Time Reset", "Time Reset All", "Time Set", "Tare CTs", "Save Profile", "Open Profile", "Get Profiles", "Update Screen", "Update Controls", "Save App Config", "Write Outputs", "Disable Background", "Enable Background", "Get/Release Control", "Log Fuel Change", "Fuel Change Popup", "Read Inputs", "Remote Timer Reset", "Controller Change", "Get Alarms", "Init Alarms", "Save Alarms", "Voltage Selection", "Set Watlow Temp 1", "Set Watlow Temp 2", "Get Pressure", "Write Tare Pressure", "Adjust Controls", "Reinit ADC", "Write Initial Times", "Write Pumps Present", "HMI Command", "Save Pump Times", "Check Pump Stop Time", "Save LS App Config", "Init Data File", "Reset LS Cycles", "Reset Anomalies", "Reset Opens", "Save LS Data", "Save LS Test Data", "Check Serial Numbers", "Main Tab", "Allow Data Note", "Resume Profile"]
              n235 = Unbundle By Name(w622) -> ("LS App Config.Record Constant"=w623:bool)
              n236 = Not Equal?(x=w623, y="Record Constant") -> (x != y?=w619:bool)
              n237 = Bundle By Name(cluster=w621, "LS App Config.Record Constant"="Record Constant") -> (w620:T25)
            }
            frame 73 {
              w626 = T14[] [] items=["Main", "Init Files", "Init", "Unused", "Save As", "Start Profile", "Check Step Time", "Alarm", "Alarm Dismiss", "Run Step", "Stop Profile", "Cycle Reset", "Time Reset", "Time Reset All", "Time Set", "Tare CTs", "Save Profile", "Open Profile", "Get Profiles", "Update Screen", "Update Controls", "Save App Config", "Write Outputs", "Disable Background", "Enable Background", "Get/Release Control", "Log Fuel Change", "Fuel Change Popup", "Read Inputs", "Remote Timer Reset", "Controller Change", "Get Alarms", "Init Alarms", "Save Alarms", "Voltage Selection", "Set Watlow Temp 1", "Set Watlow Temp 2", "Get Pressure", "Write Tare Pressure", "Adjust Controls", "Reinit ADC", "Write Initial Times", "Write Pumps Present", "HMI Command", "Save Pump Times", "Check Pump Stop Time", "Save LS App Config", "Init Data File", "Reset LS Cycles", "Reset Anomalies", "Reset Opens", "Save LS Data", "Save LS Test Data", "Check Serial Numbers", "Main Tab", "Allow Data Note", "Resume Profile"]
              n238 = call "LS Data Global.vi"() -> ("Recording Out"=→"Recording":bool, "Transferring Out"=→"Transferring":bool)  [unwired: 13 in, 1 out]
            }
            frame 74 {
              w629 = T14[] [enum."Save LS App Config", enum."Write Outputs"] items=["Main", "Init Files", "Init", "Unused", "Save As", "Start Profile", "Check Step Time", "Alarm", "Alarm Dismiss", "Run Step", "Stop Profile", "Cycle Reset", "Time Reset", "Time Reset All", "Time Set", "Tare CTs", "Save Profile", "Open Profile", "Get Profiles", "Update Screen", "Update Controls", "Save App Config", "Write Outputs", "Disable Background", "Enable Background", "Get/Release Control", "Log Fuel Change", "Fuel Change Popup", "Read Inputs", "Remote Timer Reset", "Controller Change", "Get Alarms", "Init Alarms", "Save Alarms", "Voltage Selection", "Set Watlow Temp 1", "Set Watlow Temp 2", "Get Pressure", "Write Tare Pressure", "Adjust Controls", "Reinit ADC", "Write Initial Times", "Write Pumps Present", "HMI Command", "Save Pump Times", "Check Pump Stop Time", "Save LS App Config", "Init Data File", "Reset LS Cycles", "Reset Anomalies", "Reset Opens", "Save LS Data", "Save LS Test Data", "Check Serial Numbers", "Main Tab", "Allow Data Note", "Resume Profile"]
              n239 = Unbundle By Name(w633) -> ("LS App Config.2nd Step Check"=w630:bool)
              n240 = Not Equal?(x=w630, y="Second Step Check") -> (x != y?=w632:bool)
              n241 = Bundle By Name(cluster=w635, "LS App Config.2nd Step Check"="Second Step Check") -> (w634:T25)
            }
            frame 75 {
              w639 = T14[] [enum."Save LS App Config", enum."Write Outputs"] items=["Main", "Init Files", "Init", "Unused", "Save As", "Start Profile", "Check Step Time", "Alarm", "Alarm Dismiss", "Run Step", "Stop Profile", "Cycle Reset", "Time Reset", "Time Reset All", "Time Set", "Tare CTs", "Save Profile", "Open Profile", "Get Profiles", "Update Screen", "Update Controls", "Save App Config", "Write Outputs", "Disable Background", "Enable Background", "Get/Release Control", "Log Fuel Change", "Fuel Change Popup", "Read Inputs", "Remote Timer Reset", "Controller Change", "Get Alarms", "Init Alarms", "Save Alarms", "Voltage Selection", "Set Watlow Temp 1", "Set Watlow Temp 2", "Get Pressure", "Write Tare Pressure", "Adjust Controls", "Reinit ADC", "Write Initial Times", "Write Pumps Present", "HMI Command", "Save Pump Times", "Check Pump Stop Time", "Save LS App Config", "Init Data File", "Reset LS Cycles", "Reset Anomalies", "Reset Opens", "Save LS Data", "Save LS Test Data", "Check Serial Numbers", "Main Tab", "Allow Data Note", "Resume Profile"]
              n242 = Unbundle By Name(w641) -> ("LS App Config.Bias Resistances"=w640:dbl[])
              n243 = Not Equal?(x=w640, y="Bias Resistances") -> (x != y?=w637:bool[])
              n244 = Or Array Elements(Boolean array=w637) -> (logical OR=w636:bool)
              n245 = Bundle By Name(cluster=w643, "LS App Config.Bias Resistances"="Bias Resistances") -> (w642:T25)
            }
            frame 76 {
              w646 = T14[] [enum."Save LS App Config", enum."Write Outputs"] items=["Main", "Init Files", "Init", "Unused", "Save As", "Start Profile", "Check Step Time", "Alarm", "Alarm Dismiss", "Run Step", "Stop Profile", "Cycle Reset", "Time Reset", "Time Reset All", "Time Set", "Tare CTs", "Save Profile", "Open Profile", "Get Profiles", "Update Screen", "Update Controls", "Save App Config", "Write Outputs", "Disable Background", "Enable Background", "Get/Release Control", "Log Fuel Change", "Fuel Change Popup", "Read Inputs", "Remote Timer Reset", "Controller Change", "Get Alarms", "Init Alarms", "Save Alarms", "Voltage Selection", "Set Watlow Temp 1", "Set Watlow Temp 2", "Get Pressure", "Write Tare Pressure", "Adjust Controls", "Reinit ADC", "Write Initial Times", "Write Pumps Present", "HMI Command", "Save Pump Times", "Check Pump Stop Time", "Save LS App Config", "Init Data File", "Reset LS Cycles", "Reset Anomalies", "Reset Opens", "Save LS Data", "Save LS Test Data", "Check Serial Numbers", "Main Tab", "Allow Data Note", "Resume Profile"]
              n246 = Unbundle By Name(w648) -> ("LS App Config.Voltage(T)/Resistance(F)"=w647:bool)
              n247 = Not Equal?(x=w647, y="Voltage(T)/Resistance(F)") -> (x != y?=w645:bool)
              n248 = Bundle By Name(cluster=w650, "LS App Config.Voltage(T)/Resistance(F)"="Voltage(T)/Resistance(F)") -> (w649:T25)
            }
            frame 77 {
              w654 = T14[] [enum."Stop Profile"] items=["Main", "Init Files", "Init", "Unused", "Save As", "Start Profile", "Check Step Time", "Alarm", "Alarm Dismiss", "Run Step", "Stop Profile", "Cycle Reset", "Time Reset", "Time Reset All", "Time Set", "Tare CTs", "Save Profile", "Open Profile", "Get Profiles", "Update Screen", "Update Controls", "Save App Config", "Write Outputs", "Disable Background", "Enable Background", "Get/Release Control", "Log Fuel Change", "Fuel Change Popup", "Read Inputs", "Remote Timer Reset", "Controller Change", "Get Alarms", "Init Alarms", "Save Alarms", "Voltage Selection", "Set Watlow Temp 1", "Set Watlow Temp 2", "Get Pressure", "Write Tare Pressure", "Adjust Controls", "Reinit ADC", "Write Initial Times", "Write Pumps Present", "HMI Command", "Save Pump Times", "Check Pump Stop Time", "Save LS App Config", "Init Data File", "Reset LS Cycles", "Reset Anomalies", "Reset Opens", "Save LS Data", "Save LS Test Data", "Check Serial Numbers", "Main Tab", "Allow Data Note", "Resume Profile"]
              w653 = T14[] [enum."Voltage Selection", enum."Resume Profile"] items=["Main", "Init Files", "Init", "Unused", "Save As", "Start Profile", "Check Step Time", "Alarm", "Alarm Dismiss", "Run Step", "Stop Profile", "Cycle Reset", "Time Reset", "Time Reset All", "Time Set", "Tare CTs", "Save Profile", "Open Profile", "Get Profiles", "Update Screen", "Update Controls", "Save App Config", "Write Outputs", "Disable Background", "Enable Background", "Get/Release Control", "Log Fuel Change", "Fuel Change Popup", "Read Inputs", "Remote Timer Reset", "Controller Change", "Get Alarms", "Init Alarms", "Save Alarms", "Voltage Selection", "Set Watlow Temp 1", "Set Watlow Temp 2", "Get Pressure", "Write Tare Pressure", "Adjust Controls", "Reinit ADC", "Write Initial Times", "Write Pumps Present", "HMI Command", "Save Pump Times", "Check Pump Stop Time", "Save LS App Config", "Init Data File", "Reset LS Cycles", "Reset Anomalies", "Reset Opens", "Save LS Data", "Save LS Test Data", "Check Serial Numbers", "Main Tab", "Allow Data Note", "Resume Profile"]
              # "T:Pause\nF:Resume"
              n249 = Unbundle By Name(w657) -> ("Pause Test"=w656:bool)
              n250 = Not Equal?(x=w656, y="pb.Pause/Resume") -> (x != y?=w655:bool)
              n251 = Select(t=w654, s="pb.Pause/Resume", f=w653) -> (s? t:f=w651:T14[])
              n252 = Bundle By Name(cluster=w659, "Pause Test"="pb.Pause/Resume") -> (w658:T25)
            }
          }
        }
        n253 = Tick Count (ms)() -> (millisecond timer value=w84:u32)
        n254 = Subtract(x=w84, y=w86) -> (x-y=w83:u32)
        n255 = Subtract(x=w84, y=w85) -> (x-y=w82:u32)
        n256 = Greater?(x=w83, y=u32 100) -> (0:w78:bool)
        n257 = Greater?(x=w82, y=u32 500) -> (0:w77:bool)
        n258 = disable-structure shown="Disabled" {
          frame Disabled {
          }
          frame Enabled {
          }
        }
        n259 = case shown="True" w77 {
          tunnel: w87 -> [w100 w104]
          tunnel: w76 -> [_ w103]
          tunnel: [w100 w101] -> w88
          frame False {
          }
          frame True {
            n260 = Insert Into Array(array=w104, index=0, new element=w103) -> (w101:T14[])
          }
        }
        n261 = case shown="True" w78 {
          tunnel: w88 -> [w105 w109]
          tunnel: Sequence_States."Read Inputs" -> [_ w108]
          tunnel: [w105 w106] -> w91
          frame False {
          }
          frame True {
            n262 = Insert Into Array(array=w109, index=0, new element=w108) -> (w106:T14[])
          }
        }
        n263 = case shown="True" w79 {
          tunnel: w91 -> [w110 w114]
          tunnel: Sequence_States."Check Step Time" -> [_ w113]
          tunnel: [w110 w111] -> w92
          frame False {
          }
          frame True {
            n264 = Insert Into Array(array=w114, index=0, new element=w113) -> (w111:T14[])
          }
        }
        n265 = case shown="True" w94 {
          tunnel: w92 -> [w115 w119]
          tunnel: w95 -> [_ w118]
          tunnel: [w115 w116] -> w93
          frame False {
          }
          frame True {
            n266 = Insert Into Array(array=w119, index=0, new element=w118) -> (w116:T14[])
          }
        }
      }
      frame "Init Files" {
        w696 = T14[] [enum."Write Tare Pressure", enum."Write Initial Times", enum."Write Pumps Present"] items=["Main", "Init Files", "Init", "Unused", "Save As", "Start Profile", "Check Step Time", "Alarm", "Alarm Dismiss", "Run Step", "Stop Profile", "Cycle Reset", "Time Reset", "Time Reset All", "Time Set", "Tare CTs", "Save Profile", "Open Profile", "Get Profiles", "Update Screen", "Update Controls", "Save App Config", "Write Outputs", "Disable Background", "Enable Background", "Get/Release Control", "Log Fuel Change", "Fuel Change Popup", "Read Inputs", "Remote Timer Reset", "Controller Change", "Get Alarms", "Init Alarms", "Save Alarms", "Voltage Selection", "Set Watlow Temp 1", "Set Watlow Temp 2", "Get Pressure", "Write Tare Pressure", "Adjust Controls", "Reinit ADC", "Write Initial Times", "Write Pumps Present", "HMI Command", "Save Pump Times", "Check Pump Stop Time", "Save LS App Config", "Init Data File", "Reset LS Cycles", "Reset Anomalies", "Reset Opens", "Save LS Data", "Save LS Test Data", "Check Serial Numbers", "Main Tab", "Allow Data Note", "Resume Profile"]
        w705 = dbl[][] [[0.0, 11.0, 0.0, 0.0, 0.0], [0.0, 11.0, 0.0, 0.0, 0.0], [0.0, 11.0, 0.0, 0.0, 0.0], [0.0, 11.0, 0.0, 0.0, 0.0], [0.0, 11.0, 0.0, 0.0, 0.0], [0.0, 11.0, 0.0, 0.0, 0.0], [0.0, 1.0, 0.0, 0.0, 0.0], [0.0, 1.0, 0.0, 0.0, 0.0], [0.0, 1.0, 0.0, 0.0, 0.0], [0.0, 2.0, 0.0, 0.0, 0.0], [0.0, 1.0, 0.0, 0.0, 0.0], [0.0, 1.0, 0.0, 0.0, 0.0], [0.0, 1.0, 0.0, 0.0, 0.0], [0.0, 1.0, 0.0, 0.0, 0.0], [0.0, 1.0, 0.0, 0.0, 0.0], [0.0, 1.0, 0.0, 0.0, 0.0], [0.0, 1.0, 0.0, 0.0, 0.0], [0.0, 1.0, 0.0, 0.0, 0.0], [0.0, 1.0, 0.0, 0.0, 0.0], [0.0, 1.0, 0.0, 0.0, 0.0], [0.0, 1.0, 0.0, 0.0, 0.0], [0.0, 1.0, 0.0, 0.0, 0.0], [-60.0, 24.0, 0.0, 0.0, 0.0], [-60.0, 24.0, 0.0, 0.0, 0.0], [-60.0, 24.0, 0.0, 0.0, 0.0], [-60.0, 24.0, 0.0, 0.0, 0.0], [-60.0, 24.0, 0.0, 0.0, 0.0], [-60.0, 24.0, 0.0, 0.0, 0.0], [-660.0, 200.0, 0.0, 0.0, 0.0], [-660.0, 200.0, 0.0, 0.0, 0.0], [-258.5, 258.5, 0.0, 0.0, 0.0], [-258.5, 258.5, 0.0, 0.0, 0.0], [-258.5, 258.5, 0.0, 0.0, 0.0], [-258.5, 258.5, 0.0, 0.0, 0.0], [-258.5, 258.5, 0.0, 0.0, 0.0], [-258.5, 258.5, 0.0, 0.0, 0.0], [-150.0, 150.0, 0.0, 0.0, 0.0], [-150.0, 150.0, 0.0, 0.0, 0.0], [-150.0, 150.0, 0.0, 0.0, 0.0], [-150.0, 150.0, 0.0, 0.0, 0.0], [-150.0, 150.0, 0.0, 0.0, 0.0], [-150.0, 150.0, 0.0, 0.0, 0.0], [0.0, 1.0, 0.0, 0.0, 0.0], [0.0, 1.0, 0.0, 0.0, 0.0], [0.0, 1.0, 0.0, 0.0, 0.0], [0.0, 1.0, 0.0, 0.0, 0.0], [0.0, 1.0, 0.0, 0.0, 0.0], [0.0, 1.0, 0.0, 0.0, 0.0], [0.0, 11.0, 0.0, 0.0, 0.0], [0.0, 11.0, 0.0, 0.0, 0.0], [0.0, 11.0, 0.0, 0.0, 0.0], [0.0, 11.0, 0.0, 0.0, 0.0], [0.0, 11.0, 0.0, 0.0, 0.0], [0.0, 11.0, 0.0, 0.0, 0.0], [0.0, 0.0001, 0.0, 0.0, 0.0], [0.0, 0.0001, 0.0, 0.0, 0.0], [0.0, 0.0001, 0.0, 0.0, 0.0], [0.0, 0.0001, 0.0, 0.0, 0.0], [0.0, 0.0001, 0.0, 0.0, 0.0], [0.0, 0.0001, 0.0, 0.0, 0.0]]  # Cal Coefficients
        # "This is 10.30.189.0"
        n267 = Unbundle By Name(w714) -> ("App Config"=w699:T6, "LS App Config"=w675:T13)
        n268 = String To IP() -> (0:w709:u32)  [unwired: 1 in]
        n269 = Subtract(x=w709, y=u32 169786624) -> (x-y=w681:u32)
        n270 = Number To Decimal String(number=w681) -> (decimal integer string=w708:string)  [unwired: 1 in]
        n271 = call <vilib>:"Open Config Data.vi"("configuration file path"=path "c:/LS App Config.ini") -> ("error out"=w678:errorcluster, "file created?"=w676:bool, "refnum"=w677:T46)  [unwired: 8 in]
        n272 = case shown="False" w676 {
          tunnel: w678 -> [w732 w739]
          tunnel: w677 -> [w731 w740]
          tunnel: w675 -> [w730 w738]
          tunnel: [w730 w737] -> w664
          tunnel: [w726 w733] -> w674
          frame True {
            n273 = call "Read Write LS App Config.vi"("Write (F)"=TRUE, "Error IN"=w732, "LS App Config In"=w730, "Refnum in"=w731) -> ("Error OUT"=w727:errorcluster, "Refnum out"=w728:T46)  [unwired: 5 in, 1 out]
            n274 = call <vilib>:"Close Config Data.vi"("error in (no error)"=w727, "refnum"=w728) -> ("error out"=w726:errorcluster)  [unwired: 8 in, 1 out]
          }
          frame False {
            n275 = call "Read Write LS App Config.vi"("Error IN"=w739, "LS App Config In"=w738, "Refnum in"=w740) -> ("Error OUT"=w736:errorcluster, "LS App Config Out"=w737:T47, "Refnum out"=w735:T46)  [unwired: 6 in]
            n276 = call <vilib>:"Close Config Data.vi"("error in (no error)"=w736, "refnum"=w735) -> ("error out"=w734:errorcluster)  [unwired: 8 in, 1 out]
            n277 = call <vilib>:"Clear Errors.vi"("error in (no error)"=w734) -> ("error out"=w733:errorcluster)  [unwired: 6 in]
          }
        }
        n278 = call <vilib>:"Open Config Data.vi"("error in (no error)"=w674, "configuration file path"=path "c:/App Config.ini") -> ("error out"=w721:errorcluster, "file created?"=w719:bool, "refnum"=w722:T46)  [unwired: 7 in]
        n279 = case shown="False" w719 {
          tunnel: w722 -> [w771 w776]
          tunnel: w721 -> [w769 w774]
          tunnel: w699 -> [w766 w773]
          tunnel: [w767 w773] -> w682
          tunnel: [w765 w775] -> w683
          frame False {
            # "Read App Config.ini"
            n280 = call "Read Write App Config.vi"("Error IN"=w769, "App Config"=w766, "Refnum in"=w771) -> ("Error OUT"=w768:errorcluster, "App Config OUT"=w767:T6, "Refnum out"=w770:T46)  [unwired: 6 in]
            n281 = call <vilib>:"Close Config Data.vi"("error in (no error)"=w768, "refnum"=w770) -> ("error out"=w772:errorcluster)  [unwired: 8 in, 1 out]
            n282 = call <vilib>:"Clear Errors.vi"("error in (no error)"=w772) -> ("error out"=w765:errorcluster)  [unwired: 6 in]
          }
          frame True {
            # "Doesn't exist, so create."
            n283 = call "Read Write App Config.vi"("Write (F)"=TRUE, "Error IN"=w774, "App Config"=w773, "Refnum in"=w776) -> ("Error OUT"=w778:errorcluster, "Refnum out"=w779:T46)  [unwired: 5 in, 1 out]
            n284 = call <vilib>:"Close Config Data.vi"("error in (no error)"=w778, "refnum"=w779) -> ("error out"=w775:errorcluster)  [unwired: 8 in, 1 out]
          }
        }
        n285 = Concatenate Strings("/c/" ("string"), w708, ".cal" ("string")) -> (w700:string)
        n286 = String To Path(string=w700) -> (path=w701:path)
        n287 = To Long Integer(number=w681) -> (32bit integer=w680:i32)
        n288 = Bundle By Name(cluster=w682, "Data Log Init.IP Last 3"=w680) -> (w668:T6)
        n289 = disable-structure shown="Disabled" {
          disable-tunnel: w668 -> [w723 _]
          frame Disabled {
            n290 = Unbundle By Name(w723) -> ("Data Log Init"=w724:T7)
            n291 = call "Data Logger Main.vi"("Data Logger Mode"=Data_Logger_Mode."Init", "Data Log Init"=w724) -> ()  [unwired: 18 in]
          }
          frame Enabled {
          }
        }
        n292 = Unbundle By Name(w664) -> ("2nd Step Check"=w663:bool)
        n293 = call "Get Elapsed Times.vi"("Error In"=w683, "Path"=path "c:/ElapsedTimes" ("file (use dialog)")) -> ("Error Out"=w703:errorcluster, "Elapsed Times"=w715:dbl[])  [unwired: 8 in]
        n294 = Unbundle By Name(w668) -> ("Voltage Limits"=w686:T41, "Voltage Far PI"=w693:T42, "Voltage Mid PI"=w692:T43, "Voltage Close PI"=w691:T44, "Voltage Scale"=w690:cluster{"V_FFm":dbl, "V_FFb":dbl}, "Voltage Cutoffs"=w689:cluster{"V_MidCutoff":dbl, "V_CloseCutoff":dbl}, "Pressure Scale"=w688:cluster{"Pres_FFm":dbl, "Pres_FFb":dbl}, "Temp Format"=w685:i32, "Temp Tolerance"=w684:dbl)
        n295 = call <vilib>:"Clear Errors.vi"("error in (no error)"=w703) -> ("error out"=w704:errorcluster)  [unwired: 6 in]
        n296 = local write "Second Step Check"(w663) -> ()
        n297 = Unbundle By Name(w668) -> ("Step Threshold:"=w666:dbl, "Anomaly Threshold:"=w665:dbl, "Normal Steps:"=w667:u32)
        n298 = call "Get Pressure Offsets.vi"("Error In"=w704, "Path"=path "c:/PressureOffsets" ("file (use dialog)")) -> ("Error Out"=w702:errorcluster, "Pressure Offsets"=w716:dbl[])  [unwired: 8 in]
        n299 = call <vilib>:"Clear Errors.vi"("error in (no error)"=w702) -> ("error out"=w672:errorcluster)  [unwired: 6 in]
        n300 = local write "Voltage Limits"(w686) -> ()
        n301 = local write "Far PI"(w693) -> ()
        n302 = local write "Mid PI"(w692) -> ()
        n303 = local write "Close PI"(w691) -> ()
        n304 = local write "Voltage Scale"(w690) -> ()
        n305 = local write "Cutoffs"(w689) -> ()
        n306 = local write "Pressure Scale"(w688) -> ()
        n307 = local write "Thermocouple"(w685) -> ()
        n308 = local write "Temp Tolerance"(w684) -> ()
        n309 = call "Get Initial LS Data.vi"("Error In"=w672, "Path"=path "c:/Monitored Statistics") -> ("Error Out"=w671:errorcluster, "Initial LS Data"=w669:T15)  [unwired: 8 in]
        n310 = local write "Step Threshold:"(w666) -> ()
        n311 = local write "Anomaly Threshold:"(w665) -> ()
        n312 = local write "Normal Steps:"(w667) -> ()
        n313 = call <vilib>:"Clear Errors.vi"("error in (no error)"=w671) -> ("error out"=w670:errorcluster)  [unwired: 6 in]
        n314 = call "Get Cal Coefficients.vi"("Error In"=w670, "Path"=w701) -> ("Error"=w711:bool, "Cal Coefficients"=w712:dbl[][])  [unwired: 7 in, 1 out]
        n315 = case shown="False" w711 {
          tunnel: w712 -> [_ w744]
          tunnel: [w741 w743] -> w687
          tunnel: w705 -> [w741 w742]
          frame True {
          }
          frame False {
            n316 = for {
              tunnel: w744 -> [w746] mode=indexing
              shift-right: [w747] -> w743
              shift-left: w742 -> [w748]
              i -> [w745]
              n317 = Index Array(array=w746) -> (element #1=w759:dbl, element #2=w758:dbl, element #3=w757:dbl, element #4=w753:dbl, element #5=w752:dbl)  [unwired: 5 in]
              n318 = Equal To 0?(x=w759) -> (x = 0?=w756:bool)
              n319 = Equal To 0?(x=w758) -> (x = 0?=w755:bool)
              n320 = Equal To 0?(x=w757) -> (x = 0?=w754:bool)
              n321 = Equal To 0?(x=w753) -> (x = 0?=w751:bool)
              n322 = Equal To 0?(x=w752) -> (x = 0?=w750:bool)
              n323 = Compound Arithmetic op=AND(w756, w755, w754, w751, w750) -> (w749:bool)
              n324 = case shown="False" w749 {
                tunnel: w748 -> [w763 w764]
                tunnel: [w762 w764] -> w747
                tunnel: w746 -> [w761 _]
                tunnel: w745 -> [w760 _]
                frame False {
                  n325 = Replace Array Subset(array=w763, new element=w761, index (row)=w760) -> (w762:dbl[][])  [unwired: 1 in]
                }
                frame True {
                }
              }
            }
          }
        }
        n326 = call "PI with FF.vi"("Cutoffs"=w689, "FFcluster"=w690, "ClosePIcluster"=w691, "MidPIcluster"=w692, "FarPIcluster"=w693, "LimitCluster"=w686, "Init (F)"=TRUE) -> ()  [unwired: 8 in, 1 out]
        n327 = call "Handle Profile Resume Info.vi"("Read(F)/Write(T)"=FALSE) -> ("Current Step Out"=w662:i32, "Step Time Left Out"=w661:dbl)  [unwired: 13 in]
        n328 = Insert Into Array(array=w695, index=0, new element=w696) -> (w697:T14[])
        n329 = Bundle By Name(cluster=w714, "App Config"=w668, "Initial Times"=w715, "Pressure Offsets"=w716, "CalArray"=w687, "Initial LS Data"=w669, "LS App Config"=w664, "Current Step"=w662, "Step Time Left"=w661) -> (w713:T25)
        n330 = local write "Step:"(w662) -> ()
        n331 = local write "Time Left:"(w661) -> ()
      }
      frame "Init" {
        w794 = TRUE ("Visible")
        w781 = T30."Enabled" ("Disabled")
        w802 = u16 0 items=["0 - Off", "1 - On", "2 - Pulsing"] ("Bank 1 Power State:")
        w786 = FALSE ("Running?")
        w824 = T14[] [enum."Get Profiles", enum."Enable Background", enum."Get/Release Control", enum."Get Pressure", enum."Get Alarms", enum."Set Watlow Temp 1", enum."Set Watlow Temp 2", enum."Update Controls", enum."Controller Change", enum."Stop Profile"] items=["Main", "Init Files", "Init", "Unused", "Save As", "Start Profile", "Check Step Time", "Alarm", "Alarm Dismiss", "Run Step", "Stop Profile", "Cycle Reset", "Time Reset", "Time Reset All", "Time Set", "Tare CTs", "Save Profile", "Open Profile", "Get Profiles", "Update Screen", "Update Controls", "Save App Config", "Write Outputs", "Disable Background", "Enable Background", "Get/Release Control", "Log Fuel Change", "Fuel Change Popup", "Read Inputs", "Remote Timer Reset", "Controller Change", "Get Alarms", "Init Alarms", "Save Alarms", "Voltage Selection", "Set Watlow Temp 1", "Set Watlow Temp 2", "Get Pressure", "Write Tare Pressure", "Adjust Controls", "Reinit ADC", "Write Initial Times", "Write Pumps Present", "HMI Command", "Save Pump Times", "Check Pump Stop Time", "Save LS App Config", "Init Data File", "Reset LS Cycles", "Reset Anomalies", "Reset Opens", "Save LS Data", "Save LS Test Data", "Check Serial Numbers", "Main Tab", "Allow Data Note", "Resume Profile"]
        # "This solves an issue where location wouldn't\nshow up in the built version."
        n332 = Unbundle By Name(w840) -> ("App Config.Profiles Path"=w830:path, "App Config.Watlow Present"=w832:bool, "App Config.Temp 1"=w839:dbl, "App Config.Temp 2"=w838:dbl, "App Config.Location"=w831:string, "LS App Config.Record Bursts"=w799:bool, "LS App Config.RecInterval(s)"=w820:i32, "LS App Config.RecDuration(s)"=w819:i32, "LS App Config.RecFrequeny (Hz)"=w818:i32, "App Config.CA Number"=w800:string, "LS App Config.Data File Name:"=w780:string, "LS App Config.Serial Numbers"=w784:string[], "LS App Config.DetectionMode"=w787:i32)
        "Location:" <- w831
        n333 = case shown="1" w787 {
          frame 0, Default {
            n334 = local write "Live Data Tab"(enum32{"Page 1", "Page 2", "Page 3"}."Page 2" ("Live Data Tab")) -> ()
          }
          frame 1 {
            n335 = local write "Live Data Tab"(enum32{"Page 1", "Page 2", "Page 3"}."Page 3" ("Live Data Tab")) -> ()
          }
        }
        n336 = call "Init FPGA.vi"("FPGA Ref"=w796) -> ("error out"=w836:errorcluster, "FPGA Ref Out"=w837:T26)  [unwired: 9 in]
        n337 = call "Watlow Global.vi"("Write (F)"=TRUE, "Watlow Present"=w832) -> ()  [unwired: 9 in, 1 out]
        n338 = disable-structure shown="Enabled" {
          disable-tunnel: w837 -> [w871 _]
          disable-tunnel: w836 -> [w870 w872]
          disable-tunnel: [w869 w872] -> w835
          frame Disabled {
            n339 = call "Init ADCs.vi"("Error IN"=w870, "FPGA Ref"=w871) -> ("error out"=w869:errorcluster)  [unwired: 7 in, 2 out]
          }
          frame Enabled {
          }
        }
        n340 = local write "Main Tab"(T9."Main" ("Main Tab")) -> ()
        n341 = local write "pb.Run Profile"(FALSE ("pb.Run Profile")) -> ()
        n342 = local write "Bank 1 Power State:"(w802) -> ()
        n343 = local write "Bank 2 Power State:"(w802) -> ()
        n344 = property on="Location:" class="Str"("Text.Text"=w831) -> ()  [unwired: 2 in, 2 out]
        n345 = local write "Tank 1 Temp Cmd:"(w839) -> ()
        n346 = local write "Tank 2 Temp Cmd:"(w838) -> ()
        n347 = flat-sequence {
          tunnel: w835 -> [_]
          tunnel: w834 -> [w873]
          frame #0 {
            n348 = Set Occurrence(w873) -> ()
          }
        }
        n349 = Empty String/Path?(string/path=w800) -> (empty?=w788:bool)
        n350 = Empty String/Path?(string/path=w780) -> (empty?=w801:bool)
        n351 = call <vilib>:"Check if File or Folder Exists.vi"("path"=path "u:/CA Numbers" ("base path")) -> ("error out"=w815:errorcluster, "file or folder exists?"=w817:bool, "dup path"=w816:path)  [unwired: 8 in]
        n352 = Or(x=w788, y=w801) -> (x .or. y?=w793:bool)
        n353 = case shown="False" w817 {
          tunnel: w816 -> [w866 w868]
          tunnel: w815 -> [w865 w867]
          tunnel: [w864 w868] -> w813
          tunnel: [w863 w867] -> w808
          frame False {
            n354 = Create Folder(path (use dialog)=w866, error in=w865) -> (created path=w864:path, error out=w863:errorcluster)  [unwired: 1 in, 1 out]
          }
          frame True {
          }
        }
        n355 = call <vilib>:"Check if File or Folder Exists.vi"("path"=w830) -> ("file or folder exists?"=w844:bool, "dup path"=w843:path)  [unwired: 8 in, 1 out]
        n356 = Build Path(base path=w813, name or relative path=w800) -> (appended path=w810:path)
        n357 = case shown="False" w844 {
          tunnel: w843 -> [w874 _]
          frame False {
            n358 = Create Folder(path (use dialog)=w874) -> ()  [unwired: 2 in, 3 out]
          }
          frame True {
          }
        }
        n359 = call <vilib>:"Check if File or Folder Exists.vi"("error in (no error)"=w808, "path"=w810) -> ("error out"=w812:errorcluster, "file or folder exists?"=w789:bool, "dup path"=w811:path)  [unwired: 7 in]
        n360 = Or(x=w789, y=w788) -> (x .or. y?=w790:bool)
        n361 = case shown="False" w793 {
          tunnel: w799 -> [w848 _]
          tunnel: [w848 FALSE ("Record")] -> w795
          tunnel: [T30."Enabled" ("Disabled") T30."Disabled and Grayed Out" ("Disabled")] -> w798
          frame False {
            # "Valid File"
          }
          frame True {
            # "Invalid File"
          }
        }
        n362 = local write "pb.Pause/Resume"(TRUE) -> ()
        n363 = case shown="False" w790 {
          tunnel: w811 -> [w860 w862]
          tunnel: w812 -> [w859 w861]
          tunnel: [w858 w862] -> w809
          tunnel: [w857 w861] -> w804
          frame False {
            n364 = Create Folder(path (use dialog)=w860, error in=w859) -> (created path=w858:path, error out=w857:errorcluster)  [unwired: 1 in, 1 out]
          }
          frame True {
          }
        }
        n365 = Build Path(base path=w809, name or relative path=w780) -> (appended path=w805:path)
        n366 = property on="Data File Name:" class="Str"("Visible"=w794, "DisabledEnum"=w781) -> ()  [unwired: 2 in, 2 out]
        n367 = property on="pb.Pause/Resume" class="Bool (strict)"("DisabledEnum"=w781) -> ()  [unwired: 2 in, 2 out]
        n368 = call <vilib>:"Check if File or Folder Exists.vi"("error in (no error)"=w804, "path"=w805) -> ("error out"=w806:errorcluster, "file or folder exists?"=w792:bool, "dup path"=w807:path)  [unwired: 7 in]
        n369 = Or(x=w792, y=w793) -> (x .or. y?=w791:bool)
        n370 = case shown="False" w791 {
          tunnel: w807 -> [w854 w856]
          tunnel: w806 -> [w853 w855]
          tunnel: [w851 w856] -> w797
          tunnel: [w852 w855] -> w803
          frame False {
            n371 = Create Folder(path (use dialog)=w854, error in=w853) -> (created path=w851:path, error out=w852:errorcluster)  [unwired: 1 in, 1 out]
          }
          frame True {
          }
        }
        n372 = property on="Record During Profile" class="Bool (strict)"("Value"=w795, "DisabledEnum"=w798) -> ()  [unwired: 2 in, 2 out]
        n373 = property on="pb.Run Profile" class="Bool (strict)"("Visible"=w794, "DisabledEnum"=w781) -> ()  [unwired: 2 in, 2 out]
        n374 = Bundle(cluster=T29 {"Running?"=FALSE, "Profile Record"=FALSE, "RecordInterval"=0, "RecordDuration"=0, "RecordFreq"=0, "Data Filepath"=path "", "Hr Record"=FALSE, "Serial Numbers"=[]} ("LS Cluster In"), "Running?"=w786, "Profile Record"=w795, "RecordInterval"=w820, "RecordDuration"=w819, "RecordFreq"=w818, "Data Filepath"=w797, "Hr Record"=w786, "Serial Numbers"=w784) -> (w821:T29)
        n375 = call "Controller List.vi"() -> ("Controller List OUT"=w829:T22[])  [unwired: 11 in]
        n376 = call "LS Data Global.vi"("Mode"=enum16{"Read", "Engine Writes", "Main Writes"}."Main Writes", "LS Cluster In"=w821) -> ()  [unwired: 11 in, 3 out]
        n377 = Bundle By Name(cluster=w840, "Alarm Config Path"=path "c:/Alarm Config", "Fuel Log Path"=path "u:/Fuel Change Log.csv", "Tank CMDs.Temp 1 CMD"=w839, "Tank CMDs.Temp 2 CMD"=w838, "Controller List"=w829, "LS Data Filepath"=w797, "pb.Run Profile"=w786, "LS App Config.Record Bursts"=w795) -> (w841:T25)
        n378 = call <vilib>:"Clear Errors.vi"("error in (no error)"=w803) -> ()  [unwired: 6 in, 1 out]
        n379 = Insert Into Array(array=w825, index=0, new element=w824) -> (w822:T14[])
      }
      frame "Unused" {
      }
      frame "Get Alarms" {
        n380 = Unbundle By Name(w884) -> ("Alarm Config"=w885:T10, "Alarm Config Path"=w882:path)
        n381 = call <vilib>:"Check if File or Folder Exists.vi"("path"=w882) -> ("file or folder exists?"=w887:bool, "dup path"=w886:path)  [unwired: 8 in, 1 out]
        n382 = case shown="False" w887 {
          tunnel: w886 -> [w892 w899]
          tunnel: w885 -> [_ w897]
          tunnel: [T10 {"Alarms:"=[{"Description:"="PS/E-Stop/Float Switch", "Enabled:"=TRUE, "Data Index:"=9, "Data Type:"="Tank", "Low Limit:"=5.0, "High Limit:"=20.0, "Trip Time:"=1000, "Profile Sync:"=FALSE}, {"Description:"="Voltage (pump or ctrl)", "Enabled:"=TRUE, "Data Index:"=0, "Data Type:"="Pump", "Low Limit:"=12.0, "High Limit:"=17.0, "Trip Time:"=3000, "Profile Sync:"=TRUE}, {"Description:"="Pump Current", "Enabled:"=TRUE, "Data Index:"=10, "Data Type:"="Pump", "Low Limit:"=0.0, "High Limit:"=22.0, "Trip Time:"=1000, "Profile Sync:"=TRUE}, {"Description:"="Pump Speed", "Enabled:"=TRUE, "Data Index:"=16, "Data Type:"="Pump", "Low Limit:"=0.0, "High Limit:"=10000.0, "Trip Time:"=1000, "Profile Sync:"=TRUE}, {"Description:"="Controller Current", "Enabled:"=TRUE, "Data Index:"=22, "Data Type:"="Pump", "Low Limit:"=0.0, "High Limit:"=20.0, "Trip Time:"=1000, "Profile Sync:"=TRUE}, {"Description:"="Pump Pressure", "Enabled:"=TRUE, "Data Index:"=30, "Data Type:"="Pump", "Low Limit:"=550.0, "High Limit:"=750.0, "Trip Time:"=1000, "Profile Sync:"=TRUE}, {"Description:"="Pump Flow", "Enabled:"=FALSE, "Data Index:"=36, "Data Type:"="Pump", "Low Limit:"=0.0, "High Limit:"=400.0, "Trip Time:"=1000, "Profile Sync:"=TRUE}, {"Description:"="Tank Temperature 1", "Enabled:"=FALSE, "Data Index:"=28, "Data Type:"="Tank", "Low Limit:"=-50.0, "High Limit:"=0.0, "Trip Time:"=10000, "Profile Sync:"=FALSE}, {"Description:"="Tank Temperature 2", "Enabled:"=FALSE, "Data Index:"=29, "Data Type:"="Tank", "Low Limit:"=0.0, "High Limit:"=70.0, "Trip Time:"=10000, "Profile Sync:"=FALSE}], "Profile Sync:"={"Trip Time:"=2000, "Consecutive Trips:"=5}} ("Alarm Config") w895] -> w878
          tunnel: [w889 w894] -> w877
          frame False {
            w889 = T14[] [enum."Init Alarms", enum."Save Alarms"] items=["Main", "Init Files", "Init", "Unused", "Save As", "Start Profile", "Check Step Time", "Alarm", "Alarm Dismiss", "Run Step", "Stop Profile", "Cycle Reset", "Time Reset", "Time Reset All", "Time Set", "Tare CTs", "Save Profile", "Open Profile", "Get Profiles", "Update Screen", "Update Controls", "Save App Config", "Write Outputs", "Disable Background", "Enable Background", "Get/Release Control", "Log Fuel Change", "Fuel Change Popup", "Read Inputs", "Remote Timer Reset", "Controller Change", "Get Alarms", "Init Alarms", "Save Alarms", "Voltage Selection", "Set Watlow Temp 1", "Set Watlow Temp 2", "Get Pressure", "Write Tare Pressure", "Adjust Controls", "Reinit ADC", "Write Initial Times", "Write Pumps Present", "HMI Command", "Save Pump Times", "Check Pump Stop Time", "Save LS App Config", "Init Data File", "Reset LS Cycles", "Reset Anomalies", "Reset Opens", "Save LS Data", "Save LS Test Data", "Check Serial Numbers", "Main Tab", "Allow Data Note", "Resume Profile"]
            n383 = Open/Create/Replace File(file path (use dialog)=w892, operation (0:open)=T31."create") -> (refnum out=w891:refnum<file>, error out=w890:errorcluster)  [unwired: 4 in, 1 out]
            n384 = Close File(refnum=w891, error in=w890) -> ()  [unwired: 2 out]
          }
          frame True {
            w894 = T14[] [enum."Init Alarms"] items=["Main", "Init Files", "Init", "Unused", "Save As", "Start Profile", "Check Step Time", "Alarm", "Alarm Dismiss", "Run Step", "Stop Profile", "Cycle Reset", "Time Reset", "Time Reset All", "Time Set", "Tare CTs", "Save Profile", "Open Profile", "Get Profiles", "Update Screen", "Update Controls", "Save App Config", "Write Outputs", "Disable Background", "Enable Background", "Get/Release Control", "Log Fuel Change", "Fuel Change Popup", "Read Inputs", "Remote Timer Reset", "Controller Change", "Get Alarms", "Init Alarms", "Save Alarms", "Voltage Selection", "Set Watlow Temp 1", "Set Watlow Temp 2", "Get Pressure", "Write Tare Pressure", "Adjust Controls", "Reinit ADC", "Write Initial Times", "Write Pumps Present", "HMI Command", "Save Pump Times", "Check Pump Stop Time", "Save LS App Config", "Init Data File", "Reset LS Cycles", "Reset Anomalies", "Reset Opens", "Save LS Data", "Save LS Test Data", "Check Serial Numbers", "Main Tab", "Allow Data Note", "Resume Profile"]
            n385 = Read from Text File(file (use dialog)=w899) -> (refnum out=w896:refnum<file>, text=w898:string)  [unwired: 3 in, 2 out]
            n386 = Close File(refnum=w896) -> ()  [unwired: 1 in, 2 out]
            n387 = Unflatten From JSON(JSON string=w898, type and defaults=w897) -> (value=w895:T10)  [unwired: 5 in, 1 out]
          }
        }
        n388 = Bundle By Name(cluster=w884, "Alarm Config"=w878) -> (w883:T25)
        n389 = local write "Alarm Config"(w878) -> ()
        n390 = Insert Into Array(array=w879, index=0, new element=w877) -> (w880:T14[])
      }
      frame "Init Alarms" {
        # "Initialize alarm arrays."
        n391 = Unbundle By Name(w906) -> ("Alarm Config.Alarms:"=w908:T11[])
        n392 = for {
          tunnel: w908 -> [w915] mode=indexing
          shift-right: [w911] -> w902
          shift-left: 0 -> [w910]
          n393 = Unbundle By Name(w915) -> ("Data Type:"=w914:string, "Enabled:"=w913:bool)
          n394 = case shown="\"Pump\", Default" w914 {
            tunnel: [6 1] -> w912
            frame "Pump", Default {
            }
            frame "Tank" {
            }
          }
          n395 = case shown="True" w913 {
            tunnel: w912 -> [_ w919]
            tunnel: [w916 w918] -> w911
            tunnel: w910 -> [w916 w917]
            frame False {
            }
            frame True {
              n396 = Add(x=w919, y=w917) -> (x+y=w918:i32)
            }
          }
        }
        n397 = Tick Count (ms)() -> (millisecond timer value=w903:u32)
        n398 = Initialize Array(0, w902) -> (w901:i32[])
        n399 = Initialize Array(w903, w902) -> (w900:u32[])
        n400 = Bundle By Name(cluster=w906, "Trip Counters"=w901, "Previous Times"=w900, "Prev ON Times"=w900) -> (w905:T25)
      }
      frame "Save Alarms" {
        n401 = Unbundle By Name(w925) -> ("Alarm Config Path"=w923:path, "Alarm Config"=w924:T10)
        n402 = Flatten To JSON(anything=w924) -> (JSON string=w922:string)  [unwired: 2 in, 1 out]
        n403 = Write to Text File(file (use dialog)=w923, text=w922) -> ()  [unwired: 2 in, 3 out]
      }
      frame "Get Profiles" {
        n404 = Unbundle By Name(w934) -> ("App Config.Profiles Path"=w935:path)
        n405 = List Folder(path=w935) -> (filenames=w932:string[], error out=w931:errorcluster)  [unwired: 3 in, 2 out]
        n406 = call <vilib>:"Clear Errors.vi"("error in (no error)"=w931) -> ()  [unwired: 6 in, 1 out]
        n407 = property on="Profile Name:" class="CmbBox"("Strings[]"=w932) -> ()  [unwired: 2 in, 2 out]
        n408 = Bundle By Name(cluster=w934, "Profiles"=w932) -> (w933:T25)
        n409 = Insert Into Array(array=w928, index=0, new element=Sequence_States."Open Profile") -> (w927:T14[])
      }
      frame "Open Profile" {
        w937 = T14[] [enum."Update Screen", enum."Save App Config"] items=["Main", "Init Files", "Init", "Unused", "Save As", "Start Profile", "Check Step Time", "Alarm", "Alarm Dismiss", "Run Step", "Stop Profile", "Cycle Reset", "Time Reset", "Time Reset All", "Time Set", "Tare CTs", "Save Profile", "Open Profile", "Get Profiles", "Update Screen", "Update Controls", "Save App Config", "Write Outputs", "Disable Background", "Enable Background", "Get/Release Control", "Log Fuel Change", "Fuel Change Popup", "Read Inputs", "Remote Timer Reset", "Controller Change", "Get Alarms", "Init Alarms", "Save Alarms", "Voltage Selection", "Set Watlow Temp 1", "Set Watlow Temp 2", "Get Pressure", "Write Tare Pressure", "Adjust Controls", "Reinit ADC", "Write Initial Times", "Write Pumps Present", "HMI Command", "Save Pump Times", "Check Pump Stop Time", "Save LS App Config", "Init Data File", "Reset LS Cycles", "Reset Anomalies", "Reset Opens", "Save LS Data", "Save LS Test Data", "Check Serial Numbers", "Main Tab", "Allow Data Note", "Resume Profile"]
        n410 = Unbundle By Name(w949) -> ("App Config.Profiles Path"=w951:path, "App Config.Current Profile"=w950:string)
        n411 = Build Path(base path=w951, name or relative path=w950) -> (appended path=w946:path)
        n412 = Read from Text File(file (use dialog)=w946) -> (refnum out=w944:refnum<file>, text=w945:string, error out=w943:errorcluster)  [unwired: 3 in, 1 out]
        n413 = Close File(refnum=w944, error in=w943) -> (error out=w942:errorcluster)  [unwired: 1 out]
        n414 = case shown="No Error" w942 {
          tunnel: w945 -> [w953 _]
          tunnel: [w954 string[][] []] -> w936
          frame No Error {
            n415 = Spreadsheet String To Array(delimiter (Tab)=",", format string="%s", spreadsheet string=w953, array type (2D Dbl)=string[][] []) -> (array=w954:string[][])
          }
          frame Error {
          }
        }
        n416 = Array Size(array=w936) -> (size(s)=w947:i32[])
        n417 = Index Array(array=w947) -> (element=w941:i32)  [unwired: 1 in]
        n418 = Bundle By Name(cluster=w949, "Profile"=w936, "# of Steps"=w941) -> (w948:T25)
        n419 = Insert Into Array(array=w939, index=0, new element=w937) -> (w938:T14[])
      }
      frame "Save Profile" {
        n420 = Unbundle By Name(w963) -> ("App Config.Profiles Path"=w967:path, "App Config.Current Profile"=w965:string, "Profile"=w966:string[][])
        n421 = Empty String/Path?(string/path=w965) -> (empty?=w964:bool)
        n422 = case shown="False" w964 {
          tunnel: w967 -> [w971 _]
          tunnel: w965 -> [w970 _]
          tunnel: w966 -> [w969 _]
          tunnel: [w968 string[][] [] ("Profile OUT")] -> w960
          frame False {
            n423 = call "Save Profile.vi"("Profile"=w969, "Current Profile"=w970, "Profiles Path"=w971) -> ("Profile OUT"=w968:string[][])  [unwired: 8 in]
          }
          frame True {
          }
        }
        n424 = Array Size(array=w960) -> (size(s)=w961:i32[])
        n425 = Index Array(array=w961) -> (element=w959:i32)  [unwired: 1 in]
        n426 = Bundle By Name(cluster=w963, "Profile"=w960, "# of Steps"=w959) -> (w962:T25)
      }
      frame "Start Profile" {
        w975 = TRUE ("Running?")
        w989 = T14[] [enum."Init Alarms", enum."Check Step Time"] items=["Main", "Init Files", "Init", "Unused", "Save As", "Start Profile", "Check Step Time", "Alarm", "Alarm Dismiss", "Run Step", "Stop Profile", "Cycle Reset", "Time Reset", "Time Reset All", "Time Set", "Tare CTs", "Save Profile", "Open Profile", "Get Profiles", "Update Screen", "Update Controls", "Save App Config", "Write Outputs", "Disable Background", "Enable Background", "Get/Release Control", "Log Fuel Change", "Fuel Change Popup", "Read Inputs", "Remote Timer Reset", "Controller Change", "Get Alarms", "Init Alarms", "Save Alarms", "Voltage Selection", "Set Watlow Temp 1", "Set Watlow Temp 2", "Get Pressure", "Write Tare Pressure", "Adjust Controls", "Reinit ADC", "Write Initial Times", "Write Pumps Present", "HMI Command", "Save Pump Times", "Check Pump Stop Time", "Save LS App Config", "Init Data File", "Reset LS Cycles", "Reset Anomalies", "Reset Opens", "Save LS Data", "Save LS Test Data", "Check Serial Numbers", "Main Tab", "Allow Data Note", "Resume Profile"]
        w992 = 0 ("Current Step")
        w986 = T30."Disabled" ("Disabled")
        n427 = Unbundle By Name(w976) -> ("LS App Config.Record Bursts"=w984:bool, "LS App Config.RecInterval(s)"=w983:i32, "LS App Config.RecDuration(s)"=w982:i32, "LS App Config.RecFrequeny (Hz)"=w981:i32, "LS Data Filepath"=w980:path, "LS App Config.Record Constant"=w978:bool, "LS App Config.Serial Numbers"=w977:string[])
        n428 = Bundle(cluster=T29 {"Running?"=FALSE, "Profile Record"=FALSE, "RecordInterval"=0, "RecordDuration"=0, "RecordFreq"=0, "Data Filepath"=path "", "Hr Record"=FALSE, "Serial Numbers"=[]} ("LS Cluster In"), "Running?"=w975, "Profile Record"=w984, "RecordInterval"=w983, "RecordDuration"=w982, "RecordFreq"=w981, "Data Filepath"=w980, "Hr Record"=w978, "Serial Numbers"=w977) -> (w985:T29)
        n429 = disable-structure shown="Enabled" {
          disable-tunnel: "Data Log Enabled" -> [w999 _]
          disable-tunnel: w976 -> [w998 _]
          frame Disabled {
            n430 = case shown="True" w999 {
              tunnel: w998 -> [_ w1006]
              frame False {
              }
              frame True {
                n431 = Unbundle By Name(w1006) -> ("App Config"=w1005:T6, "Profile"=w1004:string[][], "App Config.Controller Type:"=w1003:T3, "Tank CMDs"=w1001:T19)
                n432 = Format Into String(w1003) -> (resulting string=w1002:string)  [unwired: 3 in, 1 out]
                n433 = Bundle By Name(cluster=T32 {"App Config"={"Location"="", "Profiles Path"=path "", "Current Profile"="", "CA Number"="", "Cycles Completed"=0, "Controller Type:"=enum."Kuhnke", "Stagger Time (ms)"=0, "Tank 1 Fuel"="", "Tank 2 Fuel"="", "Serial Numbers"={"Position 1 SN"="", "Position 2 SN"="", "Poaition 3 SN"="", "Position 4 SN"="", "Position 5 SN"="", "Position 6 SN"=""}, "Pumps Present"={"Pump 1"=FALSE, "Pump 2"=FALSE, "Pump 3"=FALSE, "Pump 4"=FALSE, "Pump 5"=FALSE, "Pump 6"=FALSE}, "VoltCtrlRef"="", "VoltageSelect"=FALSE, "Watlow Present"=FALSE, "Temp 1"=0.0, "Temp 2"=0.0, "V_Run PI?"=FALSE, "Voltage Limits"={"V_Step"=0.0, "V_CmdMax"=0.0, "V_CmdMin"=0.0}, "Voltage Far PI"={"V_FarSlew"=0.0, "V_FarKp"=0.0, "V_FarKi"=0.0}, "Voltage Mid PI"={"V_MidSlew"=0.0, "V_MidKp"=0.0, "V_MidKi"=0.0}, "Voltage Close PI"={"V_CloseSlew"=0.0, "V_CloseKp"=0.0, "V_CloseKi"=0.0}, "Voltage Scale"={"V_FFm"=0.0, "V_FFb"=0.0}, "Voltage Cutoffs"={"V_MidCutoff"=0.0, "V_CloseCutoff"=0.0}, "Pressure Scale"={"Pres_FFm"=0.0, "Pres_FFb"=0.0}, "Temp Format"=0, "Temp Tolerance"=0.0, "Target Voltage"=0.0, "Target Pressure"=0.0, "Data Log Init"={"Data Path"=path "", "Data Log Rate (S/s)"=0, "AKLH Rate (Hours/S)"=0.0, "Sync Time Offset (min)"=0, "IP Last 3"=0, "WebDAV IP"=""}, "Email Handler IP"="", "ADC Check"=FALSE, "3 Pump Tank"=FALSE, "Cycle Threshold:"=0.0, "Cycle Pts to Avg:"=0, "Anomaly Threshold:"=0.0, "Normal Steps:"=0, "Step Threshold:"=0.0}, "Profile"=[], "Controller Type"="", "Tank CMDs"={"PS CMD"=0.0, "Press CMD"=0.0, "Temp 1 CMD"=0.0, "Temp 2 CMD"=0.0}} ("Data Log Start"), "App Config"=w1005, "Profile"=w1004, "Controller Type"=w1002, "Tank CMDs"=w1001) -> (w1007:T32)
                n434 = call "Data Logger Main.vi"("Data Logger Mode"=Data_Logger_Mode."Start", "Data Log Start"=w1007) -> ()  [unwired: 18 in]
              }
            }
          }
          frame Enabled {
          }
        }
        n435 = call "LS Data Global.vi"("Mode"=enum16{"Read", "Engine Writes", "Main Writes"}."Main Writes", "LS Cluster In"=w985) -> ()  [unwired: 11 in, 3 out]
        n436 = local write "pb.Pause/Resume"(FALSE) -> ()
        n437 = property on="Bank 1" class="Clust (strict)"("DisabledEnum"=w986) -> ()  [unwired: 2 in, 2 out]
        n438 = property on="Bank 2" class="Clust (strict)"("DisabledEnum"=w986) -> ()  [unwired: 2 in, 2 out]
        n439 = property on="Live Data Tab" class="TabCtl (strict)"("DisabledEnum"=w986) -> ()  [unwired: 2 in, 2 out]
        n440 = property on="Pump Timers Tab" class="TabCtl (strict)"("DisabledEnum"=w986) -> ()  [unwired: 2 in, 2 out]
        n441 = Get Date/Time In Seconds() -> (seconds since 1Jan1904=w995:timestamp)
        n442 = To Double Precision Float(number=w995) -> (double precision float=w994:dbl)
        n443 = Bundle By Name(cluster=w976, "Recording"="Data Log Enabled", "Run Profile"=TRUE, "Step Start Time"=w994, "Last Profile Time"=w994, "Step Time"=0.0, "Current Step"=w992, "Stagger Counter"=w992, "pb.Run Profile"=w975) -> (w997:T25)
        n444 = Insert Into Array(array=w991, index=0, new element=w989) -> (w990:T14[])
      }
      frame "Resume Profile" {
        w1028 = TRUE ("Running?")
        w1041 = T14[] [enum."Init Alarms", enum."Run Step", enum."Check Step Time"] items=["Main", "Init Files", "Init", "Unused", "Save As", "Start Profile", "Check Step Time", "Alarm", "Alarm Dismiss", "Run Step", "Stop Profile", "Cycle Reset", "Time Reset", "Time Reset All", "Time Set", "Tare CTs", "Save Profile", "Open Profile", "Get Profiles", "Update Screen", "Update Controls", "Save App Config", "Write Outputs", "Disable Background", "Enable Background", "Get/Release Control", "Log Fuel Change", "Fuel Change Popup", "Read Inputs", "Remote Timer Reset", "Controller Change", "Get Alarms", "Init Alarms", "Save Alarms", "Voltage Selection", "Set Watlow Temp 1", "Set Watlow Temp 2", "Get Pressure", "Write Tare Pressure", "Adjust Controls", "Reinit ADC", "Write Initial Times", "Write Pumps Present", "HMI Command", "Save Pump Times", "Check Pump Stop Time", "Save LS App Config", "Init Data File", "Reset LS Cycles", "Reset Anomalies", "Reset Opens", "Save LS Data", "Save LS Test Data", "Check Serial Numbers", "Main Tab", "Allow Data Note", "Resume Profile"]
        w1039 = T30."Disabled" ("Disabled")
        # "New Step should be False so this is the only way to get Step Start Time set correctly"
        # "Time this step has ran"
        # "Removed writing the Current Step as it is already correct"
        # "Added Run Step"
        n445 = Unbundle By Name(w1029) -> ("Profile"=w1016:string[][], "Current Step"=w1017:i32, "Step Time Left"=w1012:dbl, "LS App Config.Record Bursts"=w1037:bool, "LS App Config.RecInterval(s)"=w1036:i32, "LS App Config.RecDuration(s)"=w1035:i32, "LS App Config.RecFrequeny (Hz)"=w1034:i32, "LS Data Filepath"=w1033:path, "LS App Config.Record Constant"=w1031:bool, "LS App Config.Serial Numbers"=w1030:string[])
        n446 = local read "Data Log Enabled"() -> (w1025:bool)
        n447 = Bundle(cluster=T29 {"Running?"=FALSE, "Profile Record"=FALSE, "RecordInterval"=0, "RecordDuration"=0, "RecordFreq"=0, "Data Filepath"=path "", "Hr Record"=FALSE, "Serial Numbers"=[]} ("LS Cluster In"), "Running?"=w1028, "Profile Record"=w1037, "RecordInterval"=w1036, "RecordDuration"=w1035, "RecordFreq"=w1034, "Data Filepath"=w1033, "Hr Record"=w1031, "Serial Numbers"=w1030) -> (w1038:T29)
        n448 = Decrement(x=w1017) -> (x-1=w1018:i32)
        n449 = Index Array(array=w1016, index (row)=w1018) -> (element=w1015:string[])  [unwired: 1 in]
        n450 = call "LS Data Global.vi"("Mode"=enum16{"Read", "Engine Writes", "Main Writes"}."Main Writes", "LS Cluster In"=w1038) -> ()  [unwired: 11 in, 3 out]
        n451 = Delete From Array(array=w1015, length=1, index=0 ("length")) -> (array with subset deleted=w1021:string[])  [unwired: 1 out]
        n452 = Fract/Exp String To Number(string=w1021) -> (number=w1014:dbl[])  [unwired: 3 in, 1 out]
        n453 = Delete From Array(array=w1014, length=1, index=0 ("length")) -> (deleted portion=w1024:dbl[])  [unwired: 1 out]
        n454 = Index Array(array=w1024) -> (element=w1013:dbl)  [unwired: 1 in]
        n455 = Subtract(x=w1013, y=w1012) -> (x-y=w1011:dbl)
        n456 = local write "pb.Pause/Resume"(FALSE) -> ()
        n457 = property on="Bank 1" class="Clust (strict)"("DisabledEnum"=w1039) -> ()  [unwired: 2 in, 2 out]
        n458 = property on="Bank 2" class="Clust (strict)"("DisabledEnum"=w1039) -> ()  [unwired: 2 in, 2 out]
        n459 = property on="Live Data Tab" class="TabCtl (strict)"("DisabledEnum"=w1039) -> ()  [unwired: 2 in, 2 out]
        n460 = property on="Pump Timers Tab" class="TabCtl (strict)"("DisabledEnum"=w1039) -> ()  [unwired: 2 in, 2 out]
        n461 = Get Date/Time In Seconds() -> (seconds since 1Jan1904=w1045:timestamp)
        n462 = To Double Precision Float(number=w1045) -> (double precision float=w1009:dbl)
        n463 = Subtract(x=w1009, y=w1011) -> (x-y=w1010:dbl)
        n464 = Bundle By Name(cluster=w1029, "Recording"=w1025, "Run Profile"=TRUE, "Step Start Time"=w1010, "Last Profile Time"=w1009, "Step Time"=w1013, "Stagger Counter"=0 ("Current Step"), "pb.Run Profile"=w1028) -> (w1047:T25)
        n465 = Insert Into Array(array=w1043, index=0, new element=w1041) -> (w1042:T14[])
      }
      frame "Check Step Time" {
        # "Time elapsed since\nstart of step."
        n466 = Unbundle By Name(w1070) -> ("Step Start Time"=w1073:dbl, "Step Time"=w1071:dbl, "Current Step"=w1068:i32, "App Config.Stagger Time (ms)"=w1053:i32, "Stagger Counter"=w1059:i32)
        n467 = Get Date/Time In Seconds() -> (seconds since 1Jan1904=w1072:timestamp)
        n468 = Increment(x=w1059) -> (x+1=w1054:i32)
        n469 = To Double Precision Float(number=w1072) -> (double precision float=w1067:dbl)
        n470 = Multiply(x=w1053, y=w1054) -> (x*y=w1065:i32)
        n471 = Subtract(x=w1067, y=w1073) -> (x-y=w1064:dbl)
        n472 = To Double Precision Float(number=w1065) -> (double precision float=w1058:dbl)
        n473 = Divide(x=w1058, y=1000.0) -> (x/y=w1056:dbl)
        n474 = Not Equal To 0?(x=w1053) -> (x != 0?=w1052:bool)
        n475 = Greater Or Equal?(x=w1064, y=w1056) -> (x >= y?=w1063:bool)
        n476 = Less Or Equal?(x=w1059, y=4) -> (x <= y?=w1061:bool)
        n477 = Subtract(x=w1071, y=w1064) -> (x-y=w1048:dbl)
        n478 = Compound Arithmetic op=AND(w1063, w1061, w1052) -> (w1060:bool)
        n479 = Less Or Equal To 0?(x=w1048) -> (x <= 0?=w1055:bool)
        n480 = case shown="False" w1055 {
          tunnel: [w1078 w1086] -> w1050
          tunnel: w1068 -> [w1079 w1088]
          tunnel: [w1079 w1087] -> w1049
          tunnel: [w1075 0 ("Stagger Counter")] -> w1066
          tunnel: w1060 -> [w1077 _]
          tunnel: w1059 -> [w1076 _]
          tunnel: w1051 -> [w1074 _]
          frame False {
            # "There's time left.  Update screen."
            n481 = case shown="True" w1077 {
              tunnel: [w1080 w1084] -> w1078
              tunnel: w1076 -> [w1081 w1083]
              tunnel: [w1081 w1082] -> w1075
              tunnel: w1074 -> [w1080 _]
              frame False {
              }
              frame True {
                w1084 = T14[] [enum."Run Step"] items=["Main", "Init Files", "Init", "Unused", "Save As", "Start Profile", "Check Step Time", "Alarm", "Alarm Dismiss", "Run Step", "Stop Profile", "Cycle Reset", "Time Reset", "Time Reset All", "Time Set", "Tare CTs", "Save Profile", "Open Profile", "Get Profiles", "Update Screen", "Update Controls", "Save App Config", "Write Outputs", "Disable Background", "Enable Background", "Get/Release Control", "Log Fuel Change", "Fuel Change Popup", "Read Inputs", "Remote Timer Reset", "Controller Change", "Get Alarms", "Init Alarms", "Save Alarms", "Voltage Selection", "Set Watlow Temp 1", "Set Watlow Temp 2", "Get Pressure", "Write Tare Pressure", "Adjust Controls", "Reinit ADC", "Write Initial Times", "Write Pumps Present", "HMI Command", "Save Pump Times", "Check Pump Stop Time", "Save LS App Config", "Init Data File", "Reset LS Cycles", "Reset Anomalies", "Reset Opens", "Save LS Data", "Save LS Test Data", "Check Serial Numbers", "Main Tab", "Allow Data Note", "Resume Profile"]
                n482 = Increment(x=w1083) -> (x+1=w1082:i32)
              }
            }
          }
          frame True {
            w1086 = T14[] [enum."Run Step"] items=["Main", "Init Files", "Init", "Unused", "Save As", "Start Profile", "Check Step Time", "Alarm", "Alarm Dismiss", "Run Step", "Stop Profile", "Cycle Reset", "Time Reset", "Time Reset All", "Time Set", "Tare CTs", "Save Profile", "Open Profile", "Get Profiles", "Update Screen", "Update Controls", "Save App Config", "Write Outputs", "Disable Background", "Enable Background", "Get/Release Control", "Log Fuel Change", "Fuel Change Popup", "Read Inputs", "Remote Timer Reset", "Controller Change", "Get Alarms", "Init Alarms", "Save Alarms", "Voltage Selection", "Set Watlow Temp 1", "Set Watlow Temp 2", "Get Pressure", "Write Tare Pressure", "Adjust Controls", "Reinit ADC", "Write Initial Times", "Write Pumps Present", "HMI Command", "Save Pump Times", "Check Pump Stop Time", "Save LS App Config", "Init Data File", "Reset LS Cycles", "Reset Anomalies", "Reset Opens", "Save LS Data", "Save LS Test Data", "Check Serial Numbers", "Main Tab", "Allow Data Note", "Resume Profile"]
            # "No time left.  Go to next step."
            n483 = Increment(x=w1088) -> (x+1=w1087:i32)
          }
        }
        n484 = Bundle By Name(cluster=w1070, "Last Profile Time"=w1067, "Step Time Left"=w1048, "New Step"=w1055, "Current Step"=w1049, "Stagger Counter"=w1066) -> (w1069:T25)
      }
      frame "Run Step" {
        w1110 = T14[] [enum."Write Outputs", enum."Read Inputs", enum."Update Screen"] items=["Main", "Init Files", "Init", "Unused", "Save As", "Start Profile", "Check Step Time", "Alarm", "Alarm Dismiss", "Run Step", "Stop Profile", "Cycle Reset", "Time Reset", "Time Reset All", "Time Set", "Tare CTs", "Save Profile", "Open Profile", "Get Profiles", "Update Screen", "Update Controls", "Save App Config", "Write Outputs", "Disable Background", "Enable Background", "Get/Release Control", "Log Fuel Change", "Fuel Change Popup", "Read Inputs", "Remote Timer Reset", "Controller Change", "Get Alarms", "Init Alarms", "Save Alarms", "Voltage Selection", "Set Watlow Temp 1", "Set Watlow Temp 2", "Get Pressure", "Write Tare Pressure", "Adjust Controls", "Reinit ADC", "Write Initial Times", "Write Pumps Present", "HMI Command", "Save Pump Times", "Check Pump Stop Time", "Save LS App Config", "Init Data File", "Reset LS Cycles", "Reset Anomalies", "Reset Opens", "Save LS Data", "Save LS Test Data", "Check Serial Numbers", "Main Tab", "Allow Data Note", "Resume Profile"]
        n485 = Unbundle By Name(w1092) -> ("Profile"=w1122:string[][], "Current Step"=w1121:i32, "# of Steps"=w1120:i32, "App Config.Cycles Completed"=w1119:u32, "App Config.Pumps Present"=w1111:T8, "New Step"=w1126:bool, "Step Start Time"=w1125:dbl)
        n486 = Unbundle By Name(w1092) -> ("Run Profile"=w1091:bool, "LS App Config.Record Bursts"=w1100:bool, "LS App Config.RecInterval(s)"=w1099:i32, "LS App Config.RecDuration(s)"=w1098:i32, "LS App Config.RecFrequeny (Hz)"=w1097:i32, "LS Data Filepath"=w1096:path, "LS App Config.Serial Numbers"=w1094:string[])  [unwired: 1 out]
        n487 = call "Run Step.vi"("Profile"=w1122, "Current Step in"=w1121, "# of Steps"=w1120, "Cycles Completed in"=w1119, "Pumps Present"=w1111) -> ("Bank1State"=w1105:u16, "Bank2State"=w1104:u16, "Record"=w1089:bool, "LS Freq"=w1103:dbl, "LS Duty"=w1102:dbl, "PS Cmd"=w1118:dbl, "Press Cmd"=w1117:dbl, "Ignition Relays"=w1116:T8, "Current Step out"=w1115:i32, "Cycles Completed out"=w1114:u32, "Step Time"=w1113:dbl, "Controller CMDs"=w1112:dbl[], "Power Relays"=w1090:T8)  [unwired: 10 in]
        n488 = Bundle(cluster=T29 {"Running?"=FALSE, "Profile Record"=FALSE, "RecordInterval"=0, "RecordDuration"=0, "RecordFreq"=0, "Data Filepath"=path "", "Hr Record"=FALSE, "Serial Numbers"=[]} ("LS Cluster In"), "Running?"=w1091, "Profile Record"=w1100, "RecordInterval"=w1099, "RecordDuration"=w1098, "RecordFreq"=w1097, "Data Filepath"=w1096, "Hr Record"=w1089, "Serial Numbers"=w1094) -> (w1101:T29)
        n489 = call "LS Data Global.vi"("Mode"=enum16{"Read", "Engine Writes", "Main Writes"}."Main Writes", "LS Cluster In"=w1101) -> ()  [unwired: 11 in, 3 out]
        n490 = local write "Bank 1 Power State:"(w1105) -> ()
        n491 = local write "Bank 2 Power State:"(w1104) -> ()
        n492 = local write "LS Cycle Time (ms):"(w1103) -> ()
        n493 = local write "LS On Time (ms):"(w1102) -> ()
        n494 = case shown="False" w1126 {
          tunnel: [w1136 w1137] -> w1109
          tunnel: w1125 -> [w1136 _]
          tunnel: w1112 -> [_ _]
          frame False {
          }
          frame True {
            n495 = Get Date/Time In Seconds() -> (seconds since 1Jan1904=w1138:timestamp)
            n496 = To Double Precision Float(number=w1138) -> (double precision float=w1137:dbl)
          }
        }
        n497 = Insert Into Array(array=w1123, index=0, new element=w1110) -> (w1108:T14[])
        n498 = flat-sequence {
          tunnel: w1109 -> [_]
          frame #0 {
            n499 = Tick Count (ms)() -> (millisecond timer value=w1135:u32)
            n500 = feedback #3() -> (w1134:u32)  [unwired: 1 in]
            n501 = feedback-in #3(w1135) -> ()
            n502 = Subtract(x=w1135, y=w1134) -> (x-y=→"Run Step (ms)":u32)
          }
        }
        n503 = case shown="True" "Stop Time Enable" {
          tunnel: w1108 -> [w1128 w1130]
          tunnel: [w1128 w1129] -> w1107
          frame False {
          }
          frame True {
            w1132 = T14[] [enum."Check Pump Stop Time"] items=["Main", "Init Files", "Init", "Unused", "Save As", "Start Profile", "Check Step Time", "Alarm", "Alarm Dismiss", "Run Step", "Stop Profile", "Cycle Reset", "Time Reset", "Time Reset All", "Time Set", "Tare CTs", "Save Profile", "Open Profile", "Get Profiles", "Update Screen", "Update Controls", "Save App Config", "Write Outputs", "Disable Background", "Enable Background", "Get/Release Control", "Log Fuel Change", "Fuel Change Popup", "Read Inputs", "Remote Timer Reset", "Controller Change", "Get Alarms", "Init Alarms", "Save Alarms", "Voltage Selection", "Set Watlow Temp 1", "Set Watlow Temp 2", "Get Pressure", "Write Tare Pressure", "Adjust Controls", "Reinit ADC", "Write Initial Times", "Write Pumps Present", "HMI Command", "Save Pump Times", "Check Pump Stop Time", "Save LS App Config", "Init Data File", "Reset LS Cycles", "Reset Anomalies", "Reset Opens", "Save LS Data", "Save LS Test Data", "Check Serial Numbers", "Main Tab", "Allow Data Note", "Resume Profile"]
            n504 = Insert Into Array(array=w1130, index=0, new element=w1132) -> (w1129:T14[])
          }
        }
        n505 = Bundle By Name(cluster=w1092, "Bank 1 State:"=w1105, "Bank 2 State:"=w1104, "LS App Config.LS Power (Freq):"=w1103, "LS App Config.LS Power (Duty):"=w1102, "Tank CMDs.PS CMD"=w1118, "Tank CMDs.Press CMD"=w1117, "Ignition Relay"=w1116, "Current Step"=w1115, "App Config.Cycles Completed"=w1114, "Step Time"=w1113, "Controller CMDs"=w1112, "Power Relay"=w1090, "Step Start Time"=w1109) -> (w1127:T25)
      }
      frame "Write Outputs" {
        w1147 = fxp<+/-,28,17> 0.0 ("Step Threshold")
        w1139 = 40000.0 ("x")
        w1175 = T14[] [] items=["Main", "Init Files", "Init", "Unused", "Save As", "Start Profile", "Check Step Time", "Alarm", "Alarm Dismiss", "Run Step", "Stop Profile", "Cycle Reset", "Time Reset", "Time Reset All", "Time Set", "Tare CTs", "Save Profile", "Open Profile", "Get Profiles", "Update Screen", "Update Controls", "Save App Config", "Write Outputs", "Disable Background", "Enable Background", "Get/Release Control", "Log Fuel Change", "Fuel Change Popup", "Read Inputs", "Remote Timer Reset", "Controller Change", "Get Alarms", "Init Alarms", "Save Alarms", "Voltage Selection", "Set Watlow Temp 1", "Set Watlow Temp 2", "Get Pressure", "Write Tare Pressure", "Adjust Controls", "Reinit ADC", "Write Initial Times", "Write Pumps Present", "HMI Command", "Save Pump Times", "Check Pump Stop Time", "Save LS App Config", "Init Data File", "Reset LS Cycles", "Reset Anomalies", "Reset Opens", "Save LS Data", "Save LS Test Data", "Check Serial Numbers", "Main Tab", "Allow Data Note", "Resume Profile"]
        # "T:Anomalies     F:Opens"
        n506 = Unbundle By Name(w1189) -> ("App Config.Pumps Present"=w1195:T8, "Controller Config.Controller Name"=w1196:T3, "Controller Config.Frequency"=w1194:i32, "Controller CMDs"=w1193:dbl[], "Stagger Counter"=w1192:i32, "App Config.Stagger Time (ms)"=w1191:i32, "Run Profile"=w1190:bool, "Power Relay"=w1180:T8, "Ignition Relay"=w1179:T8, "Tank CMDs"=w1182:T19, "App Config"=w1181:T6, "Voltage Enable"=w1178:bool, "App Config.V_Run PI?"=w1186:bool, "Tank CMDs.PS CMD"=w1184:dbl, "Tank Data.PS Actual (V):"=w1185:dbl, "App Config.VoltCtrlRef"=w1183:string, "LS App Config.Bank 1 Present"=w1174:T2, "LS App Config.Bank 2 Present"=w1173:T1, "LS App Config.DetectionMode"=w1159:i32, "Bank 1 State:"=w1166:u16, "Bank 2 State:"=w1169:u16, "LS App Config.LS Power (Freq):"=w1141:dbl, "LS App Config.LS Power (Duty):"=w1168:dbl, "App Config.Normal Steps:"=w1153:u32, "App Config.Anomaly Threshold:"=w1150:dbl, "App Config.Step Threshold:"=w1151:dbl, "LS App Config.2nd Step Check"=w1146:bool, "LS App Config.Bias Resistances"=w1144:dbl[], "LS App Config.Voltage(T)/Resistance(F)"=w1143:bool)
        n507 = Cluster To Array(cluster=w1174) -> (array=w1162:bool[])
        n508 = Cluster To Array(cluster=w1173) -> (array=w1164:bool[])
        n509 = Equal To 0?(x=w1159) -> (x = 0?=w1158:bool)
        n510 = Multiply(x=w1139, y=w1141) -> (x*y=w1140:dbl)
        n511 = case shown="2" w1166 {
          tunnel: [FALSE FALSE TRUE] -> w1165
          tunnel: [FALSE TRUE FALSE] -> w1154
          frame 0, Default {
            # "Off"
          }
          frame 1 {
            # "On"
          }
          frame 2 {
            # "Pulsing"
          }
        }
        n512 = case shown="2" w1169 {
          tunnel: [FALSE FALSE TRUE] -> w1167
          tunnel: [FALSE TRUE FALSE] -> w1155
          frame 0, Default {
            # "Off"
          }
          frame 1 {
            # "On"
          }
          frame 2 {
            # "Pulsing"
          }
        }
        n513 = disable-structure shown="Enabled" {
          disable-tunnel: w1196 -> [w1228 _]
          disable-tunnel: w1195 -> [w1227 _]
          disable-tunnel: w1194 -> [w1226 _]
          disable-tunnel: w1193 -> [w1225 w1257]
          disable-tunnel: w1192 -> [w1224 _]
          disable-tunnel: w1191 -> [w1223 _]
          disable-tunnel: w1190 -> [w1222 _]
          disable-tunnel: [w1221 w1257] -> w1187
          disable-tunnel: w1186 -> [w1220 _]
          disable-tunnel: w1185 -> [w1219 _]
          disable-tunnel: w1152 -> [w1217 _]
          disable-tunnel: w1184 -> [w1215 _]
          disable-tunnel: w1183 -> [w1214 _]
          disable-tunnel: w1182 -> [w1213 _]
          disable-tunnel: w1181 -> [w1212 _]
          disable-tunnel: w1180 -> [w1211 _]
          disable-tunnel: w1179 -> [w1210 _]
          disable-tunnel: w1178 -> [w1209 _]
          frame Disabled {
            n514 = call "Power Supply Global.vi"("Closed Loop"=w1220, "PS Global Mode"=Power_Supply_Global_Mode."Write Setpoint", "PS Cmd"=w1215, "PS Voltage"=w1219, "VoltCtrlRef"=w1214) -> ()  [unwired: 6 in, 5 out]
            n515 = disable-structure shown="Enabled" {
              disable-tunnel: w1217 -> [w1235 w1236]
              disable-tunnel: [w1234 w1236] -> w1216
              disable-tunnel: w1213 -> [w1233 _]
              disable-tunnel: w1212 -> [w1232 _]
              disable-tunnel: w1211 -> [w1231 _]
              disable-tunnel: w1210 -> [w1230 _]
              disable-tunnel: w1209 -> [w1229 _]
              frame Disabled {
                n516 = call "Write FPGA Outputs.vi"("FPGA Ref"=w1235, "Tank CMDs"=w1233, "App Config"=w1232, "Power Relay"=w1231, "Ignition Relay"=w1230, "Voltage Enable"=w1229) -> ("FPGA Ref OUT"=w1234:T26)  [unwired: 13 in]
              }
              frame Enabled {
              }
            }
            n517 = case shown="\"Kuhnke\", \"Helbako BLDC\", \"PSA\", Default" w1228 {
              selector: w1228 -> [_ w1248]
              tunnel: w1216 -> [w1243 _]
              tunnel: w1227 -> [_ w1252]
              tunnel: w1226 -> [w1242 _]
              tunnel: w1225 -> [w1241 w1250]
              tunnel: w1224 -> [w1240 _]
              tunnel: w1223 -> [w1239 _]
              tunnel: w1222 -> [w1238 _]
              tunnel: [w1237 w1250] -> w1221
              tunnel: w1211 -> [_ w1247]
              tunnel: w1210 -> [_ w1246]
              frame "Kuhnke", "Helbako BLDC", "PSA", Default {
                n518 = call "Write PWM Outputs.vi"("FPGE Ref"=w1243, "Frequency"=w1242, "Controller CMDs IN"=w1241, "Stagger Counter"=w1240, "Stagger Time (ms)"=w1239, "Run Profile"=w1238) -> ("Controller CMDs OUT"=w1237:dbl[])  [unwired: 13 in]
              }
              frame "Conti".."Hella BLDC Pressure" {
                n519 = Cluster To Array(cluster=w1252) -> (array=w1245:bool[])
                n520 = Search 1D Array(1D array=w1245, element=TRUE) -> (index of element=w1251:i32)  [unwired: 1 in]
                n521 = Less Than 0?(x=w1251) -> (x < 0?=w1256:bool)
                n522 = Select(t=0, s=w1256, f=w1251) -> (s? t:f=w1254:i32)
                n523 = Index Array(array=w1250, index=w1254) -> (element=w1244:dbl)
                n524 = call "CAN Global.vi"("Controller Type:"=w1248, "Write (F)"=TRUE, "CAN Cmd"=w1244, "Power Relay"=w1247, "Ignition Relay"=w1246) -> ()  [unwired: 7 in, 4 out]
              }
            }
          }
          frame Enabled {
          }
        }
        n525 = Multiply(x=w1139, y=w1168) -> (x*y=w1172:dbl)
        n526 = To Unsigned Long Integer(number=w1140) -> (unsigned 32bit integer=w1170:u32)
        n527 = To Long Integer(number=w1172) -> (32bit integer=w1171:i32)
        n528 = Insert Into Array(array=w1164, index=0, new element=w1162) -> (w1161:bool[])
        n529 = Not(x=w1158) -> (.not. x?=w1157:bool)
        n530 = And(x=w1161, y=w1158) -> (x .and. y?=w1160:bool[])
        n531 = And(x=w1161, y=w1157) -> (x .and. y?=w1156:bool[])
        n532 = To Fixed-Point(fixed-point type=w1147, number=w1150) -> (fixed-point=w1148:fxp<+/-,28,17>)
        n533 = To Fixed-Point(fixed-point type=w1147, number=w1151) -> (fixed-point=w1149:fxp<+/-,28,17>)
        n534 = xnode "Read/Write Control"("FPGA VI Reference In"=w1152, "Enable Readings"=w1161, "Enable Cycles"=w1160, "Enable Anomalies"=w1160, "Enable Opens"=w1156, "Bank1(Pulse/Const)"=w1165, "Bank1Const(On/Off)"=w1154, "Bank2(Pulse/Const)"=w1167, "Bank2Const(On/Off)"=w1155, "PWM Period (Ticks)"=w1170, "Duty (Ticks)"=w1171, "Normal Steps"=w1153, "Anomaly Threshold"=w1148, "Step Threshold"=w1149, "Enable2ndStepCheck"=w1146, "Subtract Noise"="Subtract Noise", "Resistance In"=w1144, "V(T)/R(F)"=w1143) -> ()  [unwired: 1 in, 2 out]
        n535 = Bundle By Name(cluster=w1189, "Controller CMDs"=w1187) -> (w1188:T25)
        n536 = Insert Into Array(array=w1142, index=0, new element=w1175) -> (w1176:T14[])
      }
      frame "Read Inputs" {
        w1261 = FALSE ("WebDAV Push")
        n537 = Unbundle By Name(w1307) -> ("Concat Data"=w1262:bool, "WebDAV Push"=w1272:bool, "Current Step"=w1271:i32, "Step Time Left"=w1270:dbl, "Run Profile"=w1290:bool, "Controller Config"=w1285:T22, "Trip Counters"=w1300:i32[], "Previous Times"=w1299:u32[], "Prev ON Times"=w1298:u32[], "Alarm Config"=w1301:T10, "Alarm Message 2"=w1294:string, "Alarm Message 1"=w1295:string, "Alarm Latch"=w1296:bool, "App Config.Pumps Present"=w1283:T8, "Power Relay"=w1302:T8, "Controller CMDs"=w1286:dbl[], "App Config"=w1287:T6, "Tank CMDs"=w1288:T19, "Time/Date"=w1291:string, "Run Profile"=w1284:bool, "Recording"=w1293:bool, "Power Relay"=w1289:T8, "App Config.ADC Check"=w1264:bool, "Initial LS Data"=w1259:T15)
        n538 = Cluster To Array(cluster=w1283) -> (array=w1268:bool[])
        n539 = call "Tank Data Global.vi"() -> ("Tank Data OUT"=w1306:dbl[], "Pump Data"=w1274:T17, "Tank Data"=w1273:T23, "Record Time (sec)"=w1263:dbl)  [unwired: 12 in]
        n540 = disable-structure shown="Enabled" {
          disable-tunnel: w1260 -> [w1317 _]
          disable-tunnel: w1288 -> [w1316 _]
          disable-tunnel: w1287 -> [w1315 _]
          disable-tunnel: w1286 -> [w1314 _]
          disable-tunnel: w1285 -> [w1313 _]
          disable-tunnel: w1284 -> [w1312 _]
          disable-tunnel: w1273 -> [w1311 _]
          disable-tunnel: [w1310 _] -> w1269
          disable-tunnel: w1268 -> [w1309 _]
          disable-tunnel: [w1308 _] -> w1266
          frame Disabled {
            n541 = call "Enable Timers.vi"("FPGA Ref"=w1317, "Tank Data"=w1311, "Tank CMDs"=w1316, "App Config"=w1315, "Controller CMDs"=w1314, "Controller Config"=w1313, "Run Profile"=w1312, "Pumps Present"=w1309) -> ("In Spec"=w1310:bool[], "Reset ADCs"=w1308:bool)  [unwired: 18 in]
          }
          frame Enabled {
          }
        }
        n542 = call "Evaluate Alarms.vi"("In Test"=w1290, "Controller"=w1285, "Alarm Config"=w1301, "Data"=w1306, "Pumps Present"=w1268, "Trip Counter"=w1300, "Previous Times"=w1299, "Manual CMDs"=w1286, "Prev ON Times"=w1298) -> ("Trip Counter OUT"=w1305:i32[], "Previous Times OUT"=w1304:u32[], "Alarm Tripped"=w1276:bool, "Prev ON Times OUT"=w1303:u32[], "Alarm Message 1"=w1281:string, "Alarm Message 2"=w1280:string)  [unwired: 13 in]
        n543 = call "RPi HMI Com.vi"("Pump Data"=w1274, "Tank Data"=w1273, "Power Relays"=w1302, "Pump CMDs"=w1286, "App Config"=w1287, "Tank CMDs"=w1288, "Alarm"=w1296, "RPi HMI Mode"=RPi_HMI_Mode."Write Data", "In Test"=w1284, "Alarm Message 1"=w1295, "Controller Config"=w1285, "Alarm Message 2"=w1294, "Recording"=w1293, "Pumps Present"=w1268, "Time/Date"=w1291) -> ()  [unwired: 4 in, 1 out]
        n544 = call "Freeze PID.vi"("Run Profile"=w1284, "Controller CMDs"=w1286, "Controller Config"=w1285, "Power Relay"=w1289) -> ()  [unwired: 12 in]
        n545 = call "Data Logger Global.vi"("WebDAV Push"=w1272, "In Spec"=w1269, "Current Step"=w1271, "Step Time Left"=w1270, "Pump Data"=w1274, "Tank Data"=w1273, "Concat Data"=w1262, "Record Time (sec)"=w1263, "Write (F)"=TRUE) -> ()  [unwired: 3 in, 8 out]
        n546 = call "Get LS Data.vi"("Initial LS Data"=w1259, "FPGA Ref"=w1260) -> ("LS Data"=w1258:T15)  [unwired: 9 in]
        n547 = flat-sequence {
          frame #0 {
            n548 = Tick Count (ms)() -> (millisecond timer value=w1320:u32)
            n549 = feedback #4() -> (w1319:u32)  [unwired: 1 in]
            n550 = feedback-in #4(w1320) -> ()
            n551 = Subtract(x=w1320, y=w1319) -> (x-y=→"Read Inputs (ms)":u32)
          }
        }
        n552 = And(x=w1266, y=w1264) -> (x .and. y?=w1265:bool)
        n553 = case shown="True" w1265 {
          tunnel: w1292 -> [w1326 w1330]
          tunnel: [w1326 w1329] -> w1278
          frame False {
          }
          frame True {
            n554 = Insert Into Array(array=w1330, index=0, new element=Sequence_States."Reinit ADC" ("new element/subarray")) -> (w1329:T14[])
          }
        }
        n555 = Tick Count (ms)() -> (millisecond timer value=w1267:u32)
        n556 = call "Get Time and Date.vi"() -> ("Time/Date"=w1279:string)  [unwired: 11 in]
        n557 = case shown="True" w1276 {
          tunnel: w1278 -> [w1321 w1325]
          tunnel: [w1321 w1324] -> w1277
          frame False {
          }
          frame True {
            w1322 = T14[] [enum."Stop Profile", enum."Update Screen", enum."Disable Background", enum."Alarm"] items=["Main", "Init Files", "Init", "Unused", "Save As", "Start Profile", "Check Step Time", "Alarm", "Alarm Dismiss", "Run Step", "Stop Profile", "Cycle Reset", "Time Reset", "Time Reset All", "Time Set", "Tare CTs", "Save Profile", "Open Profile", "Get Profiles", "Update Screen", "Update Controls", "Save App Config", "Write Outputs", "Disable Background", "Enable Background", "Get/Release Control", "Log Fuel Change", "Fuel Change Popup", "Read Inputs", "Remote Timer Reset", "Controller Change", "Get Alarms", "Init Alarms", "Save Alarms", "Voltage Selection", "Set Watlow Temp 1", "Set Watlow Temp 2", "Get Pressure", "Write Tare Pressure", "Adjust Controls", "Reinit ADC", "Write Initial Times", "Write Pumps Present", "HMI Command", "Save Pump Times", "Check Pump Stop Time", "Save LS App Config", "Init Data File", "Reset LS Cycles", "Reset Anomalies", "Reset Opens", "Save LS Data", "Save LS Test Data", "Check Serial Numbers", "Main Tab", "Allow Data Note", "Resume Profile"]
            n558 = Insert Into Array(array=w1325, index=0, new element=w1322) -> (w1324:T14[])
          }
        }
        n559 = Bundle By Name(cluster=w1307, "Inputs Timer"=w1267, "Pump Data"=w1274, "Tank Data"=w1273, "Trip Counters"=w1305, "Previous Times"=w1304, "Alarm Latch"=w1276, "Prev ON Times"=w1303, "Alarm Message 1"=w1281, "Alarm Message 2"=w1280, "Time/Date"=w1279, "WebDAV Push"=w1261, "Concat Data"=w1261, "LS Data"=w1258) -> (w1282:T25)
      }
      frame "Update Screen" {
        # "Backup current step and time left every ten run minutes and at the start of every new step"
        n560 = Unbundle By Name(w1347) -> ("App Config.Cycles Completed"=→"Cycles Completed:":u32, "Current Step"=w1331:i32, "Step Time Left"=w1332:dbl, "Time/Date"=→"Time/Date":string, "Recording"=→"Recording":bool, "Pump Data"=w1349:T17, "Tank Data"=w1348:T23, "LS Data"=w1344:T15, "Run Profile"=w1354:bool)
        "Step:" <- w1331
        "Time Left:" <- w1332
        n561 = Unbundle(w1349) -> ("Voltages"=→"Voltages":dbl[], "PumpCurrent"=→"PumpCurrent":dbl[], "Speed"=→"Speed":dbl[], "ControllerCurrent"=→"ControllerCurrent":dbl[], "Pressure"=→"Pressure":dbl[], "Flow"=→"Flow":dbl[], "Elapsed Time (Display)"=→"Elapsed Time:":dbl[], "Avg Pressure"=→"Avg Press:":dbl, "Avg Speed"=→"Ave. Speed":dbl)  [unwired: 1 out]
        n562 = Unbundle(w1348) -> ("PS Actual (V):"=→"PS Actual (V):":dbl, "Temp1"=→"Temp1":dbl, "Temp2"=→"Temp2":dbl)
        n563 = Unbundle(w1344) -> ("Total Cycles"=→"Total Cycles":u32[], "Steps"=→"Steps":u32[], "Anomalies Total"=→"Anomalies Total":i32[], "Cycles"=→"Cycles":u32[], "Anomalies/Cycle"=→"Anomalies/Cycle":i32[], "Anomalies (Last Cycle)"=→"Anomalies (Last Cycle)":i32[], "Opens"=→"Opens":i32[])
        n564 = Quotient & Remainder(x=w1332, y=600.0) -> (floor(x/y)=w1334:dbl)  [unwired: 1 out]
        n565 = feedback #5(w1334) -> (w1335:dbl)
        n566 = feedback-in #5(w1334) -> ()
        n567 = Not Equal?(x=w1335, y=w1334) -> (x != y?=w1333:bool)
        n568 = case shown="True" w1333 {
          tunnel: w1332 -> [_ w1371]
          tunnel: w1331 -> [_ w1372]
          frame False {
          }
          frame True {
            n569 = call "Handle Profile Resume Info.vi"("Read(F)/Write(T)"=TRUE ("Write(T)/Read(F)"), "Current Step In"=w1372, "Step Time Left In"=w1371) -> ()  [unwired: 11 in, 2 out]
          }
        }
        n570 = flat-sequence {
          frame #0 {
            n571 = Tick Count (ms)() -> (millisecond timer value=w1375:u32)
            n572 = feedback #6() -> (w1374:u32)  [unwired: 1 in]
            n573 = feedback-in #6(w1375) -> ()
            n574 = Subtract(x=w1375, y=w1374) -> (x-y=→"Update Screen (ms)":u32)
          }
        }
        n575 = case shown="True" w1354 {
          tunnel: [w1376 w1379] -> w1369
          tunnel: w1368 -> [w1376 w1378]
          frame False {
          }
          frame True {
            w1377 = T14[] [enum."Save Pump Times", enum."Update Controls"] items=["Main", "Init Files", "Init", "Unused", "Save As", "Start Profile", "Check Step Time", "Alarm", "Alarm Dismiss", "Run Step", "Stop Profile", "Cycle Reset", "Time Reset", "Time Reset All", "Time Set", "Tare CTs", "Save Profile", "Open Profile", "Get Profiles", "Update Screen", "Update Controls", "Save App Config", "Write Outputs", "Disable Background", "Enable Background", "Get/Release Control", "Log Fuel Change", "Fuel Change Popup", "Read Inputs", "Remote Timer Reset", "Controller Change", "Get Alarms", "Init Alarms", "Save Alarms", "Voltage Selection", "Set Watlow Temp 1", "Set Watlow Temp 2", "Get Pressure", "Write Tare Pressure", "Adjust Controls", "Reinit ADC", "Write Initial Times", "Write Pumps Present", "HMI Command", "Save Pump Times", "Check Pump Stop Time", "Save LS App Config", "Init Data File", "Reset LS Cycles", "Reset Anomalies", "Reset Opens", "Save LS Data", "Save LS Test Data", "Check Serial Numbers", "Main Tab", "Allow Data Note", "Resume Profile"]
            n576 = Insert Into Array(array=w1378, index=0, new element=w1377) -> (w1379:T14[])
          }
        }
        n577 = call "App Global.vi"() -> ("CPU Usage OUT"=→"CPU Usage:":dbl, "Login OUT"=w1350:bool)  [unwired: 9 in, 1 out]
        n578 = Tick Count (ms)() -> (millisecond timer value=w1345:u32)
        n579 = local write "Login"(w1350) -> ()
        n580 = Bundle By Name(cluster=w1347, "Screen Timer"=w1345) -> (w1346:T25)
      }
      frame "Update Controls" {
        w1405 = bool[] [FALSE, FALSE, FALSE, FALSE, FALSE, FALSE] ("pb.Resets")
        w1406 = T14[] [] items=["Main", "Init Files", "Init", "Unused", "Save As", "Start Profile", "Check Step Time", "Alarm", "Alarm Dismiss", "Run Step", "Stop Profile", "Cycle Reset", "Time Reset", "Time Reset All", "Time Set", "Tare CTs", "Save Profile", "Open Profile", "Get Profiles", "Update Screen", "Update Controls", "Save App Config", "Write Outputs", "Disable Background", "Enable Background", "Get/Release Control", "Log Fuel Change", "Fuel Change Popup", "Read Inputs", "Remote Timer Reset", "Controller Change", "Get Alarms", "Init Alarms", "Save Alarms", "Voltage Selection", "Set Watlow Temp 1", "Set Watlow Temp 2", "Get Pressure", "Write Tare Pressure", "Adjust Controls", "Reinit ADC", "Write Initial Times", "Write Pumps Present", "HMI Command", "Save Pump Times", "Check Pump Stop Time", "Save LS App Config", "Init Data File", "Reset LS Cycles", "Reset Anomalies", "Reset Opens", "Save LS Data", "Save LS Test Data", "Check Serial Numbers", "Main Tab", "Allow Data Note", "Resume Profile"]
        n581 = Unbundle By Name(w1408) -> ("App Config.Stagger Time (ms)"=w1417:i32, "Profile"=w1418:string[][], "App Config.Current Profile"=w1413:string, "App Config.CA Number"=w1412:string, "App Config.Controller Type:"=w1419:T3, "App Config.Pumps Present"=w1409:T8, "App Config.Tank 1 Fuel"=w1416:string, "App Config.Tank 2 Fuel"=w1415:string, "App Config.Serial Numbers"=w1414:T40, "App Config.Target Voltage"=w1411:dbl, "App Config.Target Pressure"=w1410:dbl, "Email Alarms Disabled"=w1404:bool, "Run Profile"=w1403:bool, "Recording"=w1402:bool, "Tank CMDs.Press CMD"=w1401:dbl, "Controller CMDs"=w1400:dbl[], "Tank CMDs.PS CMD"=w1399:dbl, "Power Relay"=w1398:T8, "Ignition Relay"=w1383:T8, "WebDAV Push"=w1382:bool, "Concat Data"=w1381:bool, "LS App Config.LS Power (Freq):"=w1387:dbl, "LS App Config.LS Power (Duty):"=w1386:dbl, "LS App Config.Bank 1 Present"=w1385:T2, "LS App Config.Bank 2 Present"=w1384:T1, "LS App Config.Data File Name:"=w1388:string, "LS App Config.Record Bursts"=w1397:bool, "LS App Config.RecInterval(s)"=w1396:i32, "LS App Config.RecDuration(s)"=w1395:i32, "LS App Config.RecFrequeny (Hz)"=w1394:i32, "LS App Config.DetectionMode"=w1393:i32, "LS App Config.Serial Numbers"=w1392:string[], "Bank 1 State:"=w1390:u16, "Bank 2 State:"=w1389:u16)
        n582 = Array To Cluster(array=w1392) -> (cluster=w1391:T48)
        n583 = local write "LS Cycle Time (ms):"(w1387) -> ()
        n584 = local write "LS On Time (ms):"(w1386) -> ()
        n585 = local write "Bank 1"(w1385) -> ()
        n586 = local write "Bank 2"(w1384) -> ()
        n587 = local write "Data File Name:"(w1388) -> ()
        n588 = local write "Record During Profile"(w1397) -> ()
        n589 = local write "Interval Between\nRecordings (s):"(w1396) -> ()
        n590 = local write "Recording\nDuration (s):"(w1395) -> ()
        n591 = local write "Recording\nFrequency (Hz):"(w1394) -> ()
        n592 = local write "Detection Mode:"(w1393) -> ()
        n593 = local write "LS Serial Numbers"(w1391) -> ()
        n594 = local write "Bank 1 Power State:"(w1390) -> ()
        n595 = local write "Bank 2 Power State:"(w1389) -> ()
        n596 = local write "pb.Run Profile"(w1403) -> ()
        n597 = local write "Recording"(w1402) -> ()
        n598 = local write "PressureCMD"(w1401) -> ()
        n599 = local write "Controller\nCMD"(w1400) -> ()
        n600 = local write "Power Supply Cmd:"(w1399) -> ()
        n601 = local write "Power Relay"(w1398) -> ()
        n602 = local write "Ignition Relay"(w1383) -> ()
        n603 = local write "WebDAV Push"(w1382) -> ()
        n604 = local write "Concat Data"(w1381) -> ()
        n605 = local write "pb.Resets"(w1405) -> ()
        n606 = local write "pb.Sets"(w1405) -> ()
        n607 = case shown="False" w1403 {
          tunnel: w1419 -> [w1433 _]
          tunnel: w1418 -> [w1432 _]
          tunnel: w1417 -> [w1431 _]
          tunnel: w1416 -> [w1430 _]
          tunnel: w1415 -> [w1429 _]
          tunnel: w1414 -> [w1428 _]
          tunnel: w1413 -> [w1427 _]
          tunnel: w1412 -> [w1426 _]
          tunnel: w1411 -> [w1425 _]
          tunnel: w1410 -> [w1424 _]
          tunnel: w1409 -> [w1423 _]
          tunnel: w1404 -> [w1422 _]
          frame False {
            n608 = local write "Stagger Time (ms):"(w1431) -> ()
            n609 = local write "Profile:"(w1432) -> ()
            n610 = local write "Profile Name:"(w1427) -> ()
            n611 = local write "CA Number:"(w1426) -> ()
            n612 = local write "Controller Type:"(w1433) -> ()
            n613 = local write "Pumps Present"(w1423) -> ()
            n614 = local write "Tank 1 Fuel Type:"(w1430) -> ()
            n615 = local write "Tank 2 Fuel Type:"(w1429) -> ()
            n616 = local write "Serial Numbers"(w1428) -> ()
            n617 = local write "Target Voltage:"(w1425) -> ()
            n618 = local write "Target Pressure:"(w1424) -> ()
            n619 = local write "Disable Alarm Email"(w1422) -> ()
            "Email Alarms Disabled" <- w1422
          }
          frame True {
          }
        }
        n620 = Insert Into Array(array=w1420, index=0, new element=w1406) -> (w1421:T14[])
      }
      frame "Check Pump Stop Time" {
        n621 = Unbundle By Name(w1443) -> ("Pump Data.Elapsed Time"=w1435:dbl[], "App Config.Pumps Present"=w1437:T8)
        n622 = Cluster To Array(cluster=w1437) -> (array=w1436:bool[])
        n623 = for {
          tunnel: w1436 -> [w1444] mode=indexing
          tunnel: w1435 -> [w1445] mode=indexing
          tunnel: [w1445] -> w1434 mode=indexing if=w1444
        }
        n624 = Array Max & Min(array=w1434) -> (min value=w1442:dbl)  [unwired: 3 out]
        n625 = Greater?(x=w1442, y="Stop Time:") -> (0:w1438:bool)
        n626 = case shown="True" w1438 {
          tunnel: w1440 -> [w1446 w1448]
          tunnel: [w1446 w1447] -> w1439
          frame False {
          }
          frame True {
            w1449 = T14[] [enum."Stop Profile"] items=["Main", "Init Files", "Init", "Unused", "Save As", "Start Profile", "Check Step Time", "Alarm", "Alarm Dismiss", "Run Step", "Stop Profile", "Cycle Reset", "Time Reset", "Time Reset All", "Time Set", "Tare CTs", "Save Profile", "Open Profile", "Get Profiles", "Update Screen", "Update Controls", "Save App Config", "Write Outputs", "Disable Background", "Enable Background", "Get/Release Control", "Log Fuel Change", "Fuel Change Popup", "Read Inputs", "Remote Timer Reset", "Controller Change", "Get Alarms", "Init Alarms", "Save Alarms", "Voltage Selection", "Set Watlow Temp 1", "Set Watlow Temp 2", "Get Pressure", "Write Tare Pressure", "Adjust Controls", "Reinit ADC", "Write Initial Times", "Write Pumps Present", "HMI Command", "Save Pump Times", "Check Pump Stop Time", "Save LS App Config", "Init Data File", "Reset LS Cycles", "Reset Anomalies", "Reset Opens", "Save LS Data", "Save LS Test Data", "Check Serial Numbers", "Main Tab", "Allow Data Note", "Resume Profile"]
            n627 = Insert Into Array(array=w1448, index=0, new element=w1449) -> (w1447:T14[])
          }
        }
      }
      frame "Stop Profile" {
        w1461 = u16 0 items=["0 - Off", "1 - On", "2 - Pulsing"] ("Bank 1 Power State:")
        w1460 = FALSE ("Running?")
        w1472 = T14[] [enum."Write Outputs", enum."Update Controls"] items=["Main", "Init Files", "Init", "Unused", "Save As", "Start Profile", "Check Step Time", "Alarm", "Alarm Dismiss", "Run Step", "Stop Profile", "Cycle Reset", "Time Reset", "Time Reset All", "Time Set", "Tare CTs", "Save Profile", "Open Profile", "Get Profiles", "Update Screen", "Update Controls", "Save App Config", "Write Outputs", "Disable Background", "Enable Background", "Get/Release Control", "Log Fuel Change", "Fuel Change Popup", "Read Inputs", "Remote Timer Reset", "Controller Change", "Get Alarms", "Init Alarms", "Save Alarms", "Voltage Selection", "Set Watlow Temp 1", "Set Watlow Temp 2", "Get Pressure", "Write Tare Pressure", "Adjust Controls", "Reinit ADC", "Write Initial Times", "Write Pumps Present", "HMI Command", "Save Pump Times", "Check Pump Stop Time", "Save LS App Config", "Init Data File", "Reset LS Cycles", "Reset Anomalies", "Reset Opens", "Save LS Data", "Save LS Test Data", "Check Serial Numbers", "Main Tab", "Allow Data Note", "Resume Profile"]
        w1477 = T8 {"Pump 1"=FALSE, "Pump 2"=FALSE, "Pump 3"=FALSE, "Pump 4"=FALSE, "Pump 5"=FALSE, "Pump 6"=FALSE} ("Power Relay")
        n628 = Unbundle By Name(w1476) -> ("Controller Config.Stop Command"=w1475:dbl, "LS App Config.Record Bursts"=w1466:bool, "LS App Config.RecInterval(s)"=w1465:i32, "LS App Config.RecDuration(s)"=w1464:i32, "LS App Config.RecFrequeny (Hz)"=w1463:i32, "LS Data Filepath"=w1462:path, "LS App Config.Record Constant"=w1457:bool, "LS App Config.Serial Numbers"=w1456:string[], "Login"=w1459:bool, "Current Step"=w1452:i32, "Step Time Left"=w1451:dbl)
        n629 = call "Handle Profile Resume Info.vi"("Read(F)/Write(T)"=TRUE, "Current Step In"=w1452, "Step Time Left In"=w1451) -> ()  [unwired: 11 in, 2 out]
        n630 = Bundle(cluster=T29 {"Running?"=FALSE, "Profile Record"=FALSE, "RecordInterval"=0, "RecordDuration"=0, "RecordFreq"=0, "Data Filepath"=path "", "Hr Record"=FALSE, "Serial Numbers"=[]} ("LS Cluster In"), "Running?"=w1460, "Profile Record"=w1466, "RecordInterval"=w1465, "RecordDuration"=w1464, "RecordFreq"=w1463, "Data Filepath"=w1462, "Hr Record"=w1457, "Serial Numbers"=w1456) -> (w1467:T29)
        n631 = call "LS Data Global.vi"("Mode"=enum16{"Read", "Engine Writes", "Main Writes"}."Main Writes", "LS Cluster In"=w1467) -> ()  [unwired: 11 in, 3 out]
        n632 = case shown="True" w1459 {
          frame False {
          }
          frame True {
            w1483 = T30."Enabled" ("Disabled")
            n633 = property on="Bank 1" class="Clust (strict)"("DisabledEnum"=w1483) -> ()  [unwired: 2 in, 2 out]
            n634 = property on="Bank 2" class="Clust (strict)"("DisabledEnum"=w1483) -> ()  [unwired: 2 in, 2 out]
            n635 = property on="Live Data Tab" class="TabCtl (strict)"("DisabledEnum"=w1483) -> ()  [unwired: 2 in, 2 out]
            n636 = property on="Pump Timers Tab" class="TabCtl (strict)"("DisabledEnum"=w1483) -> ()  [unwired: 2 in, 2 out]
          }
        }
        n637 = disable-structure shown="Disabled" {
          frame Disabled {
            n638 = call "Data Logger Main.vi"("Data Logger Mode"=Data_Logger_Mode."Stop") -> ()  [unwired: 19 in]
          }
          frame Enabled {
          }
        }
        n639 = local write "Stop Time Enable"(FALSE ("Stop Time Enable")) -> ()
        n640 = Initialize Array(w1475, 6 ("dimension size")) -> (w1473:dbl[])
        n641 = local write "pb.Pause/Resume"(TRUE) -> ()
        n642 = local write "Bank 1 Power State:"(w1461) -> ()
        n643 = local write "Bank 2 Power State:"(w1461) -> ()
        n644 = Bundle By Name(cluster=w1476, "pb.Run Profile"=w1460, "Run Profile"=FALSE, "Controller CMDs"=w1473, "Power Relay"=w1477, "Ignition Relay"=w1477, "Tank CMDs.Press CMD"=0.0, "Recording"=FALSE, "Bank 1 State:"=w1461, "Bank 2 State:"=w1461) -> (w1470:T25)
        n645 = Insert Into Array(array=w1480, index=0, new element=w1472) -> (w1479:T14[])
      }
      frame "Save As" {
        n646 = property on="Save As Tab" class="TabCtl (strict)"("Visible"=TRUE) -> (error out=w1488:errorcluster)  [unwired: 2 in, 1 out]
        n647 = while {
          tunnel: ["pb.Save As OK"] -> w1494
          tunnel: w1488 -> [_]
          stop <- w1496 stop-if-true
          n648 = Wait (ms)(milliseconds to wait=u32 10) -> ()  [unwired: 1 out]
          n649 = Or(x="pb.Save As OK", y="pb.Save As Cancel") -> (x .or. y?=w1496:bool)
        }
        n650 = Unbundle By Name(w1492) -> ("App Config.Profiles Path"=w1493:path, "Profile"=w1490:string[][])
        n651 = case shown="True" w1494 {
          tunnel: w1493 -> [_ w1504]
          tunnel: [w1499 w1501] -> w1485
          tunnel: w1492 -> [w1500 w1506]
          tunnel: [w1500 w1505] -> w1491
          tunnel: w1490 -> [_ w1503]
          frame False {
            w1499 = T14[] [enum."Enable Background"] items=["Main", "Init Files", "Init", "Unused", "Save As", "Start Profile", "Check Step Time", "Alarm", "Alarm Dismiss", "Run Step", "Stop Profile", "Cycle Reset", "Time Reset", "Time Reset All", "Time Set", "Tare CTs", "Save Profile", "Open Profile", "Get Profiles", "Update Screen", "Update Controls", "Save App Config", "Write Outputs", "Disable Background", "Enable Background", "Get/Release Control", "Log Fuel Change", "Fuel Change Popup", "Read Inputs", "Remote Timer Reset", "Controller Change", "Get Alarms", "Init Alarms", "Save Alarms", "Voltage Selection", "Set Watlow Temp 1", "Set Watlow Temp 2", "Get Pressure", "Write Tare Pressure", "Adjust Controls", "Reinit ADC", "Write Initial Times", "Write Pumps Present", "HMI Command", "Save Pump Times", "Check Pump Stop Time", "Save LS App Config", "Init Data File", "Reset LS Cycles", "Reset Anomalies", "Reset Opens", "Save LS Data", "Save LS Test Data", "Check Serial Numbers", "Main Tab", "Allow Data Note", "Resume Profile"]
          }
          frame True {
            w1501 = T14[] [enum."Enable Background", enum."Get Profiles"] items=["Main", "Init Files", "Init", "Unused", "Save As", "Start Profile", "Check Step Time", "Alarm", "Alarm Dismiss", "Run Step", "Stop Profile", "Cycle Reset", "Time Reset", "Time Reset All", "Time Set", "Tare CTs", "Save Profile", "Open Profile", "Get Profiles", "Update Screen", "Update Controls", "Save App Config", "Write Outputs", "Disable Background", "Enable Background", "Get/Release Control", "Log Fuel Change", "Fuel Change Popup", "Read Inputs", "Remote Timer Reset", "Controller Change", "Get Alarms", "Init Alarms", "Save Alarms", "Voltage Selection", "Set Watlow Temp 1", "Set Watlow Temp 2", "Get Pressure", "Write Tare Pressure", "Adjust Controls", "Reinit ADC", "Write Initial Times", "Write Pumps Present", "HMI Command", "Save Pump Times", "Check Pump Stop Time", "Save LS App Config", "Init Data File", "Reset LS Cycles", "Reset Anomalies", "Reset Opens", "Save LS Data", "Save LS Test Data", "Check Serial Numbers", "Main Tab", "Allow Data Note", "Resume Profile"]
            n652 = call "Save Profile.vi"("Profile"=w1503, "Current Profile"="New Profile Name:", "Profiles Path"=w1504) -> ()  [unwired: 8 in, 1 out]
            n653 = Bundle By Name(cluster=w1506, "App Config.Current Profile"="New Profile Name:") -> (w1505:T25)
          }
        }
        n654 = Insert Into Array(array=w1487, index=0, new element=w1485) -> (w1486:T14[])
      }
      frame "Save App Config" {
        n655 = Unbundle By Name(w1515) -> ("App Config"=w1514:T6)
        n656 = call <vilib>:"Open Config Data.vi"("create file if necessary (T)"=TRUE, "configuration file path"=path "c:/App Config.ini") -> ("error out"=w1508:errorcluster, "refnum"=w1512:T46)  [unwired: 7 in, 1 out]
        n657 = call "Read Write App Config.vi"("Write (F)"=TRUE, "Error IN"=w1508, "App Config"=w1514, "Refnum in"=w1512) -> ("Error OUT"=w1510:errorcluster, "Refnum out"=w1511:T46)  [unwired: 5 in, 1 out]
        n658 = call <vilib>:"Close Config Data.vi"("error in (no error)"=w1510, "refnum"=w1511) -> ()  [unwired: 8 in, 2 out]
      }
      frame "Save LS App Config" {
        n659 = Unbundle By Name(w1544) -> ("LS App Config"=w1526:T13, "pb.Run Profile"=w1537:bool, "LS App Config.Record Bursts"=w1522:bool, "LS App Config.RecInterval(s)"=w1536:i32, "LS App Config.RecDuration(s)"=w1535:i32, "LS App Config.RecFrequeny (Hz)"=w1534:i32, "LS Data Filepath"=w1532:path, "LS App Config.Record Constant"=w1523:bool, "LS App Config.Serial Numbers"=w1527:string[], "App Config.CA Number"=w1525:string, "LS App Config.Data File Name:"=w1524:string)
        n660 = Empty String/Path?(string/path=w1525) -> (empty?=w1530:bool)
        n661 = Empty String/Path?(string/path=w1524) -> (empty?=w1529:bool)
        n662 = call <vilib>:"Open Config Data.vi"("create file if necessary (T)"=TRUE, "configuration file path"=path "c:/LS App Config.ini") -> ("error out"=w1539:errorcluster, "refnum"=w1542:T46)  [unwired: 7 in, 1 out]
        n663 = Bundle By Name(cluster=T29 {"Running?"=FALSE, "Profile Record"=FALSE, "RecordInterval"=0, "RecordDuration"=0, "RecordFreq"=0, "Data Filepath"=path "", "Hr Record"=FALSE, "Serial Numbers"=[]} ("LS Cluster In"), "Running?"=w1537, "Profile Record"=w1522, "RecordInterval"=w1536, "RecordDuration"=w1535, "RecordFreq"=w1534, "Data Filepath"=w1532, "Hr Record"=w1523, "Serial Numbers"=w1527) -> (w1533:T29)
        n664 = Or(x=w1530, y=w1529) -> (x .or. y?=w1528:bool)
        n665 = call "Read Write LS App Config.vi"("Write (F)"=TRUE, "Error IN"=w1539, "LS App Config In"=w1526, "Refnum in"=w1542) -> ("Error OUT"=w1540:errorcluster, "Refnum out"=w1541:T46)  [unwired: 5 in, 1 out]
        n666 = case shown="False" w1528 {
          tunnel: w1523 -> [w1547 _]
          tunnel: w1522 -> [w1548 _]
          tunnel: [w1550 FALSE ("Record During Profile")] -> w1519
          tunnel: [w1549 T30."Disabled and Grayed Out" ("Disabled")] -> w1521
          tunnel: [w1552 FALSE ("Record During Profile")] -> w1518
          tunnel: [w1551 T30."Disabled and Grayed Out" ("Disabled")] -> w1520
          frame False {
            # "Valid file"
            n667 = And(x=w1548, y=w1547) -> (x .and. y?=w1553:bool)
            n668 = case shown="False" w1553 {
              tunnel: [w1554 FALSE] -> w1552
              tunnel: [w1558 T30."Enabled" ("Disabled")] -> w1551
              tunnel: [w1559 FALSE] -> w1550
              tunnel: [w1555 T30."Enabled" ("Disabled")] -> w1549
              tunnel: w1548 -> [w1554 _]
              tunnel: w1547 -> [w1559 _]
              frame False {
                n669 = Select(t=T30."Disabled and Grayed Out" ("Disabled"), s=w1559, f=T30."Enabled" ("Disabled")) -> (s? t:f=w1558:T30)
                n670 = Select(t=T30."Disabled and Grayed Out" ("Disabled"), s=w1554, f=T30."Enabled" ("Disabled")) -> (s? t:f=w1555:T30)
              }
              frame True {
                # "Reset allowing new selection"
                # "Error! - Cannot have both saves active"
              }
            }
          }
          frame True {
            # "Missing Data File Name/CA Number\nCannot Save"
          }
        }
        n671 = call <vilib>:"Close Config Data.vi"("error in (no error)"=w1540, "refnum"=w1541) -> ()  [unwired: 8 in, 2 out]
        n672 = call "LS Data Global.vi"("Mode"=enum16{"Read", "Engine Writes", "Main Writes"}."Main Writes", "LS Cluster In"=w1533) -> ()  [unwired: 11 in, 3 out]
        n673 = property on="Record During Profile" class="Bool (strict)"("Value"=w1518, "DisabledEnum"=w1520) -> ()  [unwired: 2 in, 2 out]
        n674 = property on="Record Constant" class="Bool (strict)"("Value"=w1519, "DisabledEnum"=w1521) -> ()  [unwired: 2 in, 2 out]
      }
      frame "Save Pump Times" {
        n675 = Unbundle By Name(w1574) -> ("Pump Data.Elapsed Time"=w1573:dbl[])
        n676 = Array Size(array=w1573) -> (size(s)=w1572:i32)
        n677 = Equal?(x=w1572, y=6) -> (x = y?=w1570:bool)
        n678 = case shown="True" w1570 {
          tunnel: w1573 -> [_ w1577]
          frame False {
          }
          frame True {
            n679 = Write to Binary File(file (use dialog)=path "c:/ElapsedTimes", data=w1577) -> (refnum out=w1578:refnum<file>, error out=w1579:errorcluster)  [unwired: 4 in, 1 out]
            n680 = Close File(refnum=w1578, error in=w1579) -> ()  [unwired: 2 out]
          }
        }
      }
      frame "Disable Background" {
        w1580 = T30."Disabled and Grayed Out" ("Disabled")
        n681 = property on="Main Tab" class="TabCtl (strict)"("DisabledEnum"=w1580) -> ()  [unwired: 2 in, 2 out]
        n682 = property on="pb.Stop Profile" class="Bool"("DisabledEnum"=w1580) -> ()  [unwired: 2 in, 2 out]
        n683 = property on="Monitoring Tab" class="TabCtl (strict)"("DisabledEnum"=w1580) -> ()  [unwired: 2 in, 2 out]
        n684 = property on="Title Tab" class="TabCtl (strict)"("DisabledEnum"=w1580) -> ()  [unwired: 2 in, 2 out]
        n685 = property on="CPU Usage:" class="DigNum (strict)"("DisabledEnum"=w1580) -> ()  [unwired: 2 in, 2 out]
        n686 = property on="Pump Timers Tab" class="TabCtl (strict)"("DisabledEnum"=w1580) -> ()  [unwired: 2 in, 2 out]
        n687 = property on="Live Data Tab" class="TabCtl (strict)"("DisabledEnum"=w1580) -> ()  [unwired: 2 in, 2 out]
      }
      frame "Enable Background" {
        w1583 = FALSE ("Visible")
        w1584 = T30."Enabled" ("Disabled")
        n688 = disable-structure shown="Enabled" {
          disable-tunnel: w1586 -> [w1589 w1591]
          frame Disabled {
            n689 = xnode "Read/Write Control"("FPGA VI Reference In"=w1589, "Timer Resets"=bool[] [FALSE, FALSE, FALSE, FALSE, FALSE, FALSE] ("array")) -> ()  [unwired: 1 in, 2 out]
          }
          frame Enabled {
            w1590 = bool[] [FALSE, FALSE, FALSE, FALSE, FALSE, FALSE, FALSE, FALSE, FALSE, FALSE, FALSE, FALSE] ("Opens Resets")
            n690 = xnode "Read/Write Control"("FPGA VI Reference In"=w1591, "Opens Resets"=w1590, "Anomaly Resets"=w1590, "Cycle Resets"=w1590) -> ()  [unwired: 1 in, 2 out]
          }
        }
        n691 = property on="Save As Tab" class="TabCtl (strict)"("Visible"=w1583) -> ()  [unwired: 2 in, 2 out]
        n692 = property on="Reset Tab" class="TabCtl (strict)"("Visible"=w1583) -> ()  [unwired: 2 in, 2 out]
        n693 = property on="Set Time Tab" class="TabCtl (strict)"("Visible"=w1583) -> ()  [unwired: 2 in, 2 out]
        n694 = property on="Alarm Tab" class="TabCtl (strict)"("Visible"=w1583) -> ()  [unwired: 2 in, 2 out]
        n695 = property on="Fuel Change Tab" class="TabCtl (strict)"("Visible"=w1583) -> ()  [unwired: 2 in, 2 out]
        n696 = property on="Note Tab" class="TabCtl (strict)"("Visible"=w1583) -> ()  [unwired: 2 in, 2 out]
        n697 = property on="Main Tab" class="TabCtl (strict)"("DisabledEnum"=w1584) -> ()  [unwired: 2 in, 2 out]
        n698 = property on="pb.Stop Profile" class="Bool"("DisabledEnum"=w1584) -> ()  [unwired: 2 in, 2 out]
        n699 = property on="Monitoring Tab" class="TabCtl (strict)"("DisabledEnum"=w1584) -> ()  [unwired: 2 in, 2 out]
        n700 = property on="Title Tab" class="TabCtl (strict)"("DisabledEnum"=w1584) -> ()  [unwired: 2 in, 2 out]
        n701 = property on="CPU Usage:" class="DigNum (strict)"("DisabledEnum"=w1584) -> ()  [unwired: 2 in, 2 out]
        n702 = property on="Alarm Tab" class="TabCtl (strict)"("DisabledEnum"=w1584) -> ()  [unwired: 2 in, 2 out]
        n703 = property on="Pump Timers Tab" class="TabCtl (strict)"("DisabledEnum"=w1584) -> ()  [unwired: 2 in, 2 out]
        n704 = property on="Live Data Tab" class="TabCtl (strict)"("DisabledEnum"=w1584) -> ()  [unwired: 2 in, 2 out]
      }
      frame "Cycle Reset".."Time Reset All", "Reset LS Cycles".."Reset Opens" {
        w1596 = T14[] [enum."Enable Background", enum."Write Initial Times"] items=["Main", "Init Files", "Init", "Unused", "Save As", "Start Profile", "Check Step Time", "Alarm", "Alarm Dismiss", "Run Step", "Stop Profile", "Cycle Reset", "Time Reset", "Time Reset All", "Time Set", "Tare CTs", "Save Profile", "Open Profile", "Get Profiles", "Update Screen", "Update Controls", "Save App Config", "Write Outputs", "Disable Background", "Enable Background", "Get/Release Control", "Log Fuel Change", "Fuel Change Popup", "Read Inputs", "Remote Timer Reset", "Controller Change", "Get Alarms", "Init Alarms", "Save Alarms", "Voltage Selection", "Set Watlow Temp 1", "Set Watlow Temp 2", "Get Pressure", "Write Tare Pressure", "Adjust Controls", "Reinit ADC", "Write Initial Times", "Write Pumps Present", "HMI Command", "Save Pump Times", "Check Pump Stop Time", "Save LS App Config", "Init Data File", "Reset LS Cycles", "Reset Anomalies", "Reset Opens", "Save LS Data", "Save LS Test Data", "Check Serial Numbers", "Main Tab", "Allow Data Note", "Resume Profile"]
        n705 = property on="Reset Tab" class="TabCtl (strict)"("Visible"=TRUE) -> (error out=w1592:errorcluster)  [unwired: 2 in, 1 out]
        n706 = while {
          tunnel: ["pb.Reset OK"] -> w1594
          tunnel: w1592 -> [_]
          stop <- w1671 stop-if-true
          n707 = Wait (ms)(milliseconds to wait=u32 10) -> ()  [unwired: 1 out]
          n708 = Or(x="pb.Reset Cancel", y="pb.Reset OK") -> (x .or. y?=w1671:bool)
        }
        n709 = disable-structure shown="Enabled" {
          disable-tunnel: [w1611 w1641] -> w1602
          disable-tunnel: w1601 -> [w1610 w1639]
          disable-tunnel: w1600 -> [w1609 w1637]
          disable-tunnel: w1599 -> [w1608 w1640]
          disable-tunnel: w1594 -> [w1607 w1638]
          frame Disabled {
            n710 = Unbundle By Name(w1609) -> ("pb.Resets"=w1606:bool[], "Initial Times"=w1603:dbl[])
            n711 = Search 1D Array(1D array=w1606, element=TRUE) -> (index of element=w1604:i32)  [unwired: 1 in]
            n712 = case shown="True" w1607 {
              tunnel: [w1612 w1618] -> w1611
              tunnel: w1609 -> [w1612 w1617]
              tunnel: w1604 -> [_ w1616]
              tunnel: w1603 -> [_ w1615]
              tunnel: w1610 -> [_ w1614]
              tunnel: w1608 -> [_ w1613]
              frame False {
              }
              frame True {
                n713 = case shown="\"Time Reset\"" w1613 {
                  tunnel: w1617 -> [w1621 w1631 w1636]
                  tunnel: [w1620 w1630 w1635] -> w1618
                  tunnel: w1616 -> [_ w1626 _]
                  tunnel: w1615 -> [_ w1629 _]
                  tunnel: w1614 -> [_ w1624 w1634]
                  frame "Cycle Reset", Default {
                    n714 = Bundle By Name(cluster=w1621, "App Config.Cycles Completed"=u32 0) -> (w1620:T25)
                  }
                  frame "Time Reset" {
                    n715 = Replace Array Subset(array=w1629, new element=0.0 ("new element/subarray"), index=w1626) -> (w1622:dbl[])
                    n716 = Replace Array Subset(array=bool[] [FALSE, FALSE, FALSE, FALSE, FALSE, FALSE], new element=TRUE ("new element/subarray"), index=w1626) -> (w1627:bool[])
                    n717 = xnode "Read/Write Control"("FPGA VI Reference In"=w1624, "Timer Resets"=w1627) -> ()  [unwired: 1 in, 2 out]
                    n718 = Bundle By Name(cluster=w1631, "Initial Times"=w1622) -> (w1630:T25)
                  }
                  frame "Time Reset All" {
                    n719 = xnode "Read/Write Control"("FPGA VI Reference In"=w1634, "Timer Resets"=bool[] [TRUE, TRUE, TRUE, TRUE, TRUE, TRUE] ("array")) -> ()  [unwired: 1 in, 2 out]
                    n720 = Bundle By Name(cluster=w1636, "Initial Times"=dbl[] [0.0, 0.0, 0.0, 0.0, 0.0, 0.0] ("Intitial Times")) -> (w1635:T25)
                  }
                }
              }
            }
          }
          frame Enabled {
            n721 = case shown="True" w1638 {
              tunnel: [w1642 w1646] -> w1641
              tunnel: w1637 -> [w1642 w1645]
              tunnel: w1639 -> [_ w1644]
              tunnel: w1640 -> [_ w1643]
              frame False {
              }
              frame True {
                n722 = case shown="\"Reset Opens\"" w1643 {
                  tunnel: w1645 -> [w1650 w1658 w1665 w1669]
                  tunnel: [w1649 w1657 w1664 w1669] -> w1646
                  tunnel: w1644 -> [w1648 w1656 w1663 _]
                  frame "Reset LS Cycles" {
                    n723 = flat-sequence {
                      tunnel: w1648 -> [w1652]
                      frame #0 {
                        n724 = xnode "Read/Write Control"("FPGA VI Reference In"=w1652, "Cycle Resets"=bool[] [TRUE, TRUE, TRUE, TRUE, TRUE, TRUE, TRUE, TRUE, TRUE, TRUE, TRUE, TRUE] ("Opens Resets")) -> ()  [unwired: 1 in, 2 out]
                      }
                      frame #1 {
                        n725 = Wait (ms)(milliseconds to wait=u32 5) -> ()  [unwired: 1 out]
                      }
                    }
                    n726 = Bundle By Name(cluster=w1650, "Initial LS Data.Total Cycles"=u32[] [0, 0, 0, 0, 0, 0, 0, 0, 0, 0, 0, 0]) -> (w1649:T25)
                  }
                  frame "Reset Anomalies" {
                    w1654 = i32[] [0, 0, 0, 0, 0, 0, 0, 0, 0, 0, 0, 0] ("Initial LS Data.Anomalies (Last Cycle)")
                    w1655 = u32[] [0, 0, 0, 0, 0, 0, 0, 0, 0, 0, 0, 0] ("Initial LS Data.Steps")
                    n727 = flat-sequence {
                      tunnel: w1656 -> [w1660]
                      frame #0 {
                        n728 = xnode "Read/Write Control"("FPGA VI Reference In"=w1660, "Anomaly Resets"=bool[] [TRUE, TRUE, TRUE, TRUE, TRUE, TRUE, TRUE, TRUE, TRUE, TRUE, TRUE, TRUE] ("Opens Resets")) -> ()  [unwired: 1 in, 2 out]
                      }
                      frame #1 {
                        n729 = Wait (ms)(milliseconds to wait=u32 5) -> ()  [unwired: 1 out]
                      }
                    }
                    n730 = Bundle By Name(cluster=w1658, "Initial LS Data.Steps"=w1655, "Initial LS Data.Anomalies Total"=w1654, "Initial LS Data.Cycles"=w1655, "Initial LS Data.Anomalies/Cycle"=w1654, "Initial LS Data.Anomalies (Last Cycle)"=w1654) -> (w1657:T25)
                  }
                  frame "Reset Opens" {
                    n731 = flat-sequence {
                      tunnel: w1663 -> [w1667]
                      frame #0 {
                        n732 = xnode "Read/Write Control"("FPGA VI Reference In"=w1667, "Opens Resets"=bool[] [TRUE, TRUE, TRUE, TRUE, TRUE, TRUE, TRUE, TRUE, TRUE, TRUE, TRUE, TRUE]) -> ()  [unwired: 1 in, 2 out]
                      }
                      frame #1 {
                        n733 = Wait (ms)(milliseconds to wait=u32 5) -> ()  [unwired: 1 out]
                      }
                    }
                    n734 = Bundle By Name(cluster=w1665, "Initial LS Data.Opens"=i32[] [0, 0, 0, 0, 0, 0, 0, 0, 0, 0, 0, 0]) -> (w1664:T25)
                  }
                  frame Default {
                  }
                }
              }
            }
          }
        }
        n735 = Insert Into Array(array=w1598, index=0, new element=w1596) -> (w1597:T14[])
      }
      frame "Alarm" {
        w1683 = T14[] [] items=["Main", "Init Files", "Init", "Unused", "Save As", "Start Profile", "Check Step Time", "Alarm", "Alarm Dismiss", "Run Step", "Stop Profile", "Cycle Reset", "Time Reset", "Time Reset All", "Time Set", "Tare CTs", "Save Profile", "Open Profile", "Get Profiles", "Update Screen", "Update Controls", "Save App Config", "Write Outputs", "Disable Background", "Enable Background", "Get/Release Control", "Log Fuel Change", "Fuel Change Popup", "Read Inputs", "Remote Timer Reset", "Controller Change", "Get Alarms", "Init Alarms", "Save Alarms", "Voltage Selection", "Set Watlow Temp 1", "Set Watlow Temp 2", "Get Pressure", "Write Tare Pressure", "Adjust Controls", "Reinit ADC", "Write Initial Times", "Write Pumps Present", "HMI Command", "Save Pump Times", "Check Pump Stop Time", "Save LS App Config", "Init Data File", "Reset LS Cycles", "Reset Anomalies", "Reset Opens", "Save LS Data", "Save LS Test Data", "Check Serial Numbers", "Main Tab", "Allow Data Note", "Resume Profile"]
        n736 = Unbundle By Name(w1674) -> ("Alarm Message 1"=w1679:string, "Alarm Message 2"=w1686:string, "App Config.Location"=w1687:string, "App Config.Email Handler IP"=w1676:string, "Email Alarms Disabled"=w1675:bool)
        n737 = Format Into String(format string="%s\n\n%s", w1679, w1686) -> (resulting string=w1684:string)  [unwired: 2 in, 1 out]
        n738 = Concatenate Strings(w1687, " ALARM!" ("string")) -> (w1685:string)
        n739 = case shown="False" w1675 {
          tunnel: w1685 -> [w1690 _]
          tunnel: w1684 -> [w1689 _]
          tunnel: w1676 -> [w1688 _]
          frame False {
            n740 = flat-sequence {
              tunnel: w1690 -> [w1694]
              tunnel: w1689 -> [w1693]
              tunnel: w1688 -> [w1691]
              frame #0 {
                n741 = call "Email to Handler.vi"("Email Mode"=Email_Mode."Trigger Email", "Email Handler IP"=w1691, "Message:"=w1693, "Subject:"=w1694) -> ()  [unwired: 8 in]
              }
              frame #1 {
                n742 = call "Email Global.vi"("Write (F)"=TRUE, "Send Email"=TRUE) -> ()  [unwired: 9 in, 1 out]
              }
            }
          }
          frame True {
          }
        }
        n743 = flat-sequence {
          tunnel: w1684 -> [w1697]
          frame #0 {
            "Alarm Message" <- w1697
          }
          frame #1 {
            n744 = property on="Alarm Tab" class="TabCtl (strict)"("Visible"=TRUE) -> ()  [unwired: 2 in, 2 out]
          }
        }
        n745 = Insert Into Array(array=w1681, index=0, new element=w1683) -> (w1680:T14[])
      }
      frame "Alarm Dismiss" {
        w1705 = T14[] [enum."Enable Background"] items=["Main", "Init Files", "Init", "Unused", "Save As", "Start Profile", "Check Step Time", "Alarm", "Alarm Dismiss", "Run Step", "Stop Profile", "Cycle Reset", "Time Reset", "Time Reset All", "Time Set", "Tare CTs", "Save Profile", "Open Profile", "Get Profiles", "Update Screen", "Update Controls", "Save App Config", "Write Outputs", "Disable Background", "Enable Background", "Get/Release Control", "Log Fuel Change", "Fuel Change Popup", "Read Inputs", "Remote Timer Reset", "Controller Change", "Get Alarms", "Init Alarms", "Save Alarms", "Voltage Selection", "Set Watlow Temp 1", "Set Watlow Temp 2", "Get Pressure", "Write Tare Pressure", "Adjust Controls", "Reinit ADC", "Write Initial Times", "Write Pumps Present", "HMI Command", "Save Pump Times", "Check Pump Stop Time", "Save LS App Config", "Init Data File", "Reset LS Cycles", "Reset Anomalies", "Reset Opens", "Save LS Data", "Save LS Test Data", "Check Serial Numbers", "Main Tab", "Allow Data Note", "Resume Profile"]
        n746 = Bundle By Name(cluster=w1701, "Alarm Latch"=FALSE) -> (w1700:T25)
        n747 = Insert Into Array(array=w1703, index=0, new element=w1705) -> (w1702:T14[])
      }
      frame "Time Set" {
        w1709 = T14[] [enum."Enable Background", enum."Write Initial Times"] items=["Main", "Init Files", "Init", "Unused", "Save As", "Start Profile", "Check Step Time", "Alarm", "Alarm Dismiss", "Run Step", "Stop Profile", "Cycle Reset", "Time Reset", "Time Reset All", "Time Set", "Tare CTs", "Save Profile", "Open Profile", "Get Profiles", "Update Screen", "Update Controls", "Save App Config", "Write Outputs", "Disable Background", "Enable Background", "Get/Release Control", "Log Fuel Change", "Fuel Change Popup", "Read Inputs", "Remote Timer Reset", "Controller Change", "Get Alarms", "Init Alarms", "Save Alarms", "Voltage Selection", "Set Watlow Temp 1", "Set Watlow Temp 2", "Get Pressure", "Write Tare Pressure", "Adjust Controls", "Reinit ADC", "Write Initial Times", "Write Pumps Present", "HMI Command", "Save Pump Times", "Check Pump Stop Time", "Save LS App Config", "Init Data File", "Reset LS Cycles", "Reset Anomalies", "Reset Opens", "Save LS Data", "Save LS Test Data", "Check Serial Numbers", "Main Tab", "Allow Data Note", "Resume Profile"]
        n748 = disable-structure shown="Disabled" {
          disable-tunnel: [w1723 w1741] -> w1712
          disable-tunnel: w1711 -> [w1722 w1741]
          disable-tunnel: w1710 -> [w1715 _]
          frame Disabled {
            n749 = Unbundle By Name(w1722) -> ("pb.Sets"=w1721:bool[], "Initial Times"=w1716:dbl[], "Pump Data.Elapsed Time"=w1719:dbl[])
            n750 = Search 1D Array(1D array=w1721, element=TRUE) -> (index of element=w1718:i32)  [unwired: 1 in]
            n751 = Index Array(array=w1719, index=w1718) -> (element=w1717:dbl)
            n752 = local write "New Time"(w1717) -> ()
            n753 = property on="Set Time Tab" class="TabCtl (strict)"("Visible"=TRUE) -> (error out=w1713:errorcluster)  [unwired: 2 in, 1 out]
            n754 = while {
              tunnel: ["pb.Set Time OK"] -> w1724
              tunnel: w1717 -> [_]
              tunnel: w1713 -> [_]
              stop <- w1727 stop-if-true
              n755 = Wait (ms)(milliseconds to wait=u32 10) -> ()  [unwired: 1 out]
              n756 = Or(x="pb.Set Time Cancel", y="pb.Set Time OK") -> (x .or. y?=w1727:bool)
            }
            n757 = case shown="True" w1724 {
              tunnel: w1722 -> [w1729 w1735]
              tunnel: [w1729 w1734] -> w1723
              tunnel: w1718 -> [_ w1731]
              tunnel: w1716 -> [_ w1733]
              tunnel: w1715 -> [_ w1732]
              frame False {
              }
              frame True {
                n758 = xnode "Read/Write Control"("FPGA VI Reference In"=w1732) -> ("FPGA VI Reference Out"=w1738:T26, "Timer Resets"=w1739)  [unwired: 1 in, 1 out]
                n759 = Replace Array Subset(array=w1733, new element="New Time", index=w1731) -> (w1740:dbl[])
                n760 = Replace Array Subset(array=w1739, new element=TRUE ("new element/subarray"), index=w1731) -> (w1737:bool[])
                n761 = Bundle By Name(cluster=w1735, "Initial Times"=w1740) -> (w1734:T25)
                n762 = xnode "Read/Write Control"("FPGA VI Reference In"=w1738, "Timer Resets"=w1737) -> ()  [unwired: 1 in, 2 out]
              }
            }
          }
          frame Enabled {
          }
        }
        n763 = Insert Into Array(array=w1707, index=0, new element=w1709) -> (w1706:T14[])
      }
      frame "Remote Timer Reset" {
        w1745 = T14[] [enum."Write Initial Times"] items=["Main", "Init Files", "Init", "Unused", "Save As", "Start Profile", "Check Step Time", "Alarm", "Alarm Dismiss", "Run Step", "Stop Profile", "Cycle Reset", "Time Reset", "Time Reset All", "Time Set", "Tare CTs", "Save Profile", "Open Profile", "Get Profiles", "Update Screen", "Update Controls", "Save App Config", "Write Outputs", "Disable Background", "Enable Background", "Get/Release Control", "Log Fuel Change", "Fuel Change Popup", "Read Inputs", "Remote Timer Reset", "Controller Change", "Get Alarms", "Init Alarms", "Save Alarms", "Voltage Selection", "Set Watlow Temp 1", "Set Watlow Temp 2", "Get Pressure", "Write Tare Pressure", "Adjust Controls", "Reinit ADC", "Write Initial Times", "Write Pumps Present", "HMI Command", "Save Pump Times", "Check Pump Stop Time", "Save LS App Config", "Init Data File", "Reset LS Cycles", "Reset Anomalies", "Reset Opens", "Save LS Data", "Save LS Test Data", "Check Serial Numbers", "Main Tab", "Allow Data Note", "Resume Profile"]
        n764 = disable-structure shown="Disabled" {
          disable-tunnel: w1748 -> [w1754 _]
          frame Disabled {
            n765 = xnode "Read/Write Control"("FPGA VI Reference In"=w1754, "Timer Resets"=bool[] [TRUE, TRUE, TRUE, TRUE, TRUE, TRUE] ("pb.Resets")) -> ("FPGA VI Reference Out"=w1752:T26)  [unwired: 1 in, 1 out]
            n766 = flat-sequence {
              tunnel: w1752 -> [w1755]
              tunnel: [w1755] -> w1751
              frame #0 {
                n767 = Wait (ms)(milliseconds to wait=u32 20) -> ()  [unwired: 1 out]
              }
            }
            n768 = xnode "Read/Write Control"("FPGA VI Reference In"=w1751, "Timer Resets"=bool[] [FALSE, FALSE, FALSE, FALSE, FALSE, FALSE] ("pb.Resets")) -> ()  [unwired: 1 in, 2 out]
          }
          frame Enabled {
          }
        }
        n769 = Bundle By Name(cluster=w1747, "Initial Times"=dbl[] [0.0, 0.0, 0.0, 0.0, 0.0, 0.0] ("Intitial Times")) -> (w1749:T25)
        n770 = Insert Into Array(array=w1742, index=0, new element=w1745) -> (w1743:T14[])
      }
      frame "Get/Release Control" {
        n771 = Unbundle By Name(w1761) -> ("Login"=w1759:bool)
        n772 = case shown="False" w1759 {
          tunnel: [T30."Disabled" ("Disabled") T30."Enabled" ("Disabled")] -> w1757
          frame False {
          }
          frame True {
          }
        }
        n773 = local write "Main Tab"(T9."Main" ("Main Tab")) -> ()
        n774 = property on="Main Tab" class="TabCtl (strict)"("DisabledEnum"=w1757) -> ()  [unwired: 2 in, 2 out]
        n775 = property on="Monitoring Tab" class="TabCtl (strict)"("DisabledEnum"=w1757) -> ()  [unwired: 2 in, 2 out]
        n776 = property on="Bank 1" class="Clust (strict)"("DisabledEnum"=w1757) -> ()  [unwired: 2 in, 2 out]
        n777 = property on="Bank 2" class="Clust (strict)"("DisabledEnum"=w1757) -> ()  [unwired: 2 in, 2 out]
        n778 = property on="Pump Timers Tab" class="TabCtl (strict)"("DisabledEnum"=w1757) -> ()  [unwired: 2 in, 2 out]
        n779 = property on="Live Data Tab" class="TabCtl (strict)"("DisabledEnum"=w1757) -> ()  [unwired: 2 in, 2 out]
        n780 = disable-structure shown="Disabled" {
          disable-tunnel: w1757 -> [w1762 _]
          frame Disabled {
            n781 = property on="pb.Stop Profile" class="Bool"("DisabledEnum"=w1762) -> ()  [unwired: 2 in, 2 out]
          }
          frame Enabled {
          }
        }
      }
      frame "Log Fuel Change" {
        n782 = Get Date/Time In Seconds() -> (seconds since 1Jan1904=w1770:timestamp)
        n783 = Unbundle By Name(w1772) -> ("Fuel Log Path"=w1769:path)
        n784 = Format Date/Time String(seconds (now)=w1770) -> (date/time string=w1768:string)  [unwired: 2 in]
        n785 = Build Array(w1768) -> (w1767:string[])
        n786 = call-poly <vilib>:"Write To Spreadsheet File.vi"("delimiter (\\t)"="," ("delimiter (\\t)"), "append to file? (new file:F)"=TRUE, "1D data"=w1767, "file path (dialog if empty)"=w1769) -> ()  [unwired: 4 in, 1 out]
      }
      frame "Fuel Change Popup" {
        w1773 = T14[] [enum."Enable Background"] items=["Main", "Init Files", "Init", "Unused", "Save As", "Start Profile", "Check Step Time", "Alarm", "Alarm Dismiss", "Run Step", "Stop Profile", "Cycle Reset", "Time Reset", "Time Reset All", "Time Set", "Tare CTs", "Save Profile", "Open Profile", "Get Profiles", "Update Screen", "Update Controls", "Save App Config", "Write Outputs", "Disable Background", "Enable Background", "Get/Release Control", "Log Fuel Change", "Fuel Change Popup", "Read Inputs", "Remote Timer Reset", "Controller Change", "Get Alarms", "Init Alarms", "Save Alarms", "Voltage Selection", "Set Watlow Temp 1", "Set Watlow Temp 2", "Get Pressure", "Write Tare Pressure", "Adjust Controls", "Reinit ADC", "Write Initial Times", "Write Pumps Present", "HMI Command", "Save Pump Times", "Check Pump Stop Time", "Save LS App Config", "Init Data File", "Reset LS Cycles", "Reset Anomalies", "Reset Opens", "Save LS Data", "Save LS Test Data", "Check Serial Numbers", "Main Tab", "Allow Data Note", "Resume Profile"]
        n787 = while {
          stop <- "pb.Fuel Change OK" stop-if-true
          n788 = property on="Fuel Change Tab" class="TabCtl (strict)"("Visible"=TRUE) -> ()  [unwired: 2 in, 2 out]
          n789 = Wait (ms)(milliseconds to wait=u32 20) -> ()  [unwired: 1 out]
        }
        n790 = Insert Into Array(array=w1777, index=0, new element=w1773) -> (w1776:T14[])
      }
      frame "Controller Change" {
        n791 = disable-structure shown="Enabled" {
          disable-tunnel: w1787 -> [w1790 _]
          disable-tunnel: w1786 -> [w1789 w1832]
          disable-tunnel: [w1788 w1832] -> w1785
          frame Disabled {
            n792 = flat-sequence {
              tunnel: [w1795] -> w1792
              tunnel: [w1815] -> w1791
              tunnel: [w1802] -> w1788
              tunnel: w1789 -> [w1803]
              tunnel: w1790 -> [w1810]
              tunnel: w1789 -> [w1814]
              tunnel: w1792 -> [w1831]
              tunnel: w1791 -> [w1824]
              frame #0 {
                w1799 = dbl[] [0.0, 0.0, 0.0, 0.0, 0.0, 0.0] ("ControllerCurrent")
                # "Not updating properly."
                # "Need to write this here as well in case a non-CAN\ncontroller is chosen (otherwise, most recent CAN\ncode will continue to execute)."
                n793 = Unbundle By Name(w1814) -> ("Controller List"=w1796:T24, "App Config.Controller Type:"=w1793:T3)
                n794 = Index Array(array=w1796, index=w1793) -> (element=w1798:T49)
                n795 = Unbundle By Name(w1798) -> ("Frequency"=w1800:i32, "CommSeg"=w1801:i32, "Controller?"=w1815:bool, "High Command"=w1805:dbl, "Low Command"=w1806:dbl, "Command Step"=w1807:dbl, "Invert PWM"=w1797:bool)
                n796 = Equal?(x=1, y=w1801) -> (x = y?=w1795:bool)
                n797 = case shown="False" w1795 {
                  tunnel: [w1819 fxp<+,32,16> 1.0 ("CommFactor")] -> w1812
                  tunnel: w1801 -> [w1820 _]
                  frame False {
                    n798 = case shown="10, Default" w1820 {
                      tunnel: [fxp<+,32,16> 4.0 ("CommFactor") fxp<+,32,16> 5.0 ("CommFactor")] -> w1819
                      frame 8 {
                      }
                      frame 10, Default {
                      }
                    }
                  }
                  frame True {
                  }
                }
                n799 = call "CAN Global.vi"("Controller Type:"=w1793, "Write (F)"=TRUE) -> ()  [unwired: 10 in, 4 out]
                n800 = property on="ControllerCurrent" class="Arr (strict)"("Value"=w1799) -> ()  [unwired: 2 in, 2 out]
                n801 = local write "ControllerCurrent"(w1799) -> ()
                n802 = Divide(x=40000000.0 ("40 MHz"), y=w1800) -> (x/y=w1809:dbl)
                n803 = To Unsigned Long Integer(number=w1809) -> (unsigned 32bit integer=w1804:u32)
                n804 = xnode "Read/Write Control"("FPGA VI Reference In"=w1810, "Brushless"=w1795, "CommFactor"=w1812, "RPMhyst"="RPMhyst", "PWM Period (Ticks)"=w1804, "InvertPWM?"=w1797) -> ()  [unwired: 1 in, 2 out]
                n805 = disable-structure shown="Disabled" {
                  disable-tunnel: w1807 -> [w1818 _]
                  disable-tunnel: w1806 -> [w1817 _]
                  disable-tunnel: w1805 -> [w1816 _]
                  frame Disabled {
                    n806 = property on="Numeric" class="DigNum (strict)"("Maximum"=w1816, "Minimum"=w1817, "Increment"=w1818) -> ()  [unwired: 2 in, 2 out]
                  }
                  frame Enabled {
                  }
                }
                n807 = Bundle By Name(cluster=w1803, "Controller Config"=w1798) -> (w1802:T25)
              }
              frame #1 {
                n808 = Select(t="Pump\nCurrent\n(RMS)" ("Label.Text"), s=w1831, f="Pump\nCurrent\n(DC)" ("Label.Text")) -> (s? t:f=w1826:string)
                n809 = Select(t=T30."Enabled" ("Disabled"), s=w1824, f=T30."Disabled and Grayed Out" ("Disabled")) -> (s? t:f=w1827:T30)
                n810 = property on="PumpCurrent" class="Arr (strict)"("Caption.Text"=w1826) -> ()  [unwired: 2 in, 2 out]
                n811 = property on="ControllerCurrent" class="Arr (strict)"("DisabledEnum"=w1827) -> ()  [unwired: 2 in, 2 out]
              }
            }
          }
          frame Enabled {
          }
        }
        n812 = Insert Into Array(array=w1784, index=0, new element=Sequence_States."Voltage Selection" ("new element/subarray")) -> (w1783:T14[])
      }
      frame "Voltage Selection" {
        # "Delete out controller voltage\nrows to make array correct size"
        n813 = Unbundle By Name(w1842) -> ("Controller Config.Controller?"=w1834:bool, "CalArray"=w1839:dbl[][])
        n814 = Delete From Array(array=w1839, length=6, index (row)=48) -> (deleted portion=w1835:dbl[][], array with subset deleted=w1836:dbl[][])  [unwired: 1 in]
        n815 = case shown="False" w1834 {
          tunnel: w1836 -> [w1846 w1849]
          tunnel: w1835 -> [_ w1848]
          tunnel: [w1846 w1847] -> w1833
          frame False {
            # "Voltage @ Pump\nNo Change"
          }
          frame True {
            # "Switch Voltage\ncoefficients to \nthe controller"
            n816 = for {
              tunnel: w1848 -> [w1852] mode=indexing
              shift-right: [w1851] -> w1847
              shift-left: w1849 -> [w1853]
              i -> [w1850]
              n817 = Replace Array Subset(array=w1853, new element=w1852, index (row)=w1850) -> (w1851:dbl[][])  [unwired: 1 in]
            }
          }
        }
        n818 = Select(t="Controller\nVoltage\n(V)" ("Caption.Text"), s=w1834, f="Pump\nVoltage\n(V)" ("Caption.Text")) -> (s? t:f=w1845:string)
        n819 = property on="Voltages" class="Arr (strict)"("Caption.Text"=w1845) -> ()  [unwired: 2 in, 2 out]
        n820 = call "Tank Data Global.vi"("Pump Data Mode"=Pump_Data_Mode."Write Cal", "Cal Coefficients"=w1833) -> ()  [unwired: 10 in, 4 out]
      }
      frame "Set Watlow Temp 1", "Set Watlow Temp 2" {
        n821 = Unbundle By Name(w1862) -> ("Tank CMDs.Temp 1 CMD"=w1861:dbl, "Tank CMDs.Temp 2 CMD"=w1860:dbl)
        n822 = To Single Precision Float(number=w1861) -> (single precision float=w1859:sgl)
        n823 = To Single Precision Float(number=w1860) -> (single precision float=w1858:sgl)
        n824 = case shown="\"Set Watlow Temp 2\"" w1857 {
          tunnel: [Modbus_Mode."Tank 1 Write" ("Modbus Mode") Modbus_Mode."Tank 2 Write" ("Modbus Mode")] -> w1856
          tunnel: [Modbus_Variable."Setpoint" ("Variable") Modbus_Variable."Setpoint" ("Variable")] -> w1855
          tunnel: [w1864 w1867] -> w1854
          tunnel: w1859 -> [w1864 _]
          tunnel: w1858 -> [_ w1867]
          frame "Set Watlow Temp 1", Default {
          }
          frame "Set Watlow Temp 2" {
          }
        }
        n825 = call "Watlow Modbus.vi"("Modbus Mode"=w1856, "Data Write"=w1854, "Variable"=w1855) -> ()  [unwired: 7 in, 2 out]
      }
      frame "Get Pressure" {
        w1886 = T14[] [enum."Write Tare Pressure"] items=["Main", "Init Files", "Init", "Unused", "Save As", "Start Profile", "Check Step Time", "Alarm", "Alarm Dismiss", "Run Step", "Stop Profile", "Cycle Reset", "Time Reset", "Time Reset All", "Time Set", "Tare CTs", "Save Profile", "Open Profile", "Get Profiles", "Update Screen", "Update Controls", "Save App Config", "Write Outputs", "Disable Background", "Enable Background", "Get/Release Control", "Log Fuel Change", "Fuel Change Popup", "Read Inputs", "Remote Timer Reset", "Controller Change", "Get Alarms", "Init Alarms", "Save Alarms", "Voltage Selection", "Set Watlow Temp 1", "Set Watlow Temp 2", "Get Pressure", "Write Tare Pressure", "Adjust Controls", "Reinit ADC", "Write Initial Times", "Write Pumps Present", "HMI Command", "Save Pump Times", "Check Pump Stop Time", "Save LS App Config", "Init Data File", "Reset LS Cycles", "Reset Anomalies", "Reset Opens", "Save LS Data", "Save LS Test Data", "Check Serial Numbers", "Main Tab", "Allow Data Note", "Resume Profile"]
        n826 = flat-sequence {
          tunnel: [w1890] -> w1878
          frame #0 {
            n827 = call "Tank Data Global.vi"("Pump Data Mode"=Pump_Data_Mode."Write Pressure Offsets", "Pressure Offsets"=dbl[] [0.0, 0.0, 0.0, 0.0, 0.0, 0.0]) -> ()  [unwired: 10 in, 4 out]
          }
          frame #1 {
            # "Wait for write to occur."
            n828 = Wait (ms)(milliseconds to wait=u32 500) -> ()  [unwired: 1 out]
          }
          frame #2 {
            n829 = call "Tank Data Global.vi"("Pump Data Mode"=Pump_Data_Mode."Read") -> ("Tank Data OUT"=w1890:dbl[])  [unwired: 11 in, 3 out]
          }
        }
        n830 = Array Subset(array=w1878, index=30, length=6) -> (w1870:dbl[])
        n831 = Bundle By Name(cluster=w1879, "Pressure Offsets"=w1870) -> (w1880:T25)
        n832 = To Double Precision Float(number=w1870) -> (double precision float=w1875:dbl[])
        n833 = Array To Spreadsheet String(delimiter (Tab)=",", array=w1875, 3:"%.2f" ("format string")) -> (spreadsheet string=w1873:string)
        n834 = Write to Text File(file (use dialog)=path "c:/PressureOffsets", text=w1873) -> (refnum out=w1872:refnum<file>, error out=w1871:errorcluster)  [unwired: 2 in, 1 out]
        n835 = Close File(refnum=w1872, error in=w1871) -> ()  [unwired: 2 out]
        n836 = Insert Into Array(array=w1884, index=0, new element=w1886) -> (w1883:T14[])
      }
      frame "Write Tare Pressure" {
        n837 = Unbundle By Name(w1894) -> ("Pressure Offsets"=w1892:dbl[])
        n838 = call "Tank Data Global.vi"("Pump Data Mode"=Pump_Data_Mode."Write Pressure Offsets", "Pressure Offsets"=w1892) -> ()  [unwired: 10 in, 4 out]
      }
      frame "Adjust Controls" {
        n839 = Unbundle By Name(w1903) -> ("App Config.Voltage Limits"=w1897:T41, "App Config.Voltage Far PI"=w1898:T42, "App Config.Voltage Mid PI"=w1899:T43, "App Config.Voltage Close PI"=w1900:T44, "App Config.Voltage Scale"=w1901:cluster{"V_FFm":dbl, "V_FFb":dbl}, "App Config.Voltage Cutoffs"=w1896:cluster{"V_MidCutoff":dbl, "V_CloseCutoff":dbl})
        n840 = call "PI with FF.vi"("Cutoffs"=w1896, "FFcluster"=w1901, "ClosePIcluster"=w1900, "MidPIcluster"=w1899, "FarPIcluster"=w1898, "LimitCluster"=w1897, "Init (F)"=TRUE) -> ()  [unwired: 8 in, 1 out]
      }
      frame "Reinit ADC" {
        n841 = call "Init FPGA.vi"("FPGA Ref"=w1907) -> ("error out"=w1905:errorcluster, "FPGA Ref Out"=w1906:T26)  [unwired: 9 in]
        n842 = feedback #7(0) -> (w1908:i32)
        "ADC Errors" <- w1908
        n843 = Increment(x=w1908) -> (x+1=w1909:i32)
        n844 = feedback-in #7(w1909) -> ()
        n845 = disable-structure shown="Disabled" {
          disable-tunnel: w1906 -> [w1914 _]
          disable-tunnel: w1905 -> [w1913 _]
          frame Disabled {
            n846 = call "Init ADCs.vi"("Error IN"=w1913, "FPGA Ref"=w1914) -> ()  [unwired: 7 in, 3 out]
          }
          frame Enabled {
          }
        }
      }
      frame "Write Initial Times" {
        w1918 = T14[] [enum."Read Inputs", enum."Save Pump Times"] items=["Main", "Init Files", "Init", "Unused", "Save As", "Start Profile", "Check Step Time", "Alarm", "Alarm Dismiss", "Run Step", "Stop Profile", "Cycle Reset", "Time Reset", "Time Reset All", "Time Set", "Tare CTs", "Save Profile", "Open Profile", "Get Profiles", "Update Screen", "Update Controls", "Save App Config", "Write Outputs", "Disable Background", "Enable Background", "Get/Release Control", "Log Fuel Change", "Fuel Change Popup", "Read Inputs", "Remote Timer Reset", "Controller Change", "Get Alarms", "Init Alarms", "Save Alarms", "Voltage Selection", "Set Watlow Temp 1", "Set Watlow Temp 2", "Get Pressure", "Write Tare Pressure", "Adjust Controls", "Reinit ADC", "Write Initial Times", "Write Pumps Present", "HMI Command", "Save Pump Times", "Check Pump Stop Time", "Save LS App Config", "Init Data File", "Reset LS Cycles", "Reset Anomalies", "Reset Opens", "Save LS Data", "Save LS Test Data", "Check Serial Numbers", "Main Tab", "Allow Data Note", "Resume Profile"]
        n847 = Unbundle By Name(w1920) -> ("Initial Times"=w1919:dbl[])
        n848 = call "Tank Data Global.vi"("Pump Data Mode"=Pump_Data_Mode."Write Initial Times", "Intitial Times"=w1919) -> ()  [unwired: 10 in, 4 out]
        n849 = Insert Into Array(array=w1916, index=0, new element=w1918) -> (w1915:T14[])
      }
      frame "Write Pumps Present" {
        w1937 = T14[] [enum."Write Outputs", enum."Update Controls"] items=["Main", "Init Files", "Init", "Unused", "Save As", "Start Profile", "Check Step Time", "Alarm", "Alarm Dismiss", "Run Step", "Stop Profile", "Cycle Reset", "Time Reset", "Time Reset All", "Time Set", "Tare CTs", "Save Profile", "Open Profile", "Get Profiles", "Update Screen", "Update Controls", "Save App Config", "Write Outputs", "Disable Background", "Enable Background", "Get/Release Control", "Log Fuel Change", "Fuel Change Popup", "Read Inputs", "Remote Timer Reset", "Controller Change", "Get Alarms", "Init Alarms", "Save Alarms", "Voltage Selection", "Set Watlow Temp 1", "Set Watlow Temp 2", "Get Pressure", "Write Tare Pressure", "Adjust Controls", "Reinit ADC", "Write Initial Times", "Write Pumps Present", "HMI Command", "Save Pump Times", "Check Pump Stop Time", "Save LS App Config", "Init Data File", "Reset LS Cycles", "Reset Anomalies", "Reset Opens", "Save LS Data", "Save LS Test Data", "Check Serial Numbers", "Main Tab", "Allow Data Note", "Resume Profile"]
        # "Power and Ignition relays can only turn of if pumps are present."
        n850 = Unbundle By Name(w1926) -> ("App Config.Pumps Present"=w1929:T8, "Power Relay"=w1933:T8, "Ignition Relay"=w1932:T8)
        n851 = Cluster To Array(cluster=w1929) -> (array=w1922:bool[])
        n852 = Cluster To Array(cluster=w1933) -> (array=w1931:bool[])
        n853 = Cluster To Array(cluster=w1932) -> (array=w1930:bool[])
        n854 = call "Tank Data Global.vi"("Pump Data Mode"=Pump_Data_Mode."Write Pumps Present", "Pumps Present"=w1922) -> ()  [unwired: 10 in, 4 out]
        n855 = And(x=w1931, y=w1922) -> (x .and. y?=w1928:bool[])
        n856 = And(x=w1930, y=w1922) -> (x .and. y?=w1927:bool[])
        n857 = Array To Cluster(array=w1928) -> (cluster=w1924:T50)
        n858 = Array To Cluster(array=w1927) -> (cluster=w1923:T50)
        n859 = Bundle By Name(cluster=w1926, "Power Relay"=w1924, "Ignition Relay"=w1923) -> (w1925:T25)
        n860 = Insert Into Array(array=w1935, index=0, new element=w1937) -> (w1934:T14[])
      }
      frame "HMI Command" {
        w1940 = T14[] [] items=["Main", "Init Files", "Init", "Unused", "Save As", "Start Profile", "Check Step Time", "Alarm", "Alarm Dismiss", "Run Step", "Stop Profile", "Cycle Reset", "Time Reset", "Time Reset All", "Time Set", "Tare CTs", "Save Profile", "Open Profile", "Get Profiles", "Update Screen", "Update Controls", "Save App Config", "Write Outputs", "Disable Background", "Enable Background", "Get/Release Control", "Log Fuel Change", "Fuel Change Popup", "Read Inputs", "Remote Timer Reset", "Controller Change", "Get Alarms", "Init Alarms", "Save Alarms", "Voltage Selection", "Set Watlow Temp 1", "Set Watlow Temp 2", "Get Pressure", "Write Tare Pressure", "Adjust Controls", "Reinit ADC", "Write Initial Times", "Write Pumps Present", "HMI Command", "Save Pump Times", "Check Pump Stop Time", "Save LS App Config", "Init Data File", "Reset LS Cycles", "Reset Anomalies", "Reset Opens", "Save LS Data", "Save LS Test Data", "Check Serial Numbers", "Main Tab", "Allow Data Note", "Resume Profile"]
        n861 = flat-sequence {
          tunnel: [w1954] -> w1941
          frame #0 {
            n862 = call "RPi HMI Global.vi"("Mode"=HMI_Global_Mode."Reset Cmd") -> ()  [unwired: 10 in, 1 out]
          }
          frame #1 {
            n863 = call "RPi HMI Global.vi"("Mode"=HMI_Global_Mode."Read") -> ("HMI Cluster OUT"=w1954:T16)  [unwired: 10 in]
          }
        }
        n864 = Unbundle By Name(w1941) -> ("Power Relays"=w1950:T8, "Pump CMDs"=w1949:dbl[], "Tank CMDs.PS CMD"=w1948:dbl, "Tank CMDs.Press CMD"=w1947:dbl, "Tank CMDs.Temp 1 CMD"=w1946:dbl, "Tank CMDs.Temp 2 CMD"=w1945:dbl, "HMI Tog Buttons.Start Test"=w1944:bool)
        n865 = local write "Power Relay"(w1950) -> ()
        n866 = local write "Controller\nCMD"(w1949) -> ()
        n867 = local write "Power Supply Cmd:"(w1948) -> ()
        n868 = local write "PressureCMD"(w1947) -> ()
        n869 = local write "Tank 1 Temp Cmd:"(w1946) -> ()
        n870 = local write "Tank 2 Temp Cmd:"(w1945) -> ()
        n871 = local write "pb.Run Profile"(w1944) -> ()
        n872 = Insert Into Array(array=w1951, index=0, new element=w1940) -> (w1939:T14[])
        n873 = Bundle By Name(cluster=w1943, "HMI"=w1941) -> (w1942:T25)
      }
      frame "Init Data File" {
        n874 = Get Date/Time In Seconds() -> (seconds since 1Jan1904=w1957:timestamp)
        n875 = Unbundle By Name(w1971) -> ("App Config.CA Number"=w1966:string, "LS App Config.Data File Name:"=w1967:string, "LS App Config.Serial Numbers"=w1962:string[])
        n876 = Format Date/Time String(time format string (%c)="_%m%d%y.csv", seconds (now)=w1957) -> (date/time string=w1956:string)  [unwired: 1 in]
        n877 = Empty String/Path?(string/path=w1967) -> (empty?=w1965:bool)
        n878 = Empty String/Path?(string/path=w1966) -> (empty?=w1964:bool)
        n879 = call "Remove illegal file characters.vi"("Filename In"=w1966) -> ("Filename Out"=w1960:string)  [unwired: 10 in]
        n880 = call "Remove illegal file characters.vi"("Filename In"=w1967) -> ("Filename Out"=w1959:string)  [unwired: 10 in]
        n881 = Or(x=w1965, y=w1964) -> (x .or. y?=w1961:bool)
        n882 = Build Path(base path=path "u:/CA Numbers", name or relative path=w1960) -> (appended path=w1968:path)
        n883 = case shown="False" w1961 {
          tunnel: w1968 -> [_ w1978]
          tunnel: w1956 -> [_ w1977]
          tunnel: w1959 -> [_ w1976]
          tunnel: [path "" ("LS Data Filepath") w1975] -> w1963
          tunnel: w1962 -> [_ w1974]
          frame True {
          }
          frame False {
            n884 = disable-structure shown="Enabled" {
              disable-tunnel: w1978 -> [w1991 w2035]
              disable-tunnel: w1977 -> [_ w2030]
              disable-tunnel: w1976 -> [w1979 w2028]
              disable-tunnel: [w1982 w2023] -> w1975
              disable-tunnel: w1974 -> [w1980 w2021]
              frame Enabled {
                n885 = call <vilib>:"Check if File or Folder Exists.vi"("path"=w1991) -> ("error out"=w1988:errorcluster, "file or folder exists?"=w1989:bool, "dup path"=w1990:path)  [unwired: 8 in]
                n886 = case shown="False" w1989 {
                  tunnel: w1990 -> [w2018 w2019]
                  tunnel: w1988 -> [w2015 w2020]
                  tunnel: [w2016 w2020] -> _
                  tunnel: [w2017 w2019] -> w1987
                  frame False {
                    n887 = Create Folder(path (use dialog)=w2018, error in=w2015) -> (created path=w2017:path, error out=w2016:errorcluster)  [unwired: 1 in, 1 out]
                  }
                  frame True {
                  }
                }
                n888 = Build Path(base path=w1987, name or relative path=w1979) -> (appended path=w1986:path)
                n889 = call <vilib>:"Check if File or Folder Exists.vi"("path"=w1986) -> ("error out"=w1983:errorcluster, "file or folder exists?"=w1984:bool, "dup path"=w1985:path)  [unwired: 8 in]
                n890 = disable-structure shown="Enabled" {
                  disable-tunnel: w1985 -> [w1997 w2014]
                  disable-tunnel: w1984 -> [w1996 _]
                  disable-tunnel: w1983 -> [w1995 _]
                  disable-tunnel: [w1994 w2014] -> w1982
                  disable-tunnel: "Timestamp,Pos 1 Voltage,Pos 2 Voltage,Pos 3 Voltage,Pos 4 Voltage,Pos 5 Voltage,Pos 6 Voltage,Pos 7 Voltage,Pos 8 Voltage,Pos 9 Voltage,Pos 10 Voltage,Pos 11 Voltage,Pos 12 Voltage,PS Voltage,Bank 1 State,Bank 2 State\n" -> [w1993 _]
                  disable-tunnel: w1980 -> [w1992 _]
                  frame Disabled {
                    n891 = case shown="False" w1996 {
                      tunnel: w1997 -> [w2012 w2013]
                      tunnel: w1995 -> [w2011 _]
                      tunnel: [w2009 w2013] -> w1994
                      tunnel: w1993 -> [w2003 _]
                      tunnel: w1992 -> [w1999 _]
                      frame False {
                        n892 = Array To Spreadsheet String(delimiter (Tab)=",", array=w1999, 3:"%s" ("format string")) -> (spreadsheet string=w1998:string)
                        n893 = Open/Create/Replace File(file path (use dialog)=w2012, error in=w2011, operation (0:open)=T31."create") -> (refnum out=w2006:refnum<file>, error out=w2008:errorcluster)  [unwired: 3 in, 1 out]
                        n894 = Concatenate Strings("Serial Numbers," ("string"), w1998, w2003) -> (w2002:string)
                        n895 = Write to Text File(file (use dialog)=w2006, text=w2002, error in=w2008) -> (refnum out=w2005:refnum<file>, error out=w2007:errorcluster)  [unwired: 1 in, 1 out]
                        n896 = Close File(refnum=w2005, error in=w2007) -> (path=w2009:path)  [unwired: 1 out]
                      }
                      frame True {
                      }
                    }
                  }
                  frame Enabled {
                  }
                }
              }
              frame Disabled {
                n897 = call <vilib>:"Check if File or Folder Exists.vi"("path"=w2035) -> ("error out"=w2032:errorcluster, "file or folder exists?"=w2033:bool, "dup path"=w2034:path)  [unwired: 8 in]
                n898 = Concatenate Strings(w2028, w2030) -> (w2029:string)
                n899 = case shown="False" w2033 {
                  tunnel: w2034 -> [w2055 w2056]
                  tunnel: w2032 -> [w2052 w2057]
                  tunnel: [w2053 w2057] -> _
                  tunnel: [w2054 w2056] -> w2031
                  frame False {
                    n900 = Create Folder(path (use dialog)=w2055, error in=w2052) -> (created path=w2054:path, error out=w2053:errorcluster)  [unwired: 1 in, 1 out]
                  }
                  frame True {
                  }
                }
                n901 = Build Path(base path=w2031, name or relative path=w2029) -> (appended path=w2027:path)
                n902 = call <vilib>:"Check if File or Folder Exists.vi"("path"=w2027) -> ("error out"=w2024:errorcluster, "file or folder exists?"=w2025:bool, "dup path"=w2026:path)  [unwired: 8 in]
                n903 = case shown="False" w2025 {
                  tunnel: w2026 -> [w2050 w2051]
                  tunnel: w2024 -> [w2049 _]
                  tunnel: [w2047 w2051] -> w2023
                  tunnel: "Timestamp,Pos 1 Voltage,Pos 2 Voltage,Pos 3 Voltage,Pos 4 Voltage,Pos 5 Voltage,Pos 6 Voltage,Pos 7 Voltage,Pos 8 Voltage,Pos 9 Voltage,Pos 10 Voltage,Pos 11 Voltage,Pos 12 Voltage,PS Voltage,Bank 1 State,Bank 2 State\n" -> [w2041 _]
                  tunnel: w2021 -> [w2037 _]
                  frame False {
                    n904 = Array To Spreadsheet String(delimiter (Tab)=",", array=w2037, 3:"%s" ("format string")) -> (spreadsheet string=w2036:string)
                    n905 = Open/Create/Replace File(file path (use dialog)=w2050, error in=w2049, operation (0:open)=T31."create") -> (refnum out=w2044:refnum<file>, error out=w2046:errorcluster)  [unwired: 3 in, 1 out]
                    n906 = Concatenate Strings("Serial Numbers," ("string"), w2036, w2041) -> (w2040:string)
                    n907 = Write to Text File(file (use dialog)=w2044, text=w2040, error in=w2046) -> (refnum out=w2043:refnum<file>, error out=w2045:errorcluster)  [unwired: 1 in, 1 out]
                    n908 = Close File(refnum=w2043, error in=w2045) -> (path=w2047:path)  [unwired: 1 out]
                  }
                  frame True {
                  }
                }
              }
            }
          }
        }
        n909 = local write "CA Number:"(w1960) -> ()
        n910 = local write "Data File Name:"(w1959) -> ()
        n911 = Bundle By Name(cluster=w1971, "App Config.CA Number"=w1960, "LS App Config.Data File Name:"=w1959, "LS Data Filepath"=w1963) -> (w1970:T25)
      }
      frame "Save LS Data" {
        n912 = Unbundle By Name(w2062) -> ("LS Data"=w2060:T15)
        n913 = Unbundle By Name(w2060) -> ("Opens"=w2059:i32[])
        n914 = Array Size(array=w2059) -> (size(s)=w2058:i32)
        n915 = case shown="12" w2058 {
          tunnel: w2060 -> [_ w2065]
          frame Default {
          }
          frame 12 {
            n916 = Write to Binary File(file (use dialog)=path "c:/Monitored Statistics" ("Path"), data=w2065) -> (refnum out=w2064:refnum<file>, error out=w2063:errorcluster)  [unwired: 4 in, 1 out]
            n917 = Close File(refnum=w2064, error in=w2063) -> ()  [unwired: 2 out]
          }
        }
      }
      frame "Save LS Test Data" {
        n918 = Unbundle By Name(w2076) -> ("LS App Config.Serial Numbers"=w2073:string[], "LS Data"=w2074:T15, "App Config.CA Number"=w2068:string, "LS App Config.Data File Name:"=w2069:string, "LS App Config.DetectionMode"=w2075:i32)
        n919 = Empty String/Path?(string/path=w2068) -> (empty?=w2071:bool)
        n920 = Empty String/Path?(string/path=w2069) -> (empty?=w2070:bool)
        n921 = Or(x=w2071, y=w2070) -> (x .or. y?=w2067:bool)
        n922 = case shown="False" w2067 {
          tunnel: w2068 -> [_ w2085]
          tunnel: w2069 -> [_ w2084]
          tunnel: w2075 -> [_ w2080]
          tunnel: w2074 -> [_ w2078]
          tunnel: w2073 -> [_ w2077]
          frame True {
          }
          frame False {
            n923 = Build Path(base path=path "u:/CA Numbers", name or relative path=w2085) -> (appended path=w2082:path)
            n924 = List Folder(path=w2082) -> (filenames=w2083:string[])  [unwired: 3 in, 3 out]
            n925 = while {
              tunnel: w2084 -> [w2128]
              tunnel: [w2126] -> w2081
              shift-right: [w2125] -> _
              shift-left: w2083 -> [w2125]
              i -> [w2130]
              stop <- w2123 stop-if-true
              n926 = Increment(x=w2130) -> (x+1=w2127:i32)
              n927 = Format Into String(format string="%s_Statistics%#f.csv", w2128, w2127) -> (resulting string=w2126:string)  [unwired: 2 in, 1 out]
              n928 = Search 1D Array(1D array=w2125, element=w2126) -> (index of element=w2124:i32)  [unwired: 1 in]
              n929 = Less Than 0?(x=w2124) -> (x < 0?=w2123:bool)
            }
            n930 = Build Path(base path=w2082, name or relative path=w2081) -> (appended path=w2079:path)
            n931 = case shown="1" w2080 {
              tunnel: w2079 -> [_ w2088]
              tunnel: w2078 -> [_ w2121]
              tunnel: w2077 -> [_ w2120]
              frame 0, Default {
                # "Anomalies"
              }
              frame 1 {
                # "Opens"
                n932 = Unbundle By Name(w2121) -> ("Opens"=w2119:i32[])
                n933 = Index Array(array=w2119) -> (element #1=w2106:i32, element #2=w2104:i32, element #3=w2103:i32, element #4=w2102:i32, element #5=w2101:i32, element #6=w2100:i32, element #7=w2099:i32, element #8=w2098:i32, element #9=w2097:i32, element #10=w2096:i32, element #11=w2095:i32, element #12=w2105:i32)  [unwired: 12 in]
                n934 = Index Array(array=w2120) -> (element #1=w2118:string, element #2=w2117:string, element #3=w2116:string, element #4=w2115:string, element #5=w2113:string, element #6=w2114:string, element #7=w2112:string, element #8=w2111:string, element #9=w2109:string, element #10=w2110:string, element #11=w2108:string, element #12=w2107:string)  [unwired: 12 in]
                n935 = Format Into String(format string=",Position 1,Position 2,Position 3,Position 4,Position 5,Position 6,Position 7,Position 8,Position 9,Position 10,Position 11,Position 12\nSerial Numbers,%s,%s,%s,%s,%s,%s,%s,%s,%s,%s,%s,%s\nOpens Detected,%f,%f,%f,%f,%f,%f,%f,%f,%f,%f,%f,%f", w2118, w2117, w2116, w2115, w2113, w2114, w2112, w2111, w2109, w2110, w2108, w2107, w2106, w2104, w2103, w2102, w2101, w2100, w2099, w2098, w2097, w2096, w2095, w2105) -> (resulting string=w2090:string, error out=w2089:errorcluster)  [unwired: 2 in]
                n936 = Open/Create/Replace File(file path (use dialog)=w2088, error in=w2089, operation (0:open)=T31."open or create") -> (refnum out=w2094:refnum<file>, error out=w2092:errorcluster)  [unwired: 3 in, 1 out]
                n937 = Write to Text File(file (use dialog)=w2094, text=w2090, error in=w2092) -> (refnum out=w2093:refnum<file>, error out=w2091:errorcluster)  [unwired: 1 in, 1 out]
                n938 = Close File(refnum=w2093, error in=w2091) -> ()  [unwired: 2 out]
              }
            }
          }
        }
      }
      frame "Check Serial Numbers" {
        n939 = Unbundle By Name(w2136) -> ("LS App Config.Serial Numbers"=w2132:string[])
        n940 = for {
          tunnel: w2132 -> [w2138] mode=indexing
          tunnel: [w2137] -> w2131 mode=indexing
          n941 = call "Remove illegal file characters.vi"("Filename In"=w2138) -> ("Filename Out"=w2137:string)  [unwired: 10 in]
        }
        n942 = Array To Cluster(array=w2131) -> (cluster=w2133:T51)
        n943 = Bundle By Name(cluster=w2136, "LS App Config.Serial Numbers"=w2131) -> (w2135:T25)
        n944 = local write "LS Serial Numbers"(w2133) -> ()
      }
      frame "Main Tab" {
        # "Justin wants Start Test, Stop Test, and Data File Name always unlocked\n\nSo moved Data File Name to where it wouldn't sit on top of another\ncontrol on another page when I made it float like the stop button"
        n945 = Unbundle By Name(w2142) -> ("Main Tab"=w2141:T9)
        n946 = case shown="\"Main\"" w2141 {
          tunnel: [T30."Enabled" ("Disabled") T30."Disabled" ("Disabled")] -> w2140
          tunnel: [TRUE ("Visible") FALSE ("Visible")] -> w2139
          frame "Main" {
          }
          frame Default {
          }
        }
        n947 = property on="pb.Run Profile" class="Bool (strict)"("Visible"=w2139, "DisabledEnum"=w2140) -> ()  [unwired: 2 in, 2 out]
        n948 = property on="Data File Name:" class="Str"("Visible"=w2139, "DisabledEnum"=w2140) -> ()  [unwired: 2 in, 2 out]
      }
      frame "Allow Data Note" {
        w2149 = T14[] [enum."Enable Background"] items=["Main", "Init Files", "Init", "Unused", "Save As", "Start Profile", "Check Step Time", "Alarm", "Alarm Dismiss", "Run Step", "Stop Profile", "Cycle Reset", "Time Reset", "Time Reset All", "Time Set", "Tare CTs", "Save Profile", "Open Profile", "Get Profiles", "Update Screen", "Update Controls", "Save App Config", "Write Outputs", "Disable Background", "Enable Background", "Get/Release Control", "Log Fuel Change", "Fuel Change Popup", "Read Inputs", "Remote Timer Reset", "Controller Change", "Get Alarms", "Init Alarms", "Save Alarms", "Voltage Selection", "Set Watlow Temp 1", "Set Watlow Temp 2", "Get Pressure", "Write Tare Pressure", "Adjust Controls", "Reinit ADC", "Write Initial Times", "Write Pumps Present", "HMI Command", "Save Pump Times", "Check Pump Stop Time", "Save LS App Config", "Init Data File", "Reset LS Cycles", "Reset Anomalies", "Reset Opens", "Save LS Data", "Save LS Test Data", "Check Serial Numbers", "Main Tab", "Allow Data Note", "Resume Profile"]
        n949 = disable-structure shown="Enabled" {
          disable-tunnel: w2148 -> [w2153 _]
          frame Disabled {
            n950 = flat-sequence {
              tunnel: [w2164] -> w2157
              tunnel: [w2163] -> w2156
              tunnel: w2153 -> [w2162]
              tunnel: [w2161] -> w2155
              tunnel: w2157 -> [w2176]
              tunnel: w2156 -> [w2177]
              tunnel: w2155 -> [w2175]
              tunnel: [w2172] -> w2154
              tunnel: w2154 -> [w2193]
              frame #0 {
                w2158 = FALSE ("Visible")
                n951 = property on="Note Tab" class="TabCtl (strict)"("Visible"=TRUE) -> ()  [unwired: 2 in, 2 out]
                n952 = property on="Normal Steps:" class="DigNum (strict)"("Visible"=w2158) -> ()  [unwired: 2 in, 2 out]
                n953 = property on="Step Threshold:" class="DigNum (strict)"("Visible"=w2158) -> ()  [unwired: 2 in, 2 out]
                n954 = property on="Cycle Pts to Avg:" class="DigNum (strict)"("Visible"=w2158) -> ()  [unwired: 2 in, 2 out]
                n955 = property on="Cycle Threshold:" class="DigNum (strict)"("Visible"=w2158) -> ()  [unwired: 2 in, 2 out]
                n956 = property on="pb.Stop Profile" class="Bool"("Visible"=w2158) -> ()  [unwired: 2 in, 2 out]
                n957 = property on="Data File Name:" class="Str"("Visible"=w2158) -> ()  [unwired: 2 in, 2 out]
                n958 = property on="pb.Run Profile" class="Bool (strict)"("Visible"=w2158) -> ()  [unwired: 2 in, 2 out]
                n959 = property on="Anomaly Threshold:" class="DigNum (strict)"("Visible"=w2158) -> ()  [unwired: 2 in, 2 out]
                n960 = property on="Second Step Check" class="Bool (strict)"("Visible"=w2158) -> ()  [unwired: 2 in, 2 out]
                n961 = property on="Main Tab" class="TabCtl (strict)"("DisabledEnum"=T30."Enabled" ("Disabled")) -> ()  [unwired: 2 in, 2 out]
              }
              frame #1 {
                n962 = while {
                  tunnel: ["pb.Note OK"] -> w2166
                  stop <- w2170 stop-if-true
                  n963 = Wait (ms)(milliseconds to wait=u32 10) -> ()  [unwired: 1 out]
                  n964 = local write "Main Tab"(T9."Configure" ("Main Tab")) -> ()
                  n965 = Or(x="pb.Note Cancel", y="pb.Note OK") -> (x .or. y?=w2170:bool)
                }
                n966 = Unbundle By Name(w2162) -> ("Login"=w2161:bool, "LS Data Filepath"=w2163:path, "LS App Config.Record Bursts"=w2165:bool)
                n967 = And(x=w2165, y=w2166) -> (x .and. y?=w2164:bool)
              }
              frame #2 {
                n968 = case shown="True" w2176 {
                  tunnel: w2177 -> [_ w2179]
                  frame False {
                  }
                  frame True {
                    n969 = Open/Create/Replace File(file path (use dialog)=w2179, operation (0:open)=T31."open or create") -> (refnum out=w2187:refnum<file>, error out=w2188:errorcluster)  [unwired: 4 in, 1 out]
                    n970 = Concatenate Strings("Note:,", "Stop Profile Note", "\n") -> (w2180:string)
                    n971 = Set File Position(refnum=w2187, from (0:start)=enum16{"start", "end", "current"}."end", error in=w2188) -> (refnum out=w2191:refnum<file>, error out=w2190:errorcluster)  [unwired: 1 in]
                    n972 = Write to Text File(file (use dialog)=w2191, text=w2180, error in=w2190) -> (refnum out=w2184:refnum<file>, error out=w2183:errorcluster)  [unwired: 1 in, 1 out]
                    n973 = Close File(refnum=w2184, error in=w2183) -> (error out=w2185:errorcluster)  [unwired: 1 out]
                    n974 = call <vilib>:"Clear Errors.vi"("error in (no error)"=w2185) -> ()  [unwired: 6 in, 1 out]
                  }
                }
                n975 = Select(t=T30."Enabled" ("Disabled"), s=w2175, f=T30."Disabled" ("Disabled")) -> (s? t:f=w2172:T30)
              }
              frame #3 {
                w2192 = TRUE ("Visible")
                n976 = local write "Stop Profile Note"("" ("Stop Profile Note")) -> ()
                n977 = local write "Main Tab"(T9."Main" ("Main Tab")) -> ()
                n978 = property on="Main Tab" class="TabCtl (strict)"("DisabledEnum"=w2193) -> ()  [unwired: 2 in, 2 out]
                n979 = property on="Note Tab" class="TabCtl (strict)"("Visible"=FALSE) -> ()  [unwired: 2 in, 2 out]
                n980 = property on="Normal Steps:" class="DigNum (strict)"("Visible"=w2192) -> ()  [unwired: 2 in, 2 out]
                n981 = property on="Step Threshold:" class="DigNum (strict)"("Visible"=w2192) -> ()  [unwired: 2 in, 2 out]
                n982 = property on="Cycle Pts to Avg:" class="DigNum (strict)"("Visible"=w2192) -> ()  [unwired: 2 in, 2 out]
                n983 = property on="Cycle Threshold:" class="DigNum (strict)"("Visible"=w2192) -> ()  [unwired: 2 in, 2 out]
                n984 = property on="pb.Stop Profile" class="Bool"("Visible"=w2192) -> ()  [unwired: 2 in, 2 out]
                n985 = property on="Data File Name:" class="Str"("Visible"=w2192) -> ()  [unwired: 2 in, 2 out]
                n986 = property on="pb.Run Profile" class="Bool (strict)"("Visible"=w2192) -> ()  [unwired: 2 in, 2 out]
                n987 = property on="Anomaly Threshold:" class="DigNum (strict)"("Visible"=w2192) -> ()  [unwired: 2 in, 2 out]
                n988 = property on="Second Step Check" class="Bool (strict)"("Visible"=w2192) -> ()  [unwired: 2 in, 2 out]
              }
            }
          }
          frame Enabled {
          }
        }
        n989 = Insert Into Array(array=w2152, index=0, new element=w2149) -> (w2151:T14[])
      }
    }
  }
  n990 = flat-sequence {
    tunnel: w5 -> [_]
    tunnel: w4 -> [w2197]
    frame #0 {
      n991 = disable-structure shown="Disabled" {
        disable-tunnel: w2197 -> [w2199 _]
        frame Disabled {
          n992 = call "Data Loop.vi"("FPGA Ref"=w2199) -> ()  [unwired: 10 in, 1 out]
        }
        frame Enabled {
        }
      }
      n993 = disable-structure shown="Disabled" {
        disable-tunnel: w2197 -> [w2198 _]
        frame Disabled {
          n994 = call "Power Supply Loop.vi"("FPGA Ref"=w2198) -> ()  [unwired: 11 in]
          n995 = call "Data Logger Loop.vi"() -> ()  [unwired: 20 in]
          n996 = call "CAN Loop.vi"() -> ()  [unwired: 12 in]
        }
        frame Enabled {
        }
      }
      n997 = call "Email Loop.vi"() -> ()  [unwired: 12 in]
      n998 = disable-structure shown="Disabled" {
        frame Disabled {
          n999 = call "Watlow Loop.vi"() -> ()  [unwired: 12 in]
        }
        frame Enabled {
        }
      }
      n1000 = call "App Loop.vi"() -> ()  [unwired: 12 in]
      n1001 = disable-structure shown="Disabled" {
        frame Disabled {
          n1002 = call "RPi HMI Loop.vi"() -> ()  [unwired: 20 in]
        }
        frame Enabled {
        }
      }
      n1003 = call "LS Data Loop.vi"("FPGA Ref"=w2197) -> ()  [unwired: 11 in]
    }
  }
  n1004 = while {
    tunnel: w4 -> [w2202]
    stop <- FALSE stop-if-true
    n1005 = local read "Main Tab"() -> (w2200:T9)
    n1006 = case shown="\"Live Graph\"" w2200 {
      tunnel: w2202 -> [_ w2205]
      frame Default {
        n1007 = Wait (ms)(milliseconds to wait=u32 10) -> ()  [unwired: 1 out]
      }
      frame "Live Graph" {
        n1008 = case shown="False" "Pause" {
          tunnel: w2205 -> [w2214 _]
          frame False {
            n1009 = xnode "Read/Write Control"("FPGA VI Reference In"=w2214) -> ("Anomaly Resamples"=w2208:fxp<+/-,28,17>[])  [unwired: 1 in, 2 out]
            n1010 = Decrement(x="Position") -> (x-1=w2211:i32)
            n1011 = In Range and Coerce(upper limit=9, x=w2211, lower limit=0) -> (coerced(x)=w2207:i32)  [unwired: 1 out]
            n1012 = Index Array(array=w2208, index=w2207) -> (element=→"Waveform Chart":fxp<+/-,28,17>)
            n1013 = Wait (ms)(milliseconds to wait=u32 1) -> ()  [unwired: 1 out]
          }
          frame True {
            n1014 = Wait (ms)(milliseconds to wait=u32 10) -> ()  [unwired: 1 out]
          }
        }
      }
    }
  }
